vi "SentinelController v25.vi"() -> ()   [LabVIEW 2011]
uses:
  <userlib>/configTool/configTool.llb/loadConfigFile.vi
  <userlib>/configTool/configTool.llb/getProperty(STR).vi
  <userlib>/configTool/configTool.llb/initConfigGlobal.vi
  <userlib>/configTool/configTool.llb/closeConfig.vi
  <userlib>/configTool/configTool.llb/getProperty(DBL).vi
  <userlib>/configTool/configTool.llb/getProperty(I32).vi
  <userlib>/configTool/configTool.llb/getProperty(U32).vi
  <userlib>/configTool/configTool.llb/getProperty(BOOL).vi
  SC virtual tester states.ctl
  <vilib>/Instr/_visa.llb/Select Event Type.ctl
  SC virtual handler states.ctl
panel:
  in  "H2 sites ready hidden":string
  out "H2 wt start hidden":u32
  out "H2 wt end hidden":u32
  out "H2 it start hidden":u32
  out "H2 it end hidden":u32
  out "H2 tt start hidden":u32
  out "H2 tt end hidden":u32
  in  "Panels":T1(tab)=enum."System Configuration"
  in  "Test cell ID":string="default"
  in  "Operator name":string="default"
  in  "Lot number":string="default"
  in  "Configuration file path and filename":path
  in  "POWER":bool=TRUE
  in  "H2 allow lower parallelism":bool
  in  "H1 allow lower parallelism":bool
  in  "H1 low yield warning":dbl=95.0 min=0.0 max=100.0 step=1.0
  in  "Ignore alarms until AFTER this many cycles":i32=20
  in  "H1 low yield alarm":dbl=85.0 min=0.0 max=100.0 step=1.0
  in  "H1 low UPH warning (%)":dbl=95.0 min=1.0 max=48000.0 step=1.0
  in  "H1 low UPH alarm (%)":dbl=90.0 min=1.0 max=48000.0 step=1.0
  in  "Enable data logging of all events":bool=TRUE
  in  "Enable electronic notification of alarms":bool
  in  "H2 low UPH alarm (%)":dbl=90.0 min=1.0 max=48000.0 step=1.0
  in  "H2 low UPH warning (%)":dbl=95.0 min=1.0 max=48000.0 step=1.0
  in  "H2 low yield alarm":dbl=90.0 min=0.0 max=100.0 step=1.0
  in  "H2  low yield warning":dbl=95.0 min=0.0 max=100.0 step=1.0
  in  "H1 enable halt\non yield alarm":bool
  in  "H2 enable halt\non yield alarm":bool
  in  "H1 enable halt\non UPH alarm":bool
  in  "H2 enable halt\non UPH alarm":bool
  out "H2 Device Count":u32 caption="Device Count"
  out "H1 Device Count":u32 caption="Decvice Count"
  out "H1 Good Units":u32 caption="Decvice Count"
  out "H2 Good Units":u32 caption="Device Count"
  out "H1 lot yield mon":dbl format="%.1f"
  out "H2 lot yield mon":dbl format="%.1f"
  out "UPH averaging":u32=20 min=2 max=100 step=1
  out "Yield averaging":u32=20 min=2 max=100 step=1
  in  "Push to reset charts":bool
  in  "Run":bool caption="Run / Stop"
  in  "Optimize handler speed":bool
  out "H1 parallelism":u32
  out "Utilization averaging":i32=6 min=2 max=20 step=1
  out "H2 nominal 2":bool=TRUE
  out "H2 warning 2":bool
  out "H2 alarm 2":bool
  out "H1 nominal 2":bool=TRUE
  out "H1 warning 2":bool
  out "H1 alarm 2":bool
  out "H2 nominal":bool=TRUE
  out "H2 warning":bool
  out "H2 alarm":bool
  out "H1 nominal":bool=TRUE
  out "H1 warning":bool
  out "H1 alarm":bool
  out "H2 Lock":bool
  out "H1 Lock":bool
  out "H2 measured Test Time":dbl caption="Index Time" format="%.2f"
  out "H2 measured  Index Time":dbl caption="Index Time" format="%.2f"
  out "H2 Indexing":bool
  out "H2 Testing":bool
  out "H2 Ready with sites":bool
  out "H2 On/Off-line":bool
  out "H2 measured Wait Time":dbl caption="Index Time" format="%.2f"
  out "H1 measured Test Time":dbl caption="Index Time" format="%.2f"
  out "H1 measured Index Time":dbl caption="Index Time" format="%.2f"
  out "H1 Indexing":bool
  out "H1 Testing":bool
  out "H1 Ready with sites":bool
  out "H1 On/Off-line":bool
  out "H1 measured Wait Time":dbl caption="Index Time" format="%.2f"
  out "System UPH":u32(knob) caption="Sys UPH" scale=0.0..30240.0 scale format="%#.0f"
  out "H2 UPH":cluster{u32, u32}(knob) scale=0.0..14400.0 scale format="%#.0f"
  out "H1 UPH":cluster{u32, u32}(knob) scale=0.0..14400.0 scale format="%#.0f"
  out "Sys utilization":dbl(knob) caption="Yield" scale=0.0..100.0
  in  "H2 online":bool=TRUE
  in  "H1 online":bool=TRUE
  in  "Tester online":bool=TRUE
  in  "Alert volume":u32(knob)=5 max=10 step=1 scale=0.0..10.0
  in  "Audio On / Off":bool
  out "SysUtilMon":cluster{i32, i32}(graph)
  out "H2 parallelism":u32 caption="H2 Paralellism"
  out "YieldMon":cluster{i32, i32, i32, i32}(graph)
  out "Program Parallelism":u32=8 caption="Tester Parallelism" min=1 max=16 step=1
  out "H2 calc UPH":dbl format="%#.0f"
  out "H1 Index Time 2":dbl caption="H1 index time"
  out "H1 Test Time 2":dbl caption="H1 test time"
  out "H1 P in formula":u32 caption="H1 Parallelism"
  out "H2 UPH per unit area":dbl format="%.1f"
  out "H1 calc UPH":dbl format="%#.0f"
  out "H1 UPH per unit area":dbl format="%.1f"
  out "Std mo cost ($/mo)":dbl
  out "Std unit cost\n(cents/device)":dbl format="%.3g"
  out "UPH":dbl format="%#.0f"
  in  "Hours per month":i32=730
  out "Std hourly\ncost ($/hr)":dbl format="%.2f"
  in  "Std cell \nfloorspace area":i32=200 min=10 max=1000 step=10
  in  "Overhead ($/mo)":dbl=1000.0 min=0.0 max=10000.0 step=100.0
  in  "Handler cost ($/mo)":dbl=2500.0 min=0.0 max=100000.0 step=100.0
  in  "Tester cost ($/mo)":dbl=8500.0 min=0.0 max=100000.0 step=500.0
  in  "Utilization (%)":u32=80 min=10 max=100 step=10
  out "Calendar days required\nfor testing all units":dbl format="%.1f"
  in  "# of devices to test":u32=10000000 min=1000 max=100000000 step=1000
  out "$ saved":i64 format="%#.0f"
  out "H2 IT (scycle)":dbl format="%.2f"
  out "H2 TT (s/cycle)":dbl format="%.2f"
  out "H2 WT (s/cycle)":dbl format="%.2f"
  out "H1 WT (s/cycle)":dbl format="%.2f"
  out "H1 IT (s/cycle)":dbl format="%.2f"
  out "H1 TT (s/cycle)":dbl format="%.2f"
  out "H2 units/cycle":u32 caption="H1 Parallelism"
  out "H1 units/cycle":u32
  out "Calc H1 UPH":u32
  out "Calc H2 UPH":u32
  out "Std cell floorspace area":i32
  out "Tandem unit cost\n(cents/device)":dbl format="%.3f"
  out "Hours per month 2":i32 caption="Hours per month"
  out "Total Mo Costs ($/mo) 3":dbl caption="Tandem mo cost ($/mo)"
  out "Total Mo Costs ($/mo) 2":dbl caption="Std mo cost ($/mo)"
  out "Calc\nsystem UPH":u32 caption="Simulated\nSystem UPH"
  out "Tandem\nfloorspace area":i32
  out "Tandem UPH\nper unit area":dbl format="%.1f"
  in  "Second handler cost ($/mo)":dbl=2500.0 min=0.0 max=10000.0 step=100.0
  out "Tandem hourly\ncost ($/hr)":dbl format="%.2f"
  in  "Celerint licensing cost ($/mo)":dbl=1000.0 min=0.0 max=10000.0 step=100.0
  in  "Celerint hardware cost ($/mo)":dbl min=0.0 max=10000.0 step=1.0
  in  "Additional floorspace\nfor second handler":i32=50 min=0 max=1000 step=10
  out "Number of text alerts":u32 caption="Number of alerts\nsent as notifications"
  in  "Enable text notification":bool
  out "Notifications Lot Display":string="default" caption="Lot number (not editable)"
  in  "Include\ndata log as\nattachment":bool=TRUE
  out "Number of email alerts":u32 caption="Number of alerts\nsent as notifications"
  out "Email alert - attachment (not editable)":path
  in  "Email alert - message":string="An alarm event has ocurred on a semiconductor test lot that you have requested to monitor.  Please see the attached data log for event details.\n\nThis message is generated automatically by the Sentinel Controller program.\n\nTo stop these messages, please contact the test floor operator and disable automatic alert notifictions.\n\n"
  in  "Email alert - engineer":string="harry@celerint.com"
  in  "Email alert - CC":string="hjr@celerint.com"
  in  "Enable email notification":bool
  in  "Carrier":enum16{"T-Mobile", "AT&T", "Verizon", "Sprint"}(ring)=enum."AT&T"
  in  "Phone number":string="5128263411"
  in  "Subject":string="From: Sentinel Controller"
  in  "Body":string="An alarm event has ocurred"
  in  "GPIB wait time (ms)":u32=1000
  in  "Slow for  Diagnostics":bool
  out "GPIB bus 0 read error":bool
  out "GPIB Bus 0 traffic":string
  out "GPIB bus 1 traffic":string
  out "GPIB bus 2 traffic":string
  out "GPIB bus 0 write error":bool
  out "GPIB bus 1 read error":bool
  out "GPIB bus 1 write error":bool
  out "GPIB bus 2 write error":bool
  out "GPIB bus 2 read error":bool
  out "VISA bus 1 open error":bool
  out "VISA bus 2 open error":bool
  out "VISA bus 0 open error":bool
  out "VISA bus 0 close error":bool
  out "VISA bus 1 close error":bool
  out "VISA bus 2 close error":bool
  out "Decrease Handler Velocity":string
  out "Increase Handler Velocity":string
  out "Get Handler Velocity":string
  in  "SentCtrl listens to tester at":refnum<visa-resource-name>="GPIB0::INTFC"
  out "H2 Address":string
  out "H1 Address":string
  out "Tester address":string
  in  "SentCtrl talks to tester at":refnum<visa-resource-name>="GPIB0::0::INSTR"
  in  "SentCtrl listens to handler 1 at":refnum<visa-resource-name>="GPIB1::INTFC"
  in  "SentCtrl talks to handler 1 at":refnum<visa-resource-name>="GPIB1::1::INSTR"
  in  "SentCtrl listens to handler 2 at":refnum<visa-resource-name>="GPIB2::INTFC"
  in  "SentCtrl talks to handler 2 at":refnum<visa-resource-name>="GPIB2::1::INSTR"
  in  "Ni Logo":bool
  in  "Ni Logo 2":bool
  in  "GPIB wait timeout hid":u32
  out "Number of data log entries hid":u32
  in  "Last locked handler":enum16{"H1", "H2"}(ring)
  out "SC measured wait time hid":dbl
  out "Exit virtual tester H2 state machine hid":bool
  out "Exit virtual tester H1 state machine hid":bool
  out "Exit virtual handler state machine hid":bool
  out "H2 response to *HAND? hidden":string
  out "H1 response to *HAND? hidden":string
  in  "SC virtual tester 2 states":T2
  in  "Tester loop counterhid":u32
  in  "H2 loop counter hid":u32
  in  "H1 loop counter hid":u32
  in  "Test Cycle State hid":T3(ring)
  in  "Test time expected hid":dbl
  out "H1 it end hidden":u32
  out "H1 wt start hidden":u32
  out "H1 tt start hidden":u32
  out "H1 wt end hidden":u32
  out "H1 tt end hidden":u32
  out "H1 it start hidden":u32
  in  "SC virtual tester 1 states":T2
  in  "H1 sites ready hidden":string
  out "VISA bus 1 resource name out":refnum<visa-resource-name>
  out "VISA bus 1 error out":errorcluster
  out "VISA bus 2 error out":errorcluster
  out "VISA bus 2 resource name out":refnum<visa-resource-name>
  out "VISA bus 0 error out":errorcluster
  out "tester wt start hidden":u32
  out "tester wt end hidden":u32
  out "tester tt start hidden":u32
  out "tester tt end hidden":u32
  out "SC measured test time hid":dbl
  in  "Binning_string hidden":string
  out "VISA bus 0 resource name out":refnum<visa-resource-name>
  in  "SC virtual handler states":T4
  out "H1 Single Handler UPH hid":dbl
  out "H1 UPH warning limit hid":dbl
  out "H1 UPH alarm limit hid":dbl
  out "H2 Single Handler UPH hid":dbl
  out "H2 UPH warning limit hid":dbl
  out "H2 UPH alarm limit hid":dbl
  in  "Min Test Time hid":dbl=0.499 caption="Min Test Time" min=0.1 max=1.0 step=0.1 format="%#.1g"
  in  "H2 index time expected hid":dbl
  in  "H1 index time expected hid":dbl
  in  "system states hid":T5(ring)
  in  "system statuts hid":T6(ring)
  out "H1 cycle yield hid":dbl format="%.1f"
  out "H2 cycle yield hid":dbl format="%.1f"
  in  "Data log path and filename":path=path "configuraitons/default_configuraiton.cfg"
  # "Sentinel Controller\nfor\nTandlem Handler\nTest Cells \nwww.celerint.com"
  # "Turning off POWER will stop execution the Sentinel Controller Program"
  # "INPUT FILE"
  # "LOT INFORMATION"
  # "Celerint Sentinel Controller"
  # "SYSTEM PERFORMANCE THRESHOLDS"
  # "Handler  1"
  # "Handler 2"
  # "Set UPH thresholds as % of max UPH"
  # "Set UPH thresholds as % of max UPH"
  # "test cycles (insertions)"
  # "Celerint Sentinel Controller"
  # "Handler 2"
  # "Handler 1"
  # "Yield"
  # "UPH"
  # "Yield"
  # "UPH"
  # "parallelism"
  # "lot yield (%)"
  # "good devices"
  # "devices tested"
  # "Data"
  # "Avg"
  # "wait time"
  # "index time"
  # "test time"
  # "waiting"
  # "H1"
  # "H2"
  # "testing"
  # "indexing"
  # "on/off-line"
  # "STANDARD SETUP"
  # "H2 calculated\nsimilarly"
  # "3600"
  # "Celerint Sentinel\nController Simulator"
  # "TANDEM HANDLER SETUP"
  # "SAVINGS"
  # "3600 (s/hr)"
  # "3600 (s/hr)"
  # "Celerint Sentinel Controller"
  # "Lot number will be appended automatically:"
  # "This data is read from the INI file (.cfg)\nat program start and is used to configure\nthe various GPIB interfaces on the Sentinel\nController."
  # "These setting are created based on the addresses read from the INI file."
  # "Laptop Tester Sim\nGPIB0,SC\naddress 0\nlisten at: GPIB0::INTFC\ntalk to: GPIB0::1::INSTR"
  # "*SITES?"
  # "binning"
  # "Bus 0"
  # "1011"
  # "SC\nGPIB0,Non-SC\naddress 1\nlisten at: GPIB0::INTFC\ntalk to: GPIB0::0::INSTR"
  # "SC\nGPIB1,SC\naddress 0\nlisten at: GPIB1::INTFC\ntalk to: GPIB1::0::INSTR"
  # "SC\nGPIB2,SC\naddress 0\nlisten at: GPIB2::INTFC\ntalk to: GPIB2::0::INSTR"
  # "NI PXI-1031"
  # "*SITES?"
  # "binning"
  # "*SITES?"
  # "binning"
  # "Bus 1"
  # "Bus 2"
  # "1011"
  # "1011"
  # "Laptop H1 Sim\nGPIB1,Non-SC\naddress 1\nlisten at: GPIB1::INTFC\ntalk to: GPIB1::0::INSTR"
  # "Laptop H2 Sim\nGPIB2,Non-SC\naddress 1\nlisten at: GPIB2::INTFC\ntalk to: GPIB2::0::INSTR"
  # "Note:\nUsually, there are default GPIB addresses used for the tester and handler.\nThese addresses are read in from the INI file (.cfrg extension) when this\nprogram initializes.  For the purposes of this map, we are using  these defaults:\n          - Semiconductor tester default GPIB address: 6\n          - Semiconductor handler default GPIB address: 14\nFor the purposes of this illustration, these addresses are purely arbitrary."
  # "Tester\nGPIB0,SC\naddress 6\nlisten at: GPIB0::INTFC\ntalk to: GPIB0:14::INSTR"
  # "*SITES?"
  # "binning"
  # "Bus 0"
  # "1011"
  # "SC\nGPIB0,Non-SC\naddress 14\nlisten at: GPIB1::INTFC\ntalk to: GPIB1:6::INSTR"
  # "SC\nGPIB1,SC\naddress 6\nlisten at: GPIB1::INTFC\ntalk to: GPIB1:14::INSTR"
  # "SC\nGPIB2,SC\naddress 6\nlisten at: GPIB2::INTFC\ntalk to: GPIB2:14::INSTR"
  # "NI PXI-1031"
  # "*SITES?"
  # "binning"
  # "*SITES?"
  # "binning"
  # "Bus 1"
  # "Bus 2"
  # "1011"
  # "1011"
  # "Handler 1\nGPIB0,Non-SC\naddress 14\nlisten at: GPIB0::INTFC\ntalk to: GPIB0:6::INSTR"
  # "Handler 2\nGPIB0,Non-SC\naddress 14\nlisten at: GPIB0::INTFC\ntalk to: GPIB0:6::INSTR"
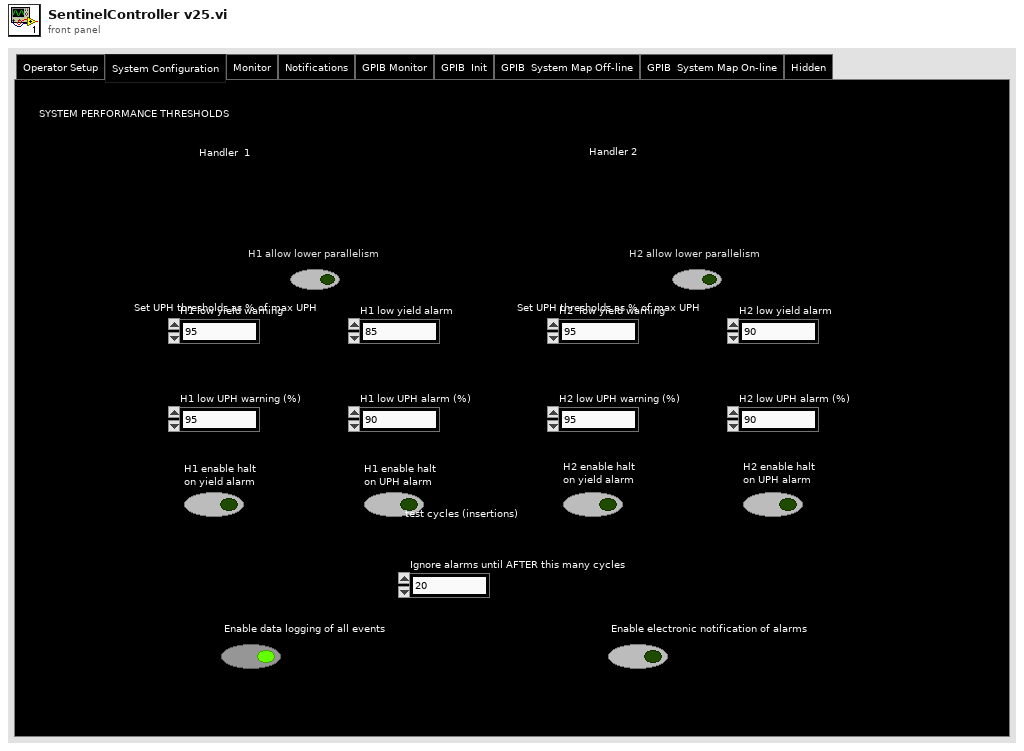
[diagram p1: front panel]
types:
  T1 = enum32{"Operator Setup", "System Configuration", "Monitor", "Benefit Analysis", "Notifications", "GPIB Monitor", "GPIB  Init", "GPIB  System Map Off-line", "GPIB  System Map On-line", "Hidden"}
  T2 = typedef "SC virtual tester states.ctl" = enum16{"initializing bus", "sending *IDN?", "polling SITES?", "sending HAND?", "sending HIDN?", "testing", "binning", "closing bus"}
  T3 = enum16{"idled", "SOT received", "SOT sent", "binning sent", "binning received", "sites ready received", "sites ready sent"}
  T4 = typedef "SC virtual handler states.ctl" = enum16{"initializing bus", "waiting on event", "reading", "responding to *IDN?", "responding to FR?", "responding to *STB?", "responding to *SITES?", "ressponding to FULLSITES?", "responding to *HIDN?", "respond to *HAND?", "testing", "responding to BINON", "responding to A BIN", "responding to ECHOOK", "responding to ECHONG", "indexing", "responding to unknown command", "closing bus"}
  T5 = enum16{"H1 Ready", "H2 Ready", "No Handler Ready"}
  T6 = enum16{"H1NH2N", "H1NH2W", "H1NH2A", "H1WH2N", "H1WH2W", "H1WH2A", "H1AH2N", "H1AH2W", "H1AH2A"}
  T7 = enum16{"open", "replace", "create", "open or create", "replace or create", "replace or create with confirmation"}
  T8 = typedef "configRef.ctl" = refnum<vi>
  T9 = cluster{i32, "rolling avg out":dbl, "H1 low yield alarm":dbl, "H2 low yield alarm":dbl}
  T10 = cluster{"rolling avg out":dbl, i32, "H1 low yield alarm":dbl, "H2 low yield alarm":dbl}
  T11 = typedef "Select Event Type.ctl" = u32
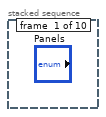
[diagram p2: hidden frame]
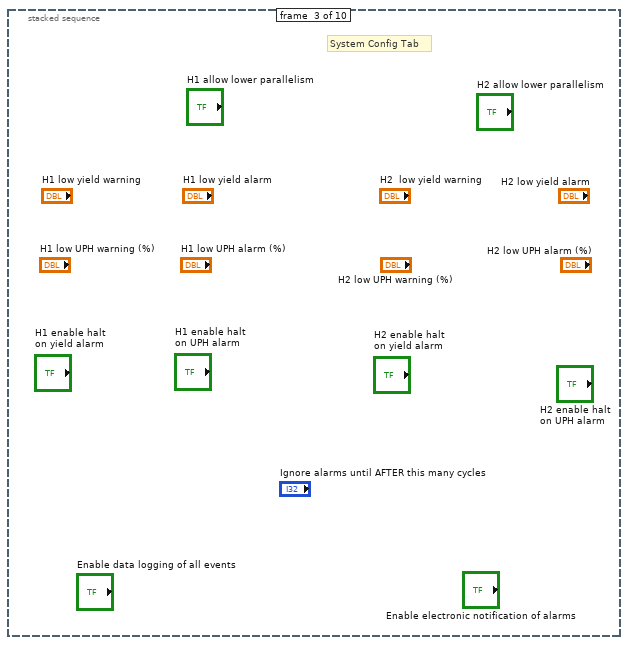
[diagram p3: hidden frame]
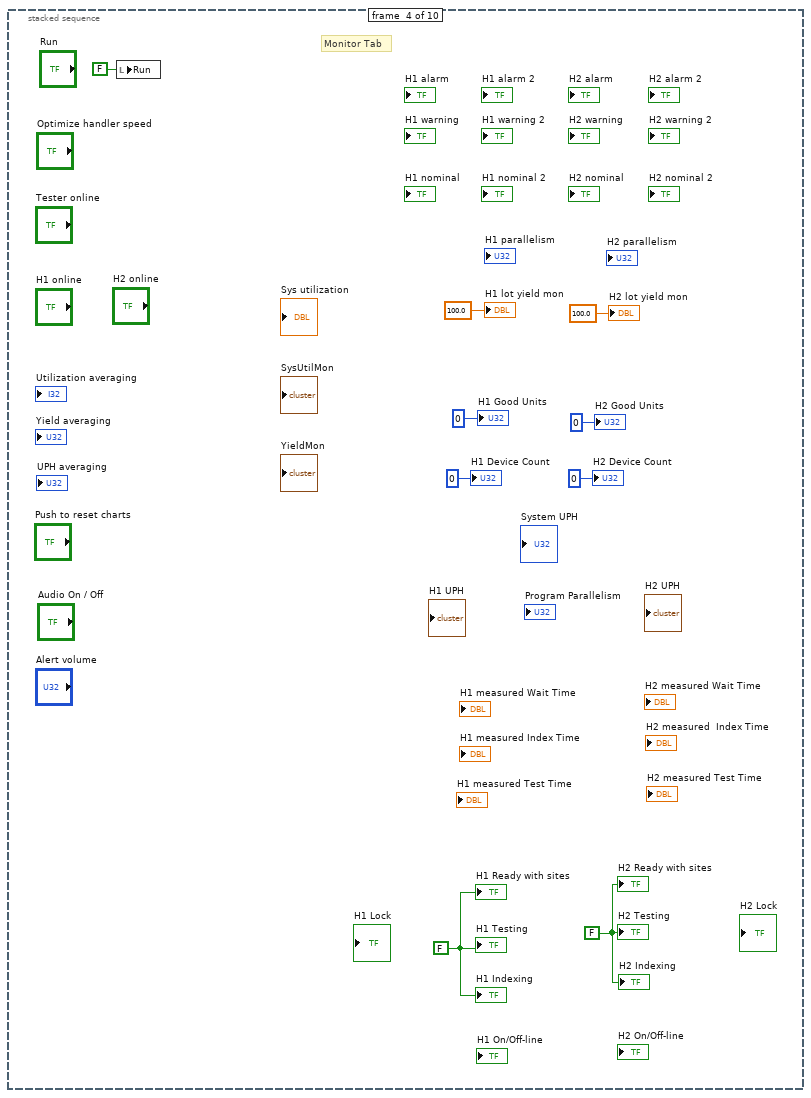
[diagram p4: hidden frame]
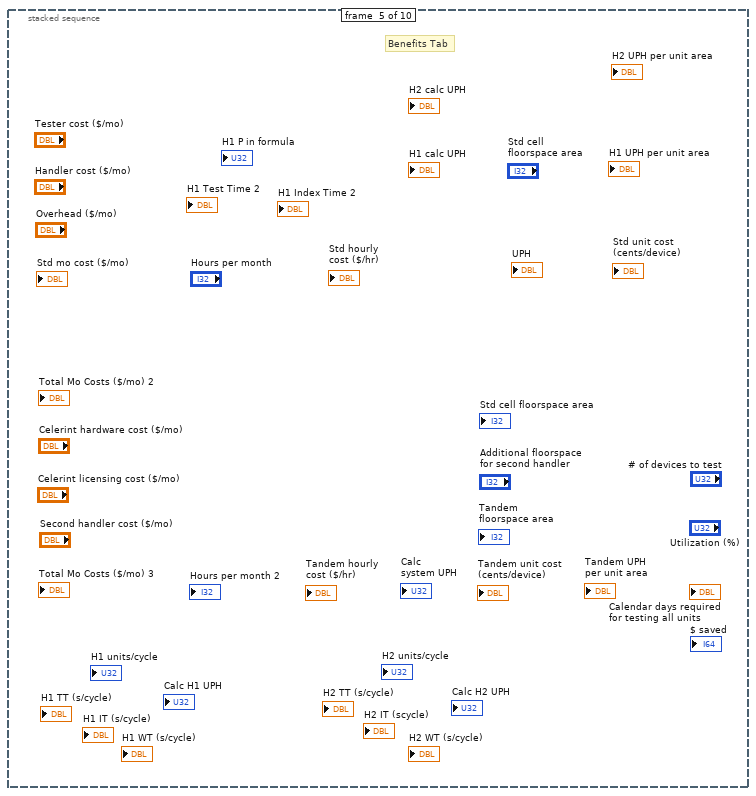
[diagram p5: hidden frame]
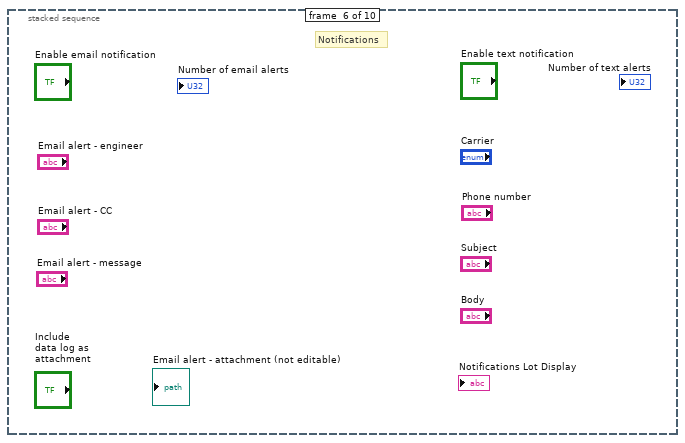
[diagram p6: hidden frame]
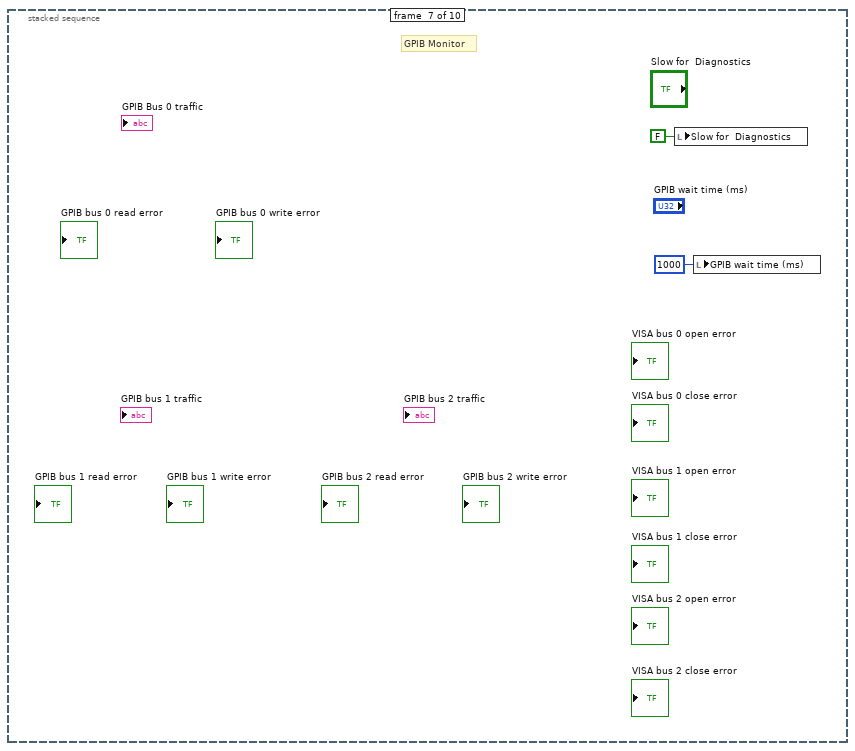
[diagram p7: hidden frame]
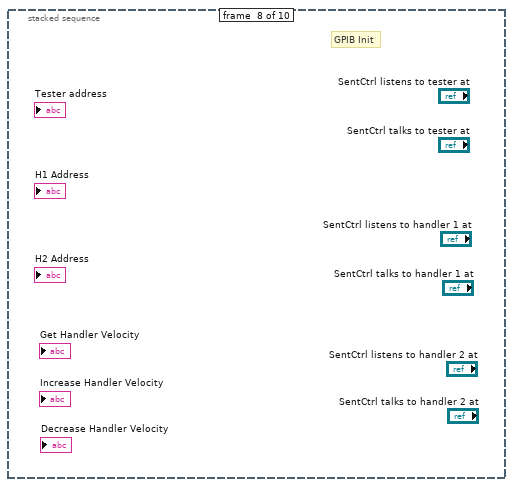
[diagram p8: hidden frame]
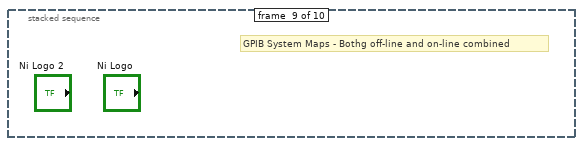
[diagram p9: hidden frame]
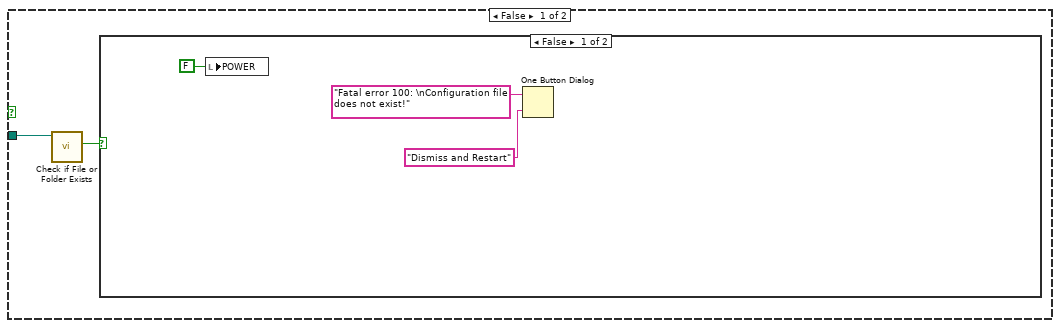
[diagram p11: hidden frame]
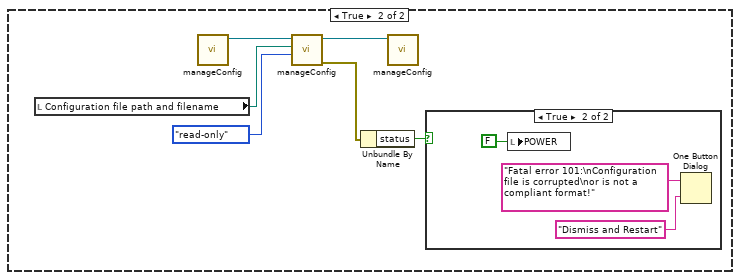
[diagram p12: hidden frame]
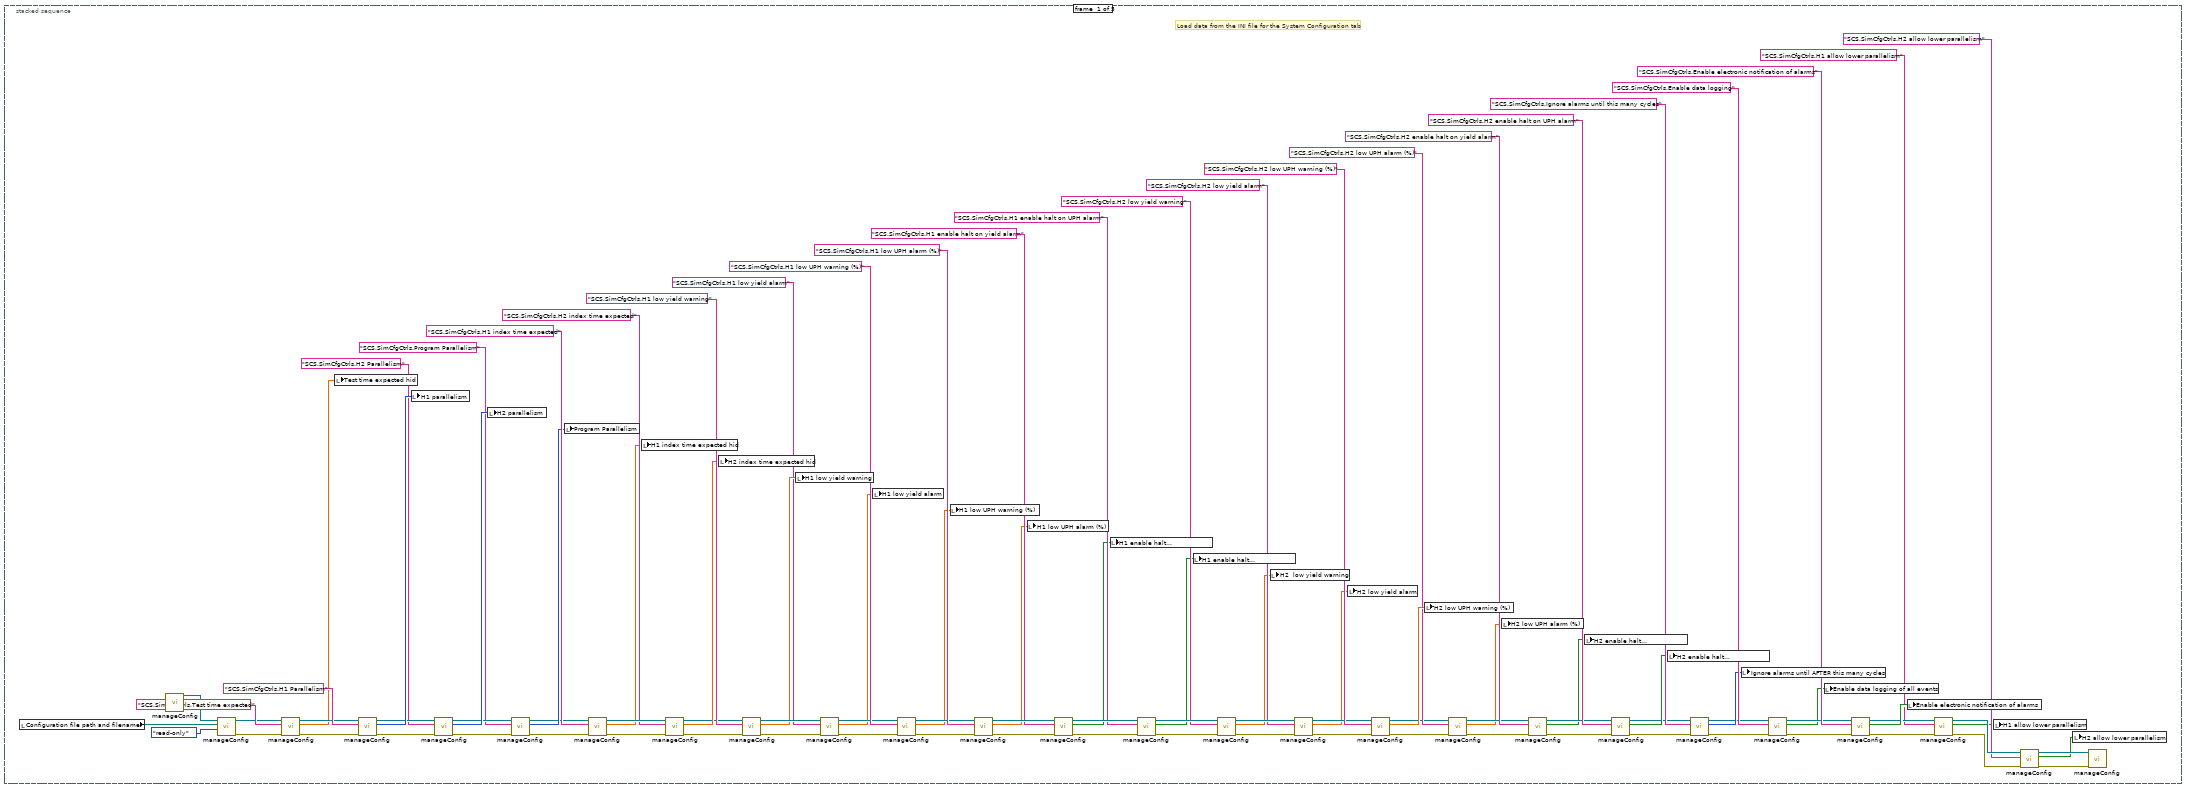
[diagram p15: hidden frame]
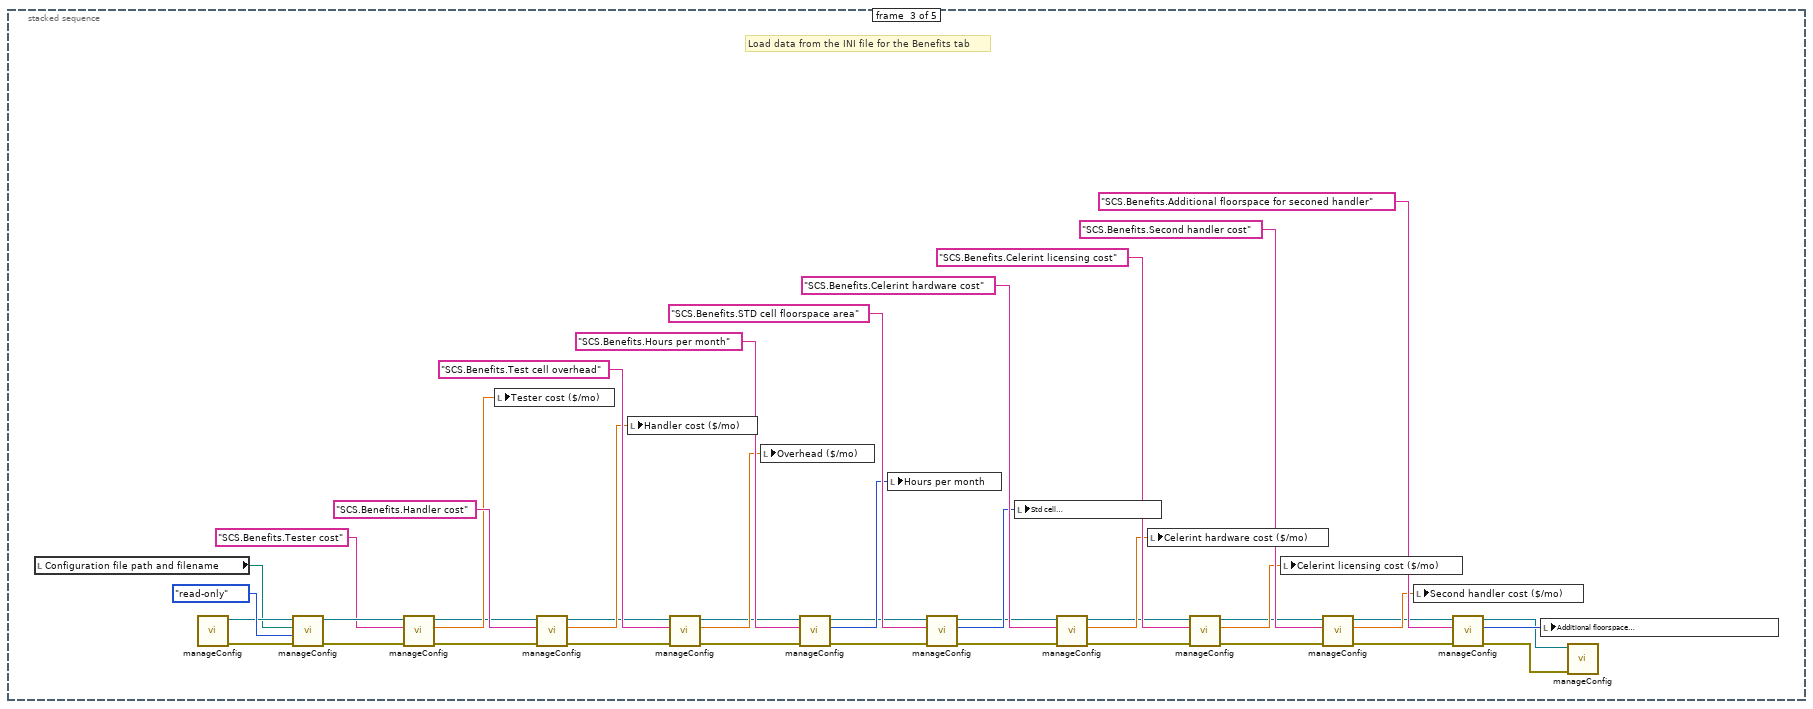
[diagram p16: hidden frame]
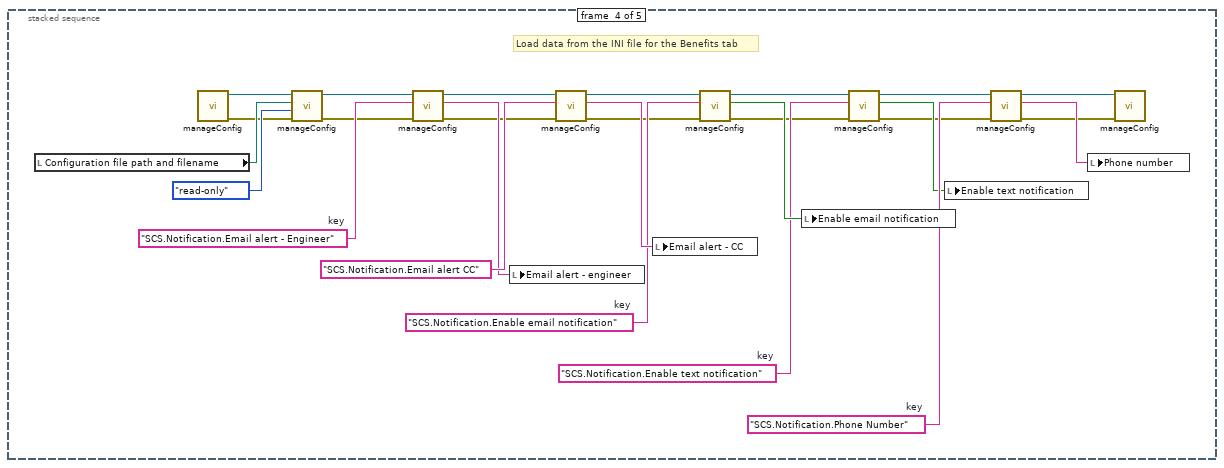
[diagram p17: hidden frame]
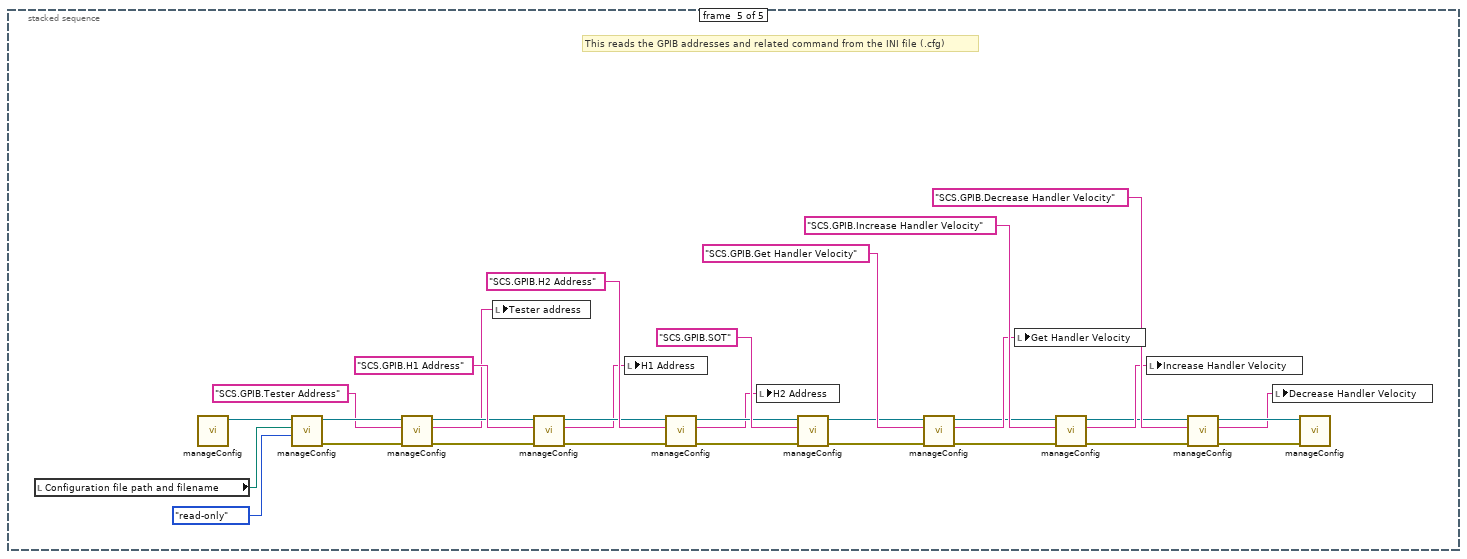
[diagram p18: hidden frame]
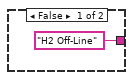
[diagram p20: hidden frame]
diagram:
  n1 = flat-sequence {
    frame #0 {
      # "This frame contains ALL declarations for control and indicators.\nAll hidden objects are on frame #9.  On the front panel, these hidden\nobjects are located on a tab that is hidden."
      n2 = stacked-sequence {
        frame #0 {
        }
        frame #1 {
          # "Operator Setup Tab"
        }
        frame #2 {
          # "System Config Tab"
        }
        frame #3 {
          w2 = FALSE ("H2 Testing")
          w1 = FALSE ("H1 Testing")
          # "Monitor Tab"
          n3 = local write "Run"(FALSE ("Run")) -> ()
          "H1 Testing" <- w1
          "H1 Ready with sites" <- w1
          "H1 Indexing" <- w1
          "H2 Testing" <- w2
          "H2 Ready with sites" <- w2
          "H2 Indexing" <- w2
          "H2 Good Units" <- 0
          "H2 Device Count" <- 0
          "H2 lot yield mon" <- 100.0 ("H2 Yield  Mon")
          "H1 lot yield mon" <- 100.0 ("H1 Yield Mon")
          "H1 Good Units" <- u32 0
          "H1 Device Count" <- u32 0
        }
        frame #4 {
          # "Benefits Tab"
        }
        frame #5 {
          # "Notifications"
        }
        frame #6 {
          # "GPIB Monitor"
          n4 = local write "Slow for  Diagnostics"(FALSE ("Slow for  Diagnostics")) -> ()
          n5 = local write "GPIB wait time (ms)"(u32 1000 ("GPIB wait time (ms)")) -> ()
        }
        frame #7 {
          # "GPIB Init"
        }
        frame #8 {
          # "GPIB System Maps - Bothg off-line and on-line combined"
        }
        frame #9 {
          (unwired) 0.031 ("tester measured wait time")
          # "Hidden controls and indicators"
          n6 = local write "Last locked handler"(enum16{"H1", "H2"}."H2" ("Last locked handler")) -> ()
          "SC measured test time hid" <- 1.0 ("tester measured test time")
          "H1 response to *HAND? hidden" <- "" ("H1 response to *HAND? hidden")
          "H2 response to *HAND? hidden" <- "" ("H2 response to *HAND? hidden")
          "Exit virtual handler state machine hid" <- FALSE ("Exit tester state machine")
          "Exit virtual tester H1 state machine hid" <- FALSE ("Exit H1 state machine")
          "Exit virtual tester H2 state machine hid" <- FALSE ("Exit H2 state machine")
          "SC measured wait time hid" <- 1.0 ("tester measured wait time hid")
          "H2 cycle yield hid" <- 100.0 ("H2 Yield  Mon")
          "H1 cycle yield hid" <- 100.0 ("H1 Yield Mon")
        }
      }
    }
    frame #1 {
      n7 = local write "POWER"(TRUE ("POWER")) -> ()
    }
    frame #2 {
      # "This frame handles verifying that the configuration file exists and is valaid.\nIt also creates the data log."
      n8 = local read "Configuration file path and filename"() -> (w25:path)
      n9 = call <vilib>:"Application Directory.vi"() -> ("Application Directory"=w27:path)
      n10 = Equal?(x=w25, y=path "") -> (x = y?=w24:bool)
      n11 = Get Date/Time String(want seconds? (F)=TRUE) -> (date string=w40:string, time string=w32:string)  [unwired: 2 in]
      n12 = Build Path(base path=w27, name or relative path="datalogs") -> (appended path=w45:path)
      n13 = Path To String(path=w45) -> (string=w36:string)
      n14 = Search and Replace String(replace all?=TRUE ("replace all? (F)"), input string=w40, search string="/", replace string="-" ("replace string (\"\")")) -> (result string=w30:string)  [unwired: 4 in, 3 out]
      n15 = Search and Replace String(replace all?=TRUE ("replace all? (F)"), input string=w32, search string=":", replace string="." ("replace string (\"\")")) -> (result string=w31:string)  [unwired: 4 in, 3 out]
      n16 = case shown="True" w24 {
        tunnel: w25 -> [w47 _]
        frame False {
          n17 = call <vilib>:"Check if File or Folder Exists.vi"("path"=w47) -> ("file or folder exists?"=w46:bool)  [unwired: 8 in, 2 out]
          n18 = case shown="False" w46 {
            frame False {
              n19 = local write "POWER"(FALSE ("POWER")) -> ()
              n20 = One Button Dialog(message="Fatal error 100: \nConfiguration file does not exist!", button name ("OK")="Dismiss and Restart") -> ()  [unwired: 1 out]
            }
            frame True {
              n21 = local read "Configuration file path and filename"() -> (w54:path)
              n22 = call-poly <userlib>:"manageConfig.vi"() -> ("config ref out"=w55:T8)  [unwired: 10 in, 1 out]
              n23 = call-poly <userlib>:"manageConfig.vi"("access (0:read/write)"=enum16{"read/write", "read-only", "write-only"}."read-only", "config file path"=w54, "config ref"=w55) -> ("error out"=w53:errorcluster, "config ref out"=w51:T8)  [unwired: 6 in, 1 out]
              n24 = Unbundle By Name(w53) -> ("status"=w52:bool)
              n25 = call-poly <userlib>:"manageConfig.vi"("config ref"=w51) -> ()  [unwired: 10 in, 1 out]
              n26 = case shown="True" w52 {
                frame False {
                }
                frame True {
                  n27 = local write "POWER"(FALSE ("POWER")) -> ()
                  n28 = One Button Dialog(message="Fatal error 101:\nConfiguration file is corrupted\nor is not a compliant format!", button name ("OK")="Dismiss and Restart") -> ()  [unwired: 1 out]
                }
              }
            }
          }
        }
        frame True {
          n29 = call <vilib>:"Application Directory.vi"() -> ("Application Directory"=w63:path)
          n30 = Build Path(base path=w63, name or relative path="configurations") -> (appended path=w60:path)
          n31 = Path To String(path=w60) -> (string=w65:string)
          n32 = Concatenate Strings(w65, "\\" ("string"), "default_configuration.cfg" ("string")) -> (w66:string)
          n33 = String To Path(string=w66) -> (path=w67:path)
          n34 = local write "Configuration file path and filename"(w67) -> ()
        }
      }
      n35 = Concatenate Strings(w36, "\\" ("string"), w30, " " ("string"), w31, ".txt" ("string")) -> (w42:string)
      n36 = String To Path(string=w42) -> (path=w44:path)
      n37 = local write "Data log path and filename"(w44) -> ()
    }
    frame #3 {
      # "This frame reads the INI file and initializes all data that is under engineering control."
      n38 = local read "POWER"() -> (w68:bool)
      n39 = case shown="True" w68 {
        frame False {
        }
        frame True {
          n40 = stacked-sequence {
            frame #0 {
              # "Load data from the INI file for the System Configuration tab"
              n41 = local read "Configuration file path and filename"() -> (w162:path)
              n42 = call-poly <userlib>:"manageConfig.vi"() -> ("config ref out"=w163:T8)  [unwired: 10 in, 1 out]
              n43 = call-poly <userlib>:"manageConfig.vi"("access (0:read/write)"=enum16{"read/write", "read-only", "write-only"}."read-only", "config file path"=w162, "config ref"=w163) -> ("error out"=w101:errorcluster, "config ref out"=w100:T8)  [unwired: 6 in, 1 out]
              n44 = call-poly <userlib>:"manageConfig.vi"("error in"=w101, "property path"="SCS.SimCfgCtrls.Test time expected" ("key"), "config ref"=w100) -> ("error out"=w97:errorcluster, "data"=w103:dbl, "config ref out"=w104:T8)  [unwired: 5 in, 1 out]
              n45 = local write "Test time expected hid"(w103) -> ()
              n46 = call-poly <userlib>:"manageConfig.vi"("error in"=w97, "property path"="SCS.SimCfgCtrls.H1 Parallelism", "config ref"=w104) -> ("error out"=w96:errorcluster, "value"=w116:u32, "config ref out"=w110:T8)  [unwired: 5 in, 1 out]
              n47 = local write "H1 parallelism"(w116) -> ()
              n48 = call-poly <userlib>:"manageConfig.vi"("error in"=w96, "property path"="SCS.SimCfgCtrls.H2 Parallelism", "config ref"=w110) -> ("error out"=w95:errorcluster, "value"=w112:u32, "config ref out"=w109:T8)  [unwired: 5 in, 1 out]
              n49 = local write "H2 parallelism"(w112) -> ()
              n50 = call-poly <userlib>:"manageConfig.vi"("error in"=w95, "property path"="SCS.SimCfgCtrls.Program Parallelism", "config ref"=w109) -> ("error out"=w94:errorcluster, "value"=w111:u32, "config ref out"=w102:T8)  [unwired: 5 in, 1 out]
              n51 = local write "Program Parallelism"(w111) -> ()
              n52 = call-poly <userlib>:"manageConfig.vi"("error in"=w94, "property path"="SCS.SimCfgCtrls.H1 index time expected", "config ref"=w102) -> ("error out"=w93:errorcluster, "data"=w106:dbl, "config ref out"=w115:T8)  [unwired: 5 in, 1 out]
              n53 = local write "H1 index time expected hid"(w106) -> ()
              n54 = call-poly <userlib>:"manageConfig.vi"("error in"=w93, "property path"="SCS.SimCfgCtrls.H2 index time expected", "config ref"=w115) -> ("error out"=w99:errorcluster, "data"=w105:dbl, "config ref out"=w98:T8)  [unwired: 5 in, 1 out]
              n55 = local write "H2 index time expected hid"(w105) -> ()
              n56 = call-poly <userlib>:"manageConfig.vi"("error in"=w99, "property path"="SCS.SimCfgCtrls.H1 low yield warning" ("key"), "config ref"=w98) -> ("error out"=w92:errorcluster, "data"=w139:dbl, "config ref out"=w149:T8)  [unwired: 5 in, 1 out]
              n57 = local write "H1 low yield warning"(w139) -> ()
              n58 = call-poly <userlib>:"manageConfig.vi"("error in"=w92, "property path"="SCS.SimCfgCtrls.H1 low yield alarm", "config ref"=w149) -> ("error out"=w91:errorcluster, "data"=w138:dbl, "config ref out"=w148:T8)  [unwired: 5 in, 1 out]
              n59 = local write "H1 low yield alarm"(w138) -> ()
              n60 = call-poly <userlib>:"manageConfig.vi"("error in"=w91, "property path"="SCS.SimCfgCtrls.H1 low UPH warning (%)", "config ref"=w148) -> ("error out"=w90:errorcluster, "data"=w137:dbl, "config ref out"=w150:T8)  [unwired: 5 in, 1 out]
              n61 = local write "H1 low UPH warning (%)"(w137) -> ()
              n62 = call-poly <userlib>:"manageConfig.vi"("error in"=w90, "property path"="SCS.SimCfgCtrls.H1 low UPH alarm (%)", "config ref"=w150) -> ("error out"=w89:errorcluster, "data"=w136:dbl, "config ref out"=w151:T8)  [unwired: 5 in, 1 out]
              n63 = local write "H1 low UPH alarm (%)"(w136) -> ()
              n64 = call-poly <userlib>:"manageConfig.vi"("error in"=w89, "property path"="SCS.SimCfgCtrls.H1 enable halt on yield alarm", "config ref"=w151) -> ("error out"=w88:errorcluster, "value"=w135:bool, "config ref out"=w152:T8)  [unwired: 5 in, 1 out]
              n65 = local write "H1 enable halt\non yield alarm"(w135) -> ()
              n66 = call-poly <userlib>:"manageConfig.vi"("error in"=w88, "property path"="SCS.SimCfgCtrls.H1 enable halt on UPH alarm", "config ref"=w152) -> ("error out"=w87:errorcluster, "value"=w134:bool, "config ref out"=w153:T8)  [unwired: 5 in, 1 out]
              n67 = local write "H1 enable halt\non UPH alarm"(w134) -> ()
              n68 = call-poly <userlib>:"manageConfig.vi"("error in"=w87, "property path"="SCS.SimCfgCtrls.H2 low yield warning", "config ref"=w153) -> ("error out"=w86:errorcluster, "data"=w133:dbl, "config ref out"=w154:T8)  [unwired: 5 in, 1 out]
              n69 = local write "H2  low yield warning"(w133) -> ()
              n70 = call-poly <userlib>:"manageConfig.vi"("error in"=w86, "property path"="SCS.SimCfgCtrls.H2 low yield alarm", "config ref"=w154) -> ("error out"=w85:errorcluster, "data"=w132:dbl, "config ref out"=w155:T8)  [unwired: 5 in, 1 out]
              n71 = local write "H2 low yield alarm"(w132) -> ()
              n72 = call-poly <userlib>:"manageConfig.vi"("error in"=w85, "property path"="SCS.SimCfgCtrls.H2 low UPH warning (%)", "config ref"=w155) -> ("error out"=w84:errorcluster, "data"=w131:dbl, "config ref out"=w123:T8)  [unwired: 5 in, 1 out]
              n73 = local write "H2 low UPH warning (%)"(w131) -> ()
              n74 = call-poly <userlib>:"manageConfig.vi"("error in"=w84, "property path"="SCS.SimCfgCtrls.H2 low UPH alarm (%)", "config ref"=w123) -> ("error out"=w83:errorcluster, "data"=w121:dbl, "config ref out"=w122:T8)  [unwired: 5 in, 1 out]
              n75 = local write "H2 low UPH alarm (%)"(w121) -> ()
              n76 = call-poly <userlib>:"manageConfig.vi"("error in"=w83, "property path"="SCS.SimCfgCtrls.H2 enable halt on yield alarm", "config ref"=w122) -> ("error out"=w82:errorcluster, "value"=w130:bool, "config ref out"=w156:T8)  [unwired: 5 in, 1 out]
              n77 = local write "H2 enable halt\non yield alarm"(w130) -> ()
              n78 = call-poly <userlib>:"manageConfig.vi"("error in"=w82, "property path"="SCS.SimCfgCtrls.H2 enable halt on UPH alarm", "config ref"=w156) -> ("error out"=w81:errorcluster, "value"=w129:bool, "config ref out"=w120:T8)  [unwired: 5 in, 1 out]
              n79 = local write "H2 enable halt\non UPH alarm"(w129) -> ()
              n80 = call-poly <userlib>:"manageConfig.vi"("error in"=w81, "property path"="SCS.SimCfgCtrls.Ignore alarms until this many cycles", "config ref"=w120) -> ("error out"=w80:errorcluster, "value"=w128:i32, "config ref out"=w119:T8)  [unwired: 5 in, 1 out]
              n81 = local write "Ignore alarms until AFTER this many cycles"(w128) -> ()
              n82 = call-poly <userlib>:"manageConfig.vi"("error in"=w80, "property path"="SCS.SimCfgCtrls.Enable data logging", "config ref"=w119) -> ("error out"=w79:errorcluster, "value"=w127:bool, "config ref out"=w140:T8)  [unwired: 5 in, 1 out]
              n83 = local write "Enable data logging of all events"(w127) -> ()
              n84 = call-poly <userlib>:"manageConfig.vi"("error in"=w79, "property path"="SCS.SimCfgCtrls.Enable electronic notification of alarms", "config ref"=w140) -> ("error out"=w78:errorcluster, "value"=w126:bool, "config ref out"=w76:T8)  [unwired: 5 in, 1 out]
              n85 = local write "Enable electronic notification of alarms"(w126) -> ()
              n86 = call-poly <userlib>:"manageConfig.vi"("error in"=w78, "property path"="SCS.SimCfgCtrls.H1 allow lower parallelism", "config ref"=w76) -> ("error out"=w77:errorcluster, "value"=w70:bool, "config ref out"=w75:T8)  [unwired: 5 in, 1 out]
              n87 = local write "H1 allow lower parallelism"(w70) -> ()
              n88 = call-poly <userlib>:"manageConfig.vi"("error in"=w77, "property path"="SCS.SimCfgCtrls.H2 allow lower parallelism", "config ref"=w75) -> ("error out"=w73:errorcluster, "value"=w69:bool, "config ref out"=w74:T8)  [unwired: 5 in, 1 out]
              n89 = local write "H2 allow lower parallelism"(w69) -> ()
              n90 = call-poly <userlib>:"manageConfig.vi"("error in (no error)"=w73, "config ref"=w74) -> ()  [unwired: 9 in, 1 out]
            }
            frame #1 {
              # "Load data from the INI file for the Monitor tab"
              n91 = local read "Configuration file path and filename"() -> (w201:path)
              n92 = call-poly <userlib>:"manageConfig.vi"() -> ("error out"=w175:errorcluster, "config ref out"=w202:T8)  [unwired: 10 in]
              n93 = call-poly <userlib>:"manageConfig.vi"("error in (no error)"=w175, "access (0:read/write)"=enum16{"read/write", "read-only", "write-only"}."read-only", "config file path"=w201, "config ref"=w202) -> ("error out"=w204:errorcluster, "config ref out"=w206:T8)  [unwired: 5 in, 1 out]
              n94 = call-poly <userlib>:"manageConfig.vi"("error in"=w204, "property path"="SCS.Monitor.Optimize handler speed" ("key"), "config ref"=w206) -> ("error out"=w174:errorcluster, "value"=w184:bool, "config ref out"=w176:T8)  [unwired: 5 in, 1 out]
              n95 = local write "Optimize handler speed"(w184) -> ()
              n96 = call-poly <userlib>:"manageConfig.vi"("error in"=w174, "property path"="SCS.Monitor.Tester on-line" ("key"), "config ref"=w176) -> ("error out"=w173:errorcluster, "value"=w183:bool, "config ref out"=w197:T8)  [unwired: 5 in, 1 out]
              n97 = local write "Tester online"(w183) -> ()
              n98 = call-poly <userlib>:"manageConfig.vi"("error in"=w173, "property path"="SCS.Monitor.H1 on-line" ("key"), "config ref"=w197) -> ("error out"=w172:errorcluster, "value"=w182:bool, "config ref out"=w196:T8)  [unwired: 5 in, 1 out]
              n99 = local write "H1 online"(w182) -> ()
              n100 = call-poly <userlib>:"manageConfig.vi"("error in"=w172, "property path"="SCS.Monitor.H2 on-line" ("key"), "config ref"=w196) -> ("error out"=w171:errorcluster, "value"=w181:bool, "config ref out"=w195:T8)  [unwired: 5 in, 1 out]
              n101 = local write "H2 online"(w181) -> ()
              n102 = call-poly <userlib>:"manageConfig.vi"("error in"=w171, "property path"="SCS.Monitor.Utilization averaging", "config ref"=w195) -> ("error out"=w170:errorcluster, "value"=w177:i32, "config ref out"=w194:T8)  [unwired: 5 in, 1 out]
              n103 = local write "Utilization averaging"(w177) -> ()
              n104 = call-poly <userlib>:"manageConfig.vi"("error in"=w170, "property path"="SCS.Monitor.Audio On/Off", "config ref"=w194) -> ("error out"=w169:errorcluster, "config ref out"=w193:T8)  [unwired: 5 in, 2 out]
              n105 = call-poly <userlib>:"manageConfig.vi"("error in"=w169, "property path"="SCS.Monitor.Alert volume", "config ref"=w193) -> ("error out"=w168:errorcluster, "value"=w180:u32, "config ref out"=w192:T8)  [unwired: 5 in, 1 out]
              n106 = local write "Alert volume"(w180) -> ()
              n107 = call-poly <userlib>:"manageConfig.vi"("error in"=w168, "property path"="SCS.Monitor.UPH averaging", "config ref"=w192) -> ("error out"=w167:errorcluster, "value"=w179:u32, "config ref out"=w191:T8)  [unwired: 5 in, 1 out]
              n108 = local write "UPH averaging"(w179) -> ()
              n109 = call-poly <userlib>:"manageConfig.vi"("error in"=w167, "property path"="SCS.Monitor.Yield averaging", "config ref"=w191) -> ("error out"=w166:errorcluster, "value"=w178:u32, "config ref out"=w190:T8)  [unwired: 5 in, 1 out]
              n110 = local write "Yield averaging"(w178) -> ()
              n111 = call-poly <userlib>:"manageConfig.vi"("error in (no error)"=w166, "config ref"=w190) -> ()  [unwired: 9 in, 1 out]
            }
            frame #2 {
              # "Load data from the INI file for the Benefits tab"
              n112 = local read "Configuration file path and filename"() -> (w243:path)
              n113 = call-poly <userlib>:"manageConfig.vi"() -> ("error out"=w216:errorcluster, "config ref out"=w244:T8)  [unwired: 10 in]
              n114 = call-poly <userlib>:"manageConfig.vi"("error in (no error)"=w216, "access (0:read/write)"=enum16{"read/write", "read-only", "write-only"}."read-only", "config file path"=w243, "config ref"=w244) -> ("error out"=w246:errorcluster, "config ref out"=w248:T8)  [unwired: 5 in, 1 out]
              n115 = call-poly <userlib>:"manageConfig.vi"("error in"=w246, "property path"="SCS.Benefits.Tester cost" ("key"), "config ref"=w248) -> ("error out"=w215:errorcluster, "data"=w234:dbl, "config ref out"=w225:T8)  [unwired: 5 in, 1 out]
              n116 = local write "Tester cost ($/mo)"(w234) -> ()
              n117 = call-poly <userlib>:"manageConfig.vi"("error in"=w215, "property path"="SCS.Benefits.Handler cost" ("key"), "config ref"=w225) -> ("error out"=w214:errorcluster, "data"=w233:dbl, "config ref out"=w224:T8)  [unwired: 5 in, 1 out]
              n118 = local write "Handler cost ($/mo)"(w233) -> ()
              n119 = call-poly <userlib>:"manageConfig.vi"("error in"=w214, "property path"="SCS.Benefits.Test cell overhead" ("key"), "config ref"=w224) -> ("error out"=w213:errorcluster, "data"=w232:dbl, "config ref out"=w223:T8)  [unwired: 5 in, 1 out]
              n120 = local write "Overhead ($/mo)"(w232) -> ()
              n121 = call-poly <userlib>:"manageConfig.vi"("error in"=w213, "property path"="SCS.Benefits.Hours per month" ("key"), "config ref"=w223) -> ("error out"=w212:errorcluster, "value"=w231:i32, "config ref out"=w222:T8)  [unwired: 5 in, 1 out]
              n122 = local write "Hours per month"(w231) -> ()
              n123 = call-poly <userlib>:"manageConfig.vi"("error in"=w212, "property path"="SCS.Benefits.STD cell floorspace area" ("key"), "config ref"=w222) -> ("error out"=w211:errorcluster, "value"=w230:i32, "config ref out"=w221:T8)  [unwired: 5 in, 1 out]
              n124 = local write "Std cell \nfloorspace area"(w230) -> ()
              n125 = call-poly <userlib>:"manageConfig.vi"("error in"=w211, "property path"="SCS.Benefits.Celerint hardware cost" ("key"), "config ref"=w221) -> ("error out"=w210:errorcluster, "data"=w229:dbl, "config ref out"=w220:T8)  [unwired: 5 in, 1 out]
              n126 = local write "Celerint hardware cost ($/mo)"(w229) -> ()
              n127 = call-poly <userlib>:"manageConfig.vi"("error in"=w210, "property path"="SCS.Benefits.Celerint licensing cost" ("key"), "config ref"=w220) -> ("error out"=w209:errorcluster, "data"=w228:dbl, "config ref out"=w219:T8)  [unwired: 5 in, 1 out]
              n128 = local write "Celerint licensing cost ($/mo)"(w228) -> ()
              n129 = call-poly <userlib>:"manageConfig.vi"("error in"=w209, "property path"="SCS.Benefits.Second handler cost" ("key"), "config ref"=w219) -> ("error out"=w208:errorcluster, "data"=w227:dbl, "config ref out"=w218:T8)  [unwired: 5 in, 1 out]
              n130 = local write "Second handler cost ($/mo)"(w227) -> ()
              n131 = call-poly <userlib>:"manageConfig.vi"("error in"=w208, "property path"="SCS.Benefits.Additional floorspace for seconed handler" ("key"), "config ref"=w218) -> ("error out"=w207:errorcluster, "value"=w226:i32, "config ref out"=w217:T8)  [unwired: 5 in, 1 out]
              n132 = local write "Additional floorspace\nfor second handler"(w226) -> ()
              n133 = call-poly <userlib>:"manageConfig.vi"("error in (no error)"=w207, "config ref"=w217) -> ()  [unwired: 9 in, 1 out]
            }
            frame #3 {
              w259 = "SCS.Notification.Enable text notification"  # key
              w265 = "SCS.Notification.Phone Number"  # key
              w266 = "SCS.Notification.Enable email notification"  # key
              w273 = "SCS.Notification.Email alert - Engineer"  # key
              # "Load data from the INI file for the Benefits tab"
              n134 = local read "Configuration file path and filename"() -> (w270:path)
              n135 = call-poly <userlib>:"manageConfig.vi"() -> ("error out"=w255:errorcluster, "config ref out"=w271:T8)  [unwired: 10 in]
              n136 = call-poly <userlib>:"manageConfig.vi"("error in (no error)"=w255, "access (0:read/write)"=enum16{"read/write", "read-only", "write-only"}."read-only", "config file path"=w270, "config ref"=w271) -> ("error out"=w254:errorcluster, "config ref out"=w274:T8)  [unwired: 5 in, 1 out]
              n137 = call-poly <userlib>:"manageConfig.vi"("error in"=w254, "property path"=w273, "config ref"=w274) -> ("error out"=w253:errorcluster, "value"=w268:string, "config ref out"=w264:T8)  [unwired: 5 in, 1 out]
              n138 = local write "Email alert - engineer"(w268) -> ()
              n139 = call-poly <userlib>:"manageConfig.vi"("error in"=w253, "property path"="SCS.Notification.Email alert CC", "config ref"=w264) -> ("error out"=w252:errorcluster, "value"=w267:string, "config ref out"=w263:T8)  [unwired: 5 in, 1 out]
              n140 = local write "Email alert - CC"(w267) -> ()
              n141 = call-poly <userlib>:"manageConfig.vi"("error in"=w252, "property path"=w266, "config ref"=w263) -> ("error out"=w251:errorcluster, "value"=w261:bool, "config ref out"=w258:T8)  [unwired: 5 in, 1 out]
              n142 = local write "Enable email notification"(w261) -> ()
              n143 = call-poly <userlib>:"manageConfig.vi"("error in"=w251, "property path"=w259, "config ref"=w258) -> ("error out"=w250:errorcluster, "value"=w256:bool, "config ref out"=w257:T8)  [unwired: 5 in, 1 out]
              n144 = local write "Enable text notification"(w256) -> ()
              n145 = call-poly <userlib>:"manageConfig.vi"("error in"=w250, "property path"=w265, "config ref"=w257) -> ("error out"=w249:errorcluster, "value"=w260:string, "config ref out"=w262:T8)  [unwired: 5 in, 1 out]
              n146 = local write "Phone number"(w260) -> ()
              n147 = call-poly <userlib>:"manageConfig.vi"("error in (no error)"=w249, "config ref"=w262) -> ()  [unwired: 9 in, 1 out]
            }
            frame #4 {
              # "This reads the GPIB addresses and related command from the INI file (.cfg)"
              n148 = local read "Configuration file path and filename"() -> (w301:path)
              n149 = call-poly <userlib>:"manageConfig.vi"() -> ("config ref out"=w302:T8)  [unwired: 10 in, 1 out]
              n150 = call-poly <userlib>:"manageConfig.vi"("access (0:read/write)"=enum16{"read/write", "read-only", "write-only"}."read-only", "config file path"=w301, "config ref"=w302) -> ("error out"=w304:errorcluster, "config ref out"=w306:T8)  [unwired: 6 in, 1 out]
              n151 = call-poly <userlib>:"manageConfig.vi"("error in"=w304, "property path"="SCS.GPIB.Tester Address" ("key"), "config ref"=w306) -> ("error out"=w291:errorcluster, "value"=w283:string, "config ref out"=w297:T8)  [unwired: 5 in, 1 out]
              n152 = local write "Tester address"(w283) -> ()
              n153 = call-poly <userlib>:"manageConfig.vi"("error in"=w291, "property path"="SCS.GPIB.H1 Address" ("key"), "config ref"=w297) -> ("error out"=w290:errorcluster, "value"=w282:string, "config ref out"=w296:T8)  [unwired: 5 in, 1 out]
              n154 = local write "H1 Address"(w282) -> ()
              n155 = call-poly <userlib>:"manageConfig.vi"("error in"=w290, "property path"="SCS.GPIB.H2 Address" ("key"), "config ref"=w296) -> ("error out"=w289:errorcluster, "value"=w281:string, "config ref out"=w295:T8)  [unwired: 5 in, 1 out]
              n156 = local write "H2 Address"(w281) -> ()
              n157 = call-poly <userlib>:"manageConfig.vi"("error in"=w289, "property path"="SCS.GPIB.SOT" ("key"), "config ref"=w295) -> ("error out"=w288:errorcluster, "config ref out"=w277:T8)  [unwired: 5 in, 2 out]
              n158 = call-poly <userlib>:"manageConfig.vi"("error in"=w288, "property path"="SCS.GPIB.Get Handler Velocity" ("key"), "config ref"=w277) -> ("error out"=w287:errorcluster, "value"=w280:string, "config ref out"=w276:T8)  [unwired: 5 in, 1 out]
              n159 = local write "Get Handler Velocity"(w280) -> ()
              n160 = call-poly <userlib>:"manageConfig.vi"("error in"=w287, "property path"="SCS.GPIB.Increase Handler Velocity" ("key"), "config ref"=w276) -> ("error out"=w286:errorcluster, "value"=w279:string, "config ref out"=w275:T8)  [unwired: 5 in, 1 out]
              n161 = local write "Increase Handler Velocity"(w279) -> ()
              n162 = call-poly <userlib>:"manageConfig.vi"("error in"=w286, "property path"="SCS.GPIB.Decrease Handler Velocity" ("key"), "config ref"=w275) -> ("error out"=w285:errorcluster, "value"=w278:string, "config ref out"=w284:T8)  [unwired: 5 in, 1 out]
              n163 = local write "Decrease Handler Velocity"(w278) -> ()
              n164 = call-poly <userlib>:"manageConfig.vi"("error in (no error)"=w285, "config ref"=w284) -> ()  [unwired: 9 in, 1 out]
            }
          }
        }
      }
    }
    frame #4 {
      # "This frame writes the headewr to the data log.\nIt includes setup and configuration information for the lot."
      n165 = local read "POWER"() -> (w307:bool)
      n166 = case shown="True" w307 {
        frame False {
        }
        frame True {
          w313 = "\r\n"
          n167 = local read "Lot number"() -> (w317:string)
          n168 = local read "Test cell ID"() -> (w315:string)
          n169 = local read "H1 online"() -> (w325:bool)
          n170 = local read "H2 online"() -> (w326:bool)
          n171 = local read "Data log path and filename"() -> (w308:path)
          n172 = local read "Operator name"() -> (w319:string)
          n173 = local read "H1 UPH warning limit hid"() -> (w321:dbl)
          n174 = local read "H2 UPH warning limit hid"() -> (w323:dbl)
          n175 = local read "H2  low yield warning"() -> (w322:dbl)
          n176 = local read "H1 low yield warning"() -> (w320:dbl)
          n177 = case shown="True" w325 {
            tunnel: ["H1 Off-Line" "H1 On-Line"] -> w327
            frame False {
            }
            frame True {
            }
          }
          n178 = case shown="True" w326 {
            tunnel: ["H2 Off-Line" "H2 On-Line"] -> w332
            frame False {
            }
            frame True {
            }
          }
          n179 = local write "Email alert - attachment (not editable)"(w308) -> ()
          n180 = Number To Decimal String(number=w320) -> (decimal integer string=w329:string)  [unwired: 1 in]
          n181 = Number To Decimal String(number=w321) -> (decimal integer string=w331:string)  [unwired: 1 in]
          n182 = Number To Decimal String(number=w322) -> (decimal integer string=w334:string)  [unwired: 1 in]
          n183 = Number To Decimal String(number=w323) -> (decimal integer string=w336:string)  [unwired: 1 in]
          n184 = Get Date/Time String() -> (date string=w310:string, time string=w312:string)  [unwired: 3 in]
          n185 = Concatenate Strings(w310, "   " ("string"), w312, w313, "Test Cell ID: ", w315, w313, "Lot Number: ", w317, w313, "Operator Name:  ", w319, w313, "System Started", w313, w327, w313, "H1 Low Yield Warning Limit: ", w329, w313, "H1 Low UPH Warning Limit: ", w331, w313, w332, w313, "H2 Low Yield Warning Limit: ", w334, w313, "H2 Low UPH Warning Limit: ", w336, w313, w313) -> (w337:string)
          n186 = call "SentinelDatalog.vi"("operation (0:open)"=T7."open or create", "String"=w337, "data log path"=w308) -> ()  [unwired: 8 in, 1 out]
        }
      }
    }
    frame #5 {
      # "This frame implements the main Sentinel Controller loop.\nAll loops within this frame execute as parallel processes."
      n187 = local read "POWER"() -> (w342:bool)
      n188 = case shown="True" w342 {
        frame False {
        }
        frame True {
          n189 = while {
            stop <- w357 stop-if-true
            w347 = 0
            w346 = 0.0
            w354 = 0
            w355 = 0.0
            # "Sentinel operating loop\n- tester loop\n- H1 loop\n- H2 loop\n- controls loop\n- alarm state machine loop\nExit with Power off"
            n190 = local read "POWER"() -> (w358:bool)
            n191 = Wait (ms)(milliseconds to wait=u32 100) -> ()  [unwired: 1 out]
            n192 = Not(x=w358) -> (.not. x?=w357:bool)
            n193 = while {
              i -> [w2333]
              stop <- w2349 stop-if-true
              n194 = local read "Run"() -> (w2325:bool)
              n195 = First Call?() -> (First Call?: T/F=w2326:bool)
              n196 = case shown="True" w2325 {
                frame False {
                  n197 = local write "Tester online"(FALSE ("Tester online")) -> ()
                  n198 = local write "H2 online"(FALSE ("H2 online")) -> ()
                  n199 = local write "H1 online"(FALSE ("H1 online")) -> ()
                }
                frame True {
                }
              }
              n200 = local read "Additional floorspace\nfor second handler"() -> (w2334:i32)
              n201 = Wait (ms)(milliseconds to wait=u32 50) -> ()  [unwired: 1 out]
              n202 = local read "Optimize handler speed"() -> (w2342:bool)
              n203 = local read "Std cell \nfloorspace area"() -> (w2347:i32)
              n204 = local read "Std cell \nfloorspace area"() -> (w2319:i32)
              n205 = local read "Celerint hardware cost ($/mo)"() -> (w2337:dbl)
              n206 = local read "Celerint licensing cost ($/mo)"() -> (w2336:dbl)
              n207 = local read "Second handler cost ($/mo)"() -> (w2335:dbl)
              n208 = case shown="True" w2326 {
                frame False {
                }
                frame True {
                  n209 = local read "H1 parallelism"() -> (w2382:u32)
                  n210 = local read "H2 parallelism"() -> (w2381:u32)
                  n211 = local read "H1 index time expected hid"() -> (w2380:dbl)
                  n212 = local read "H1 index time expected hid"() -> (w2390:dbl)
                  n213 = local read "H2 index time expected hid"() -> (w2379:dbl)
                  n214 = local read "H2 index time expected hid"() -> (w2391:dbl)
                  n215 = local read "Test time expected hid"() -> (w2388:dbl)
                  n216 = local write "H2 units/cycle"(w2381) -> ()
                  n217 = local write "H1 units/cycle"(w2382) -> ()
                  n218 = formula code="H1UPHorig=P1*3600/(T+H1ITorig);\nH2UPHorig=P2*3600/(T+H2ITorig);\nSYSH1WT=T-H1I;\nSYSH2WT=T-H2I;"("T"=w2388, "H1I"=w2380, "H2I"=w2379, "P1"=w2382, "H1ITorig"=w2390, "H2ITorig"=w2391, "P2"=w2381) -> ("H1UPHorig"=w2378:dbl, "H2UPHorig"=w2377:dbl, "SYSH1WT"=w2397:dbl, "SYSH2WT"=w2396:dbl)
                  n219 = local write "H1 Index Time 2"(w2380) -> ()
                  n220 = local write "H1 Test Time 2"(w2379) -> ()
                  n221 = local write "H1 P in formula"(w2382) -> ()
                  n222 = local write "H2 calc UPH"(w2377) -> ()
                  n223 = local read "H1 index time expected hid"() -> (w2384:dbl)
                  n224 = local read "H2 index time expected hid"() -> (w2383:dbl)
                  n225 = local read "Test time expected hid"() -> (w2385:dbl)
                  n226 = local write "H1 calc UPH"(w2378) -> ()
                  n227 = local write "UPH"(w2378) -> ()
                  n228 = local read "H2 parallelism"() -> (w2387:u32)
                  n229 = local read "H1 parallelism"() -> (w2386:u32)
                  n230 = Less Than 0?(x=w2397) -> (x < 0?=w2398:bool)
                  n231 = Less Than 0?(x=w2396) -> (x < 0?=w2399:bool)
                  n232 = Select(t=0.0, s=w2398, f=w2397) -> (s? t:f=w2393:dbl)
                  n233 = Select(t=0.0, s=w2399, f=w2396) -> (s? t:f=w2392:dbl)
                  n234 = local read "H1 index time expected hid"() -> (w2376:dbl)
                  n235 = local read "H2 index time expected hid"() -> (w2375:dbl)
                  n236 = local read "Test time expected hid"() -> (w2371:dbl)
                  n237 = formula code="ExpH1UPH=P1*3600/(T+SYSH1I+SYSH1WT);\nExpH2UPH=P2*3600/(T+SYSH2I+SYSH2WT);\nMaxUPH=Margin*(ExpH1UPH+ExpH2UPH);"("P1"=w2387, "T"=w2385, "SYSH1I"=w2384, "SYSH2I"=w2383, "Margin"=1.05 ("input variable"), "SYSH1WT"=w2393, "SYSH2WT"=w2392, "P2"=w2386) -> ("MaxUPH"=w2389:dbl, "ExpH1UPH"=w2395:dbl, "ExpH2UPH"=w2394:dbl)
                  n238 = Add(x=w2376, y=w2375) -> (x+y=w2374:dbl)
                  n239 = Divide(x=w2374, y=2.0) -> (x/y=w2372:dbl)
                  n240 = Add(x=w2371, y=w2372) -> (x+y=w2370:dbl)
                  n241 = Multiply(x=4000.0, y=w2370) -> (x*y=w2368:dbl)
                  n242 = To Unsigned Long Integer(number=w2368) -> (unsigned 32bit integer=w2367:u32)
                  n243 = local write "GPIB wait timeout hid"(w2367) -> ()
                  n244 = property on="System UPH" class="Knob (strict)"("Scale.Maximum"=w2389) -> ()  [unwired: 2 in, 2 out]
                  n245 = property on="H1 UPH" class="Knob (strict)"("Scale.Maximum"=w2395) -> ()  [unwired: 2 in, 2 out]
                  n246 = property on="H2 UPH" class="Knob (strict)"("Scale.Maximum"=w2394) -> ()  [unwired: 2 in, 2 out]
                }
              }
              n247 = local read "Handler cost ($/mo)"() -> (w2339:dbl)
              n248 = local read "Tester cost ($/mo)"() -> (w2340:dbl)
              n249 = local read "H1 online"() -> (w2329:bool)
              n250 = local read "H2 online"() -> (w2328:bool)
              n251 = local read "Overhead ($/mo)"() -> (w2338:dbl)
              n252 = local read "POWER"() -> (w2351:bool)
              n253 = Not(x=w2351) -> (.not. x?=w2350:bool)
              n254 = Not(x=w2329) -> (.not. x?=w2317:bool)
              n255 = Not(x=w2328) -> (.not. x?=w2316:bool)
              n256 = local read "Hours per month"() -> (w2321:i32)
              n257 = case shown="True" w2342 {
                frame False {
                }
                frame True {
                  # "place code here to optimize handler index times"
                }
              }
              n258 = local write "Std cell floorspace area"(w2319) -> ()
              n259 = Compound Arithmetic op=OR(w2350) -> (w2349:bool)
              n260 = And(x=w2317, y=w2316) -> (x .and. y?=w2327:bool)
              n261 = case shown="True" w2317 {
                frame False {
                }
                frame True {
                  n262 = local write "H1 nominal 2"(TRUE) -> ()
                  n263 = local write "H1 nominal"(TRUE) -> ()
                  n264 = local write "H1 warning 2"(TRUE) -> ()
                  n265 = local write "H1 warning"(TRUE) -> ()
                  n266 = local write "H1 alarm 2"(TRUE) -> ()
                  n267 = local write "H1 alarm"(TRUE) -> ()
                }
              }
              n268 = local write "H1 On/Off-line"(w2317) -> ()
              n269 = case shown="True" w2316 {
                frame False {
                }
                frame True {
                  n270 = local write "H2 nominal"(TRUE) -> ()
                  n271 = local write "H2 nominal 2"(TRUE) -> ()
                  n272 = local write "H2 warning"(TRUE) -> ()
                  n273 = local write "H2 warning 2"(TRUE) -> ()
                  n274 = local write "H2 alarm"(TRUE) -> ()
                  n275 = local write "H2 alarm 2"(TRUE) -> ()
                }
              }
              n276 = local write "H2 On/Off-line"(w2316) -> ()
              n277 = Add(x=w2334, y=w2347) -> (x+y=w2318:i32)
              n278 = Compound Arithmetic op=ADD(w2340, w2339, w2338) -> (w2344:dbl)
              n279 = Compound Arithmetic op=ADD(w2337, w2336, w2335) -> (w2345:dbl)
              n280 = Compound Arithmetic op=ADD(w2340, w2338) -> (w2322:dbl)
              n281 = case shown="False" w2327 {
                frame False {
                }
                frame True {
                  n282 = local write "System UPH"(u32 0 ("System UPH")) -> ()
                  n283 = local write "Sys utilization"(0.0 ("Sys utilization")) -> ()
                }
              }
              n284 = local write "Tandem\nfloorspace area"(w2318) -> ()
              n285 = Divide(x=w2345, y=w2321) -> (x/y=w2348:dbl)
              n286 = Add(x=w2345, y=w2344) -> (x+y=w2324:dbl)
              n287 = Divide(x=w2344, y=w2321) -> (x/y=w2320:dbl)
              n288 = local write "Hours per month 2"(w2321) -> ()
              n289 = local write "Total Mo Costs ($/mo) 2"(w2322) -> ()
              n290 = local write "Total Mo Costs ($/mo) 3"(w2324) -> ()
              n291 = local write "Std mo cost ($/mo)"(w2322) -> ()
              n292 = Add(x=w2320, y=w2348) -> (x+y=w2323:dbl)
              n293 = local write "Std hourly\ncost ($/hr)"(w2320) -> ()
              n294 = local read "Push to reset charts"() -> (w2331:bool)
              n295 = local write "Tandem hourly\ncost ($/hr)"(w2323) -> ()
              n296 = local read "Optimize handler speed"() -> (w2330:bool)
              n297 = case shown="True" w2331 {
                frame False {
                }
                frame True {
                  n298 = property on="YieldMon" class="WFChart (strict)"("History Data"=cluster{dbl, dbl, dbl, dbl}[] [{100.0, 100.0, 0.0, 0.0}]) -> ()  [unwired: 2 in, 2 out]
                  n299 = property on="SysUtilMon" class="WFChart (strict)"("History Data"=cluster{dbl, dbl}[] []) -> ()  [unwired: 2 in, 2 out]
                }
              }
              n300 = Equal To 0?(x=w2333) -> (x = 0?=w2332:bool)
              n301 = case shown="True" w2332 {
                frame False {
                }
                frame True {
                  w2424 = "" ("Message from tester")
                  w2427 = 0
                  w2430 = 0
                  w2443 = 100
                  w2444 = 0
                  w2445 = FALSE ("H1 alarm")
                  # "graphs and charts - declared here, displayed elsewhere"
                  n302 = Bundle(w2443, w2443, w2443, w2443) -> (w2422:cluster{i32, i32, i32, i32})  [unwired: 1 in]
                  n303 = Bundle(w2444, w2444) -> (w2421:cluster{i32, i32})  [unwired: 1 in]
                  n304 = local write "H2 Lock"(FALSE ("H2 Lock")) -> ()
                  n305 = local write "H1 alarm"(FALSE ("H1 warning")) -> ()
                  n306 = local write "H1 Lock"(FALSE ("H1 Lock")) -> ()
                  n307 = local write "H2 warning 2"(FALSE ("H1 warning")) -> ()
                  n308 = local write "H2 warning"(FALSE ("H1 warning")) -> ()
                  n309 = local write "H1 warning 2"(FALSE ("H1 warning")) -> ()
                  n310 = local write "H1 warning"(FALSE ("H1 warning")) -> ()
                  n311 = local write "H2 nominal 2"(TRUE ("H1 nominal")) -> ()
                  n312 = local write "H2 alarm 2"(FALSE ("H1 warning")) -> ()
                  n313 = local write "H2 alarm"(FALSE ("H1 warning")) -> ()
                  n314 = local write "H1 nominal 2"(TRUE ("H1 nominal")) -> ()
                  n315 = local write "H1 alarm 2"(FALSE ("H1 warning")) -> ()
                  n316 = local write "system statuts hid"(T6."H1NH2N" ("system statuts")) -> ()
                  n317 = local write "H1 Good Units"(w2430) -> ()
                  n318 = local write "H2 Device Count"(w2430) -> ()
                  n319 = local write "H2 Good Units"(w2430) -> ()
                  n320 = local write "H1 Device Count"(w2430) -> ()
                  n321 = property on="System UPH" class="Knob (strict)"("Scale.Minimum"=w2427) -> ()  [unwired: 2 in, 2 out]
                  n322 = property on="H1 UPH" class="Knob (strict)"("Scale.Minimum"=w2427) -> ()  [unwired: 2 in, 2 out]
                  n323 = property on="H2 UPH" class="Knob (strict)"("Scale.Minimum"=w2427) -> ()  [unwired: 2 in, 2 out]
                  n324 = property on="SysUtilMon" class="WFChart (strict)"("History Data"=cluster{dbl, dbl}[] []) -> ()  [unwired: 2 in, 2 out]
                  n325 = local write "H1 alarm"(w2445) -> ()
                  n326 = local write "H2 alarm"(w2445) -> ()
                  n327 = property on="YieldMon" class="WFChart (strict)"("History Data"=cluster{dbl, dbl, dbl, dbl}[] []) -> ()  [unwired: 2 in, 2 out]
                  n328 = local write "YieldMon"(w2422) -> ()
                  n329 = local write "SysUtilMon"(w2421) -> ()
                  n330 = local write "Sys utilization"(0.0) -> ()
                  n331 = local write "H2 alarm 2"(w2445) -> ()
                  n332 = local write "H1 alarm 2"(w2445) -> ()
                  n333 = local write "H2 nominal"(TRUE ("H1 nominal")) -> ()
                  n334 = local write "H1 nominal"(TRUE ("H1 nominal")) -> ()
                  n335 = local read "Lot number"() -> (w2419:string)
                  n336 = local write "Number of text alerts"(0.0 ("Number of Emails Alerts Sent")) -> ()
                  n337 = local write "Number of email alerts"(u32 0 ("Number of Emails Alerts Sent")) -> ()
                  n338 = local write "Tester loop counterhid"(u32 0 ("Tester loop counter")) -> ()
                  n339 = local write "H1 loop counter hid"(u32 0 ("H1 loop counter hid")) -> ()
                  n340 = local write "H2 loop counter hid"(u32 0 ("H2 loop counter hid")) -> ()
                  n341 = local write "GPIB Bus 0 traffic"(w2424) -> ()
                  n342 = local write "Notifications Lot Display"(w2419) -> ()
                  n343 = local write "GPIB bus 1 traffic"(w2424) -> ()
                  n344 = local write "GPIB bus 2 traffic"(w2424) -> ()
                }
              }
              n345 = case shown="True" w2330 {
                frame False {
                }
                frame True {
                  w2406 = FALSE
                  n346 = local read "H1 online"() -> (w2408:bool)
                  n347 = local read "H2 online"() -> (w2407:bool)
                  n348 = Equal?(x=w2408, y=w2406) -> (x = y?=w2410:bool)
                  n349 = Equal?(x=w2406, y=w2407) -> (x = y?=w2409:bool)
                  n350 = Or(x=w2410, y=w2409) -> (x .or. y?=w2405:bool)
                  n351 = case shown="True" w2405 {
                    frame False {
                    }
                    frame True {
                      n352 = local write "Optimize handler speed"(FALSE ("Optimize Handler Speed")) -> ()
                    }
                  }
                }
              }
              n353 = local read "Alert volume"() -> (w2341:u32)
              n354 = Equal To 0?(x=w2341) -> (x = 0?=w2343:bool)
              n355 = case shown="True" w2343 {
                frame False {
                }
                frame True {
                  n356 = local write "Audio On / Off"(FALSE ("Audio On/Off")) -> ()
                }
              }
            }
            n357 = case shown="True" FALSE {
              frame False {
              }
              frame True {
                n358 = while {
                  i -> [w398]
                  stop <- w411 stop-if-true
                  # "Play Audio Aert Loop"
                  n359 = local read "Ignore alarms until AFTER this many cycles"() -> (w403:i32)
                  n360 = local read "H1 Device Count"() -> (w408:u32)
                  n361 = local read "H2 Device Count"() -> (w407:u32)
                  n362 = local read "Program Parallelism"() -> (w405:u32)
                  n363 = local read "Run"() -> (w400:bool)
                  n364 = local read "POWER"() -> (w401:bool)
                  n365 = Add(x=w408, y=w407) -> (x+y=w406:u32)
                  n366 = Wait (ms)(milliseconds to wait=u32 100) -> ()  [unwired: 1 out]
                  n367 = Divide(x=w406, y=w405) -> (x/y=w404:dbl)
                  n368 = Greater?(x=w398, y=50) -> (0:w396:bool)
                  n369 = Greater?(x=w404, y=w403) -> (0:w402:bool)
                  n370 = Compound Arithmetic op=AND(w402, w401, w400, w396) -> (w399:bool)
                  n371 = case shown="True" w399 {
                    frame False {
                    }
                    frame True {
                      n372 = local read "system statuts hid"() -> (w415:T6)
                      n373 = case shown="\"H1AH2A\"" w415 {
                        frame "H1NH2N", Default {
                          n374 = Wait (ms)(milliseconds to wait=u32 50) -> ()  [unwired: 1 out]
                        }
                        frame "H1NH2W" {
                          n375 = flat-sequence {
                            frame #0 {
                              n376 = local read "Audio On / Off"() -> (w418:bool)
                              n377 = local read "H2 online"() -> (w417:bool)
                              n378 = And(x=w417, y=w418) -> (x .and. y?=w419:bool)
                              n379 = case shown="True" w419 {
                                frame False {
                                }
                                frame True {
                                n380 = local read "Run"() -> (w422:bool)
                                n381 = case shown="True" w422 {
                                tunnel: [0.001 w424] -> w421
                                frame False {
                                }
                                frame True {
                                n382 = local read "Alert volume"() -> (w424:u32)
                                }
                                }
                                n383 = call "PlayAlarm.vi"("wavefilename"="audio\\4_synth_warning.wav", "alertvolume"=w421) -> ()  [unwired: 10 in]
                                }
                              }
                            }
                            frame #1 {
                              n384 = local read "Run"() -> (w425:bool)
                              n385 = case shown="True" w425 {
                                frame False {
                                }
                                frame True {
                                n386 = Wait (ms)(milliseconds to wait=u32 5000) -> ()  [unwired: 1 out]
                                }
                              }
                            }
                          }
                        }
                        frame "H1NH2A" {
                          n387 = flat-sequence {
                            frame #0 {
                              n388 = local read "Audio On / Off"() -> (w429:bool)
                              n389 = local read "H2 online"() -> (w428:bool)
                              n390 = And(x=w428, y=w429) -> (x .and. y?=w427:bool)
                              n391 = case shown="True" w427 {
                                frame False {
                                }
                                frame True {
                                n392 = local read "Run"() -> (w432:bool)
                                n393 = case shown="True" w432 {
                                tunnel: [0.001 w434] -> w431
                                frame False {
                                }
                                frame True {
                                n394 = local read "Alert volume"() -> (w434:u32)
                                }
                                }
                                n395 = call "PlayAlarm.vi"("wavefilename"="audio\\bass_synth_alarm.wav", "alertvolume"=w431) -> ()  [unwired: 10 in]
                                }
                              }
                            }
                            frame #1 {
                              n396 = local read "Run"() -> (w435:bool)
                              n397 = case shown="True" w435 {
                                frame False {
                                n398 = Wait (ms)(milliseconds to wait=u32 50) -> ()  [unwired: 1 out]
                                }
                                frame True {
                                n399 = Wait (ms)(milliseconds to wait=u32 5000) -> ()  [unwired: 1 out]
                                }
                              }
                            }
                          }
                        }
                        frame "H1WH2N" {
                          n400 = flat-sequence {
                            frame #0 {
                              n401 = local read "Audio On / Off"() -> (w440:bool)
                              n402 = local read "H1 online"() -> (w439:bool)
                              n403 = And(x=w439, y=w440) -> (x .and. y?=w438:bool)
                              n404 = case shown="True" w438 {
                                frame False {
                                }
                                frame True {
                                n405 = local read "Run"() -> (w443:bool)
                                n406 = case shown="True" w443 {
                                tunnel: [0.001 w445] -> w442
                                frame False {
                                }
                                frame True {
                                n407 = local read "Alert volume"() -> (w445:u32)
                                }
                                }
                                n408 = call "PlayAlarm.vi"("wavefilename"="audio\\4_synth_warning.wav", "alertvolume"=w442) -> ()  [unwired: 10 in]
                                }
                              }
                            }
                            frame #1 {
                              n409 = local read "Run"() -> (w446:bool)
                              n410 = case shown="True" w446 {
                                frame False {
                                n411 = Wait (ms)(milliseconds to wait=u32 50) -> ()  [unwired: 1 out]
                                }
                                frame True {
                                n412 = Wait (ms)(milliseconds to wait=u32 5000) -> ()  [unwired: 1 out]
                                }
                              }
                            }
                          }
                        }
                        frame "H1WH2W" {
                          n413 = flat-sequence {
                            frame #0 {
                              n414 = local read "Audio On / Off"() -> (w452:bool)
                              n415 = local read "H1 online"() -> (w449:bool)
                              n416 = local read "H2 online"() -> (w451:bool)
                              n417 = Compound Arithmetic op=AND(w449, w451, w452) -> (w450:bool)
                              n418 = case shown="True" w450 {
                                frame False {
                                }
                                frame True {
                                n419 = local read "Run"() -> (w455:bool)
                                n420 = case shown="True" w455 {
                                tunnel: [0.001 w457] -> w454
                                frame False {
                                }
                                frame True {
                                n421 = local read "Alert volume"() -> (w457:u32)
                                }
                                }
                                n422 = call "PlayAlarm.vi"("wavefilename"="audio\\4_synth_warning.wav", "alertvolume"=w454) -> ()  [unwired: 10 in]
                                }
                              }
                            }
                            frame #1 {
                              n423 = local read "Run"() -> (w458:bool)
                              n424 = case shown="True" w458 {
                                frame False {
                                n425 = Wait (ms)(milliseconds to wait=u32 50) -> ()  [unwired: 1 out]
                                }
                                frame True {
                                n426 = Wait (ms)(milliseconds to wait=u32 5000) -> ()  [unwired: 1 out]
                                }
                              }
                            }
                          }
                        }
                        frame "H1WH2A" {
                          n427 = flat-sequence {
                            frame #0 {
                              n428 = local read "Audio On / Off"() -> (w464:bool)
                              n429 = local read "H1 online"() -> (w462:bool)
                              n430 = local read "H2 online"() -> (w463:bool)
                              n431 = Compound Arithmetic op=AND(w462, w463, w464) -> (w461:bool)
                              n432 = case shown="True" w461 {
                                frame False {
                                }
                                frame True {
                                n433 = local read "Run"() -> (w467:bool)
                                n434 = case shown="True" w467 {
                                tunnel: [0.001 w469] -> w466
                                frame False {
                                }
                                frame True {
                                n435 = local read "Alert volume"() -> (w469:u32)
                                }
                                }
                                n436 = call "PlayAlarm.vi"("wavefilename"="audio\\bass_synth_alarm.wav", "alertvolume"=w466) -> ()  [unwired: 10 in]
                                }
                              }
                            }
                            frame #1 {
                              n437 = local read "Run"() -> (w470:bool)
                              n438 = case shown="True" w470 {
                                frame False {
                                n439 = Wait (ms)(milliseconds to wait=u32 50) -> ()  [unwired: 1 out]
                                }
                                frame True {
                                n440 = Wait (ms)(milliseconds to wait=u32 5000) -> ()  [unwired: 1 out]
                                }
                              }
                            }
                          }
                        }
                        frame "H1AH2N" {
                          n441 = flat-sequence {
                            frame #0 {
                              n442 = local read "Audio On / Off"() -> (w475:bool)
                              n443 = local read "H1 online"() -> (w473:bool)
                              n444 = And(x=w473, y=w475) -> (x .and. y?=w474:bool)
                              n445 = case shown="True" w474 {
                                frame False {
                                }
                                frame True {
                                n446 = local read "Run"() -> (w478:bool)
                                n447 = case shown="True" w478 {
                                tunnel: [0.001 w480] -> w477
                                frame False {
                                }
                                frame True {
                                n448 = local read "Alert volume"() -> (w480:u32)
                                }
                                }
                                n449 = call "PlayAlarm.vi"("wavefilename"="audio\\bass_synth_alarm.wav", "alertvolume"=w477) -> ()  [unwired: 10 in]
                                }
                              }
                            }
                            frame #1 {
                              n450 = local read "Run"() -> (w481:bool)
                              n451 = case shown="True" w481 {
                                frame False {
                                n452 = Wait (ms)(milliseconds to wait=u32 50) -> ()  [unwired: 1 out]
                                }
                                frame True {
                                n453 = Wait (ms)(milliseconds to wait=u32 5000) -> ()  [unwired: 1 out]
                                }
                              }
                            }
                          }
                        }
                        frame "H1AH2W" {
                          n454 = flat-sequence {
                            frame #0 {
                              n455 = local read "Audio On / Off"() -> (w487:bool)
                              n456 = local read "H1 online"() -> (w485:bool)
                              n457 = local read "H2 online"() -> (w486:bool)
                              n458 = Compound Arithmetic op=AND(w485, w486, w487) -> (w484:bool)
                              n459 = case shown="True" w484 {
                                frame False {
                                }
                                frame True {
                                n460 = local read "Run"() -> (w490:bool)
                                n461 = case shown="True" w490 {
                                tunnel: [0.001 w492] -> w489
                                frame False {
                                }
                                frame True {
                                n462 = local read "Alert volume"() -> (w492:u32)
                                }
                                }
                                n463 = call "PlayAlarm.vi"("wavefilename"="audio\\bass_synth_alarm.wav", "alertvolume"=w489) -> ()  [unwired: 10 in]
                                }
                              }
                            }
                            frame #1 {
                              n464 = local read "Run"() -> (w493:bool)
                              n465 = case shown="True" w493 {
                                frame False {
                                n466 = Wait (ms)(milliseconds to wait=u32 50) -> ()  [unwired: 1 out]
                                }
                                frame True {
                                n467 = Wait (ms)(milliseconds to wait=u32 5000) -> ()  [unwired: 1 out]
                                }
                              }
                            }
                          }
                        }
                        frame "H1AH2A" {
                          n468 = flat-sequence {
                            frame #0 {
                              n469 = local read "Audio On / Off"() -> (w499:bool)
                              n470 = local read "H1 online"() -> (w497:bool)
                              n471 = local read "H2 online"() -> (w498:bool)
                              n472 = Compound Arithmetic op=AND(w497, w498, w499) -> (w496:bool)
                              n473 = case shown="True" w496 {
                                frame False {
                                }
                                frame True {
                                n474 = local read "Run"() -> (w502:bool)
                                n475 = case shown="True" w502 {
                                tunnel: [0.001 w504] -> w501
                                frame False {
                                }
                                frame True {
                                n476 = local read "Alert volume"() -> (w504:u32)
                                }
                                }
                                n477 = call "PlayAlarm.vi"("wavefilename"="audio\\bass_synth_alarm.wav", "alertvolume"=w501) -> ()  [unwired: 10 in]
                                }
                              }
                            }
                            frame #1 {
                              n478 = local read "Run"() -> (w505:bool)
                              n479 = case shown="True" w505 {
                                frame False {
                                n480 = Wait (ms)(milliseconds to wait=u32 50) -> ()  [unwired: 1 out]
                                }
                                frame True {
                                n481 = Wait (ms)(milliseconds to wait=u32 5000) -> ()  [unwired: 1 out]
                                }
                              }
                            }
                          }
                        }
                      }
                    }
                  }
                  n482 = local read "Run"() -> (w409:bool)
                  n483 = local read "POWER"() -> (w412:bool)
                  n484 = Not(x=w412) -> (.not. x?=w414:bool)
                  n485 = Not(x=w409) -> (.not. x?=w413:bool)
                  n486 = Compound Arithmetic op=OR(w414, w413) -> (w411:bool)
                }
              }
            }
            n487 = while {
              shift-right: [w1736] -> _
              shift-left: T6."H1NH2N" ("system statuts") -> [w1726]
              stop <- w1725 continue-if-true
              # "system status state machine:\n- writes data log whenever there is a change (if data loggin enabled)\n- issues email and text alerts is enabled (electronic notification of alarms)"
              n488 = local read "H1 parallelism"() -> (w1732:u32)
              n489 = local read "H1 Device Count"() -> (w1733:u32)
              n490 = local read "H2 Device Count"() -> (w1731:u32)
              n491 = local read "H2 parallelism"() -> (w1730:u32)
              n492 = local read "POWER"() -> (w1725:bool)
              n493 = Divide(x=w1731, y=w1730) -> (x/y=w1727:dbl)
              n494 = Divide(x=w1733, y=w1732) -> (x/y=w1728:dbl)
              n495 = local read "Ignore alarms until AFTER this many cycles"() -> (w1735:i32)
              n496 = Add(x=w1728, y=w1727) -> (x+y=w1729:dbl)
              n497 = Greater?(x=w1729, y=w1735) -> (0:w1734:bool)
              n498 = case shown="True" w1734 {
                tunnel: [w1738 w1741] -> w1736
                tunnel: w1726 -> [w1738 w1739]
                frame False {
                }
                frame True {
                  n499 = flat-sequence {
                    tunnel: [w1742] -> w1740
                    tunnel: w1739 -> [w1742]
                    tunnel: [w1839] -> w1741
                    tunnel: w1740 -> [w1837]
                    frame #0 {
                      # "Determine current state for System Status state-machine"
                      n500 = stacked-sequence {
                        frame #0 {
                          n501 = local read "H1 nominal 2"() -> (w1746:bool)
                          n502 = local read "H2 nominal 2"() -> (w1744:bool)
                          n503 = local read "H1 nominal"() -> (w1747:bool)
                          n504 = local read "H2 nominal"() -> (w1745:bool)
                          n505 = Compound Arithmetic op=AND(w1747, w1746, w1745, w1744) -> (w1743:bool)
                          n506 = case shown="True" w1743 {
                            frame False {
                            }
                            frame True {
                              n507 = local write "system statuts hid"(T6."H1NH2N" ("system statuts")) -> ()
                            }
                          }
                        }
                        frame #1 {
                          n508 = local read "H2 warning 2"() -> (w1751:bool)
                          n509 = local read "H2 warning"() -> (w1752:bool)
                          n510 = local read "H1 nominal 2"() -> (w1753:bool)
                          n511 = local read "H1 nominal"() -> (w1754:bool)
                          n512 = Or(x=w1752, y=w1751) -> (x .or. y?=w1750:bool)
                          n513 = Compound Arithmetic op=AND(w1754, w1753, w1750) -> (w1749:bool)
                          n514 = case shown="False" w1749 {
                            frame False {
                            }
                            frame True {
                              n515 = local write "system statuts hid"(T6."H1NH2W" ("system statuts")) -> ()
                            }
                          }
                        }
                        frame #2 {
                          n516 = local read "H1 nominal 2"() -> (w1761:bool)
                          n517 = local read "H1 nominal"() -> (w1762:bool)
                          n518 = local read "H2 alarm 2"() -> (w1759:bool)
                          n519 = local read "H2 alarm"() -> (w1760:bool)
                          n520 = Or(x=w1760, y=w1759) -> (x .or. y?=w1757:bool)
                          n521 = And(x=w1762, y=w1761) -> (x .and. y?=w1758:bool)
                          n522 = And(x=w1758, y=w1757) -> (x .and. y?=w1756:bool)
                          n523 = case shown="True" w1756 {
                            frame False {
                            }
                            frame True {
                              n524 = local write "system statuts hid"(T6."H1NH2A" ("system statuts")) -> ()
                            }
                          }
                        }
                        frame #3 {
                          n525 = local read "H1 alarm 2"() -> (w1772:bool)
                          n526 = local read "H1 alarm"() -> (w1773:bool)
                          n527 = local read "H2 nominal 2"() -> (w1775:bool)
                          n528 = local read "H1 warning 2"() -> (w1768:bool)
                          n529 = local read "H1 warning"() -> (w1769:bool)
                          n530 = local read "H2 nominal"() -> (w1774:bool)
                          n531 = Not(x=w1773) -> (.not. x?=w1771:bool)
                          n532 = Not(x=w1772) -> (.not. x?=w1770:bool)
                          n533 = Or(x=w1769, y=w1768) -> (x .or. y?=w1766:bool)
                          n534 = And(x=w1771, y=w1770) -> (x .and. y?=w1765:bool)
                          n535 = And(x=w1774, y=w1775) -> (x .and. y?=w1764:bool)
                          n536 = Compound Arithmetic op=AND(w1766, w1765, w1764) -> (w1767:bool)
                          n537 = case shown="True" w1767 {
                            frame False {
                            }
                            frame True {
                              n538 = local write "system statuts hid"(T6."H1WH2N" ("system statuts")) -> ()
                            }
                          }
                        }
                        frame #4 {
                          n539 = local read "H1 alarm 2"() -> (w1787:bool)
                          n540 = local read "H2 alarm 2"() -> (w1792:bool)
                          n541 = local read "H1 alarm"() -> (w1786:bool)
                          n542 = local read "H2 alarm"() -> (w1793:bool)
                          n543 = local read "H1 warning 2"() -> (w1783:bool)
                          n544 = local read "H2 warning 2"() -> (w1784:bool)
                          n545 = local read "H1 warning"() -> (w1782:bool)
                          n546 = local read "H2 warning"() -> (w1785:bool)
                          n547 = Not(x=w1786) -> (.not. x?=w1788:bool)
                          n548 = Not(x=w1787) -> (.not. x?=w1789:bool)
                          n549 = Not(x=w1793) -> (.not. x?=w1791:bool)
                          n550 = Not(x=w1792) -> (.not. x?=w1790:bool)
                          n551 = Or(x=w1782, y=w1783) -> (x .or. y?=w1780:bool)
                          n552 = Or(x=w1785, y=w1784) -> (x .or. y?=w1778:bool)
                          n553 = And(x=w1788, y=w1789) -> (x .and. y?=w1779:bool)
                          n554 = And(x=w1791, y=w1790) -> (x .and. y?=w1777:bool)
                          n555 = Compound Arithmetic op=AND(w1780, w1779, w1778, w1777) -> (w1781:bool)
                          n556 = case shown="True" w1781 {
                            frame False {
                            }
                            frame True {
                              n557 = local write "system statuts hid"(T6."H1WH2W" ("system statuts")) -> ()
                            }
                          }
                        }
                        frame #5 {
                          n558 = local read "H1 alarm 2"() -> (w1800:bool)
                          n559 = local read "H1 alarm"() -> (w1801:bool)
                          n560 = local read "H1 warning 2"() -> (w1803:bool)
                          n561 = local read "H1 warning"() -> (w1804:bool)
                          n562 = local read "H2 alarm 2"() -> (w1805:bool)
                          n563 = local read "H2 alarm"() -> (w1806:bool)
                          n564 = Not(x=w1801) -> (.not. x?=w1799:bool)
                          n565 = Not(x=w1800) -> (.not. x?=w1798:bool)
                          n566 = Or(x=w1804, y=w1803) -> (x .or. y?=w1797:bool)
                          n567 = Or(x=w1806, y=w1805) -> (x .or. y?=w1795:bool)
                          n568 = And(x=w1799, y=w1798) -> (x .and. y?=w1796:bool)
                          n569 = Compound Arithmetic op=AND(w1797, w1796, w1795) -> (w1802:bool)
                          n570 = case shown="True" w1802 {
                            frame False {
                            }
                            frame True {
                              n571 = local write "system statuts hid"(T6."H1WH2A" ("system statuts")) -> ()
                            }
                          }
                        }
                        frame #6 {
                          n572 = local read "H2 nominal 2"() -> (w1813:bool)
                          n573 = local read "H2 nominal"() -> (w1814:bool)
                          n574 = local read "H1 alarm 2"() -> (w1811:bool)
                          n575 = local read "H1 alarm"() -> (w1812:bool)
                          n576 = Or(x=w1812, y=w1811) -> (x .or. y?=w1809:bool)
                          n577 = And(x=w1814, y=w1813) -> (x .and. y?=w1808:bool)
                          n578 = And(x=w1809, y=w1808) -> (x .and. y?=w1810:bool)
                          n579 = case shown="True" w1810 {
                            frame False {
                            }
                            frame True {
                              n580 = local write "system statuts hid"(T6."H1AH2N" ("system statuts")) -> ()
                            }
                          }
                        }
                        frame #7 {
                          n581 = local read "H2 alarm 2"() -> (w1818:bool)
                          n582 = local read "H2 alarm"() -> (w1819:bool)
                          n583 = local read "H2 warning 2"() -> (w1824:bool)
                          n584 = local read "H2 warning"() -> (w1825:bool)
                          n585 = local read "H1 alarm 2"() -> (w1826:bool)
                          n586 = local read "H1 alarm"() -> (w1827:bool)
                          n587 = Not(x=w1819) -> (.not. x?=w1817:bool)
                          n588 = Not(x=w1818) -> (.not. x?=w1816:bool)
                          n589 = Or(x=w1827, y=w1826) -> (x .or. y?=w1822:bool)
                          n590 = Or(x=w1825, y=w1824) -> (x .or. y?=w1821:bool)
                          n591 = And(x=w1817, y=w1816) -> (x .and. y?=w1820:bool)
                          n592 = Compound Arithmetic op=AND(w1822, w1821, w1820) -> (w1823:bool)
                          n593 = case shown="True" w1823 {
                            frame False {
                            }
                            frame True {
                              n594 = local write "system statuts hid"(T6."H1AH2W" ("system statuts")) -> ()
                            }
                          }
                        }
                        frame #8 {
                          n595 = local read "H1 alarm 2"() -> (w1833:bool)
                          n596 = local read "H2 alarm 2"() -> (w1832:bool)
                          n597 = local read "H1 alarm"() -> (w1834:bool)
                          n598 = local read "H2 alarm"() -> (w1831:bool)
                          n599 = Or(x=w1834, y=w1833) -> (x .or. y?=w1829:bool)
                          n600 = Or(x=w1831, y=w1832) -> (x .or. y?=w1830:bool)
                          n601 = And(x=w1829, y=w1830) -> (x .and. y?=w1835:bool)
                          n602 = case shown="True" w1835 {
                            frame False {
                            }
                            frame True {
                              n603 = local write "system statuts hid"(T6."H1AH2A" ("system statuts")) -> ()
                            }
                          }
                        }
                      }
                    }
                    frame #1 {
                      n604 = local read "system statuts hid"() -> (w1839:T6)
                      n605 = Not Equal?(x=w1839, y=w1837) -> (x != y?=w1838:bool)
                      n606 = case shown="True" w1838 {
                        tunnel: w1839 -> [_ w1841]
                        frame False {
                        }
                        frame True {
                          n607 = local read "Enable data logging of all events"() -> (w1840:bool)
                          n608 = case shown="True" w1840 {
                            tunnel: w1841 -> [_ w1842]
                            frame False {
                            }
                            frame True {
                              n609 = stacked-sequence {
                                tunnel: w1842 -> [_ w1845 _ _ _]
                                frame #0 {
                                n610 = local read "Number of data log entries hid"() -> (w1844:u32)
                                n611 = Increment(x=w1844) -> (x+1=w1843:u32)
                                n612 = local write "Number of data log entries hid"(w1843) -> ()
                                }
                                frame #1 {
                                n613 = case shown="\"H1AH2A\"" w1845 {
                                frame "H1NH2N", Default {
                                w1852 = "\r\n"
                                n614 = local read "H1 online"() -> (w1869:bool)
                                n615 = local read "H2 online"() -> (w1870:bool)
                                n616 = local read "Number of data log entries hid"() -> (w1846:u32)
                                n617 = local read "H1 UPH warning limit hid"() -> (w1865:dbl)
                                n618 = local read "H2 UPH warning limit hid"() -> (w1867:dbl)
                                n619 = local read "YieldMon"() -> (w1850:cluster{i32, i32, i32, i32})
                                n620 = local read "H2  low yield warning"() -> (w1866:dbl)
                                n621 = local read "H1 low yield warning"() -> (w1864:dbl)
                                n622 = local read "H1 UPH"() -> (w1858:cluster{u32, u32})
                                n623 = local read "H2 UPH"() -> (w1856:cluster{u32, u32})
                                n624 = local read "YieldMon"() -> (w1848:cluster{i32, i32, i32, i32})
                                n625 = case shown="True" w1869 {
                                tunnel: ["H1 Off-Line" "H1 On-Line"] -> w1871
                                frame False {
                                }
                                frame True {
                                }
                                }
                                n626 = case shown="True" w1870 {
                                tunnel: ["H2 Off-Line" "H2 On-Line"] -> w1880
                                frame False {
                                }
                                frame True {
                                }
                                }
                                n627 = Unbundle(w1850) -> (w1849:i32)  [unwired: 3 out]
                                n628 = Unbundle(w1858) -> (w1857:u32)  [unwired: 1 out]
                                n629 = Unbundle(w1848) -> (w1847:i32)  [unwired: 3 out]
                                n630 = Unbundle(w1856) -> (w1855:u32)  [unwired: 1 out]
                                n631 = local read "Data log path and filename"() -> (w1854:path)
                                n632 = Number To Decimal String(number=w1864) -> (decimal integer string=w1873:string)  [unwired: 1 in]
                                n633 = Number To Decimal String(number=w1849) -> (decimal integer string=w1875:string)  [unwired: 1 in]
                                n634 = Number To Decimal String(number=w1865) -> (decimal integer string=w1877:string)  [unwired: 1 in]
                                n635 = Number To Decimal String(number=w1857) -> (decimal integer string=w1879:string)  [unwired: 1 in]
                                n636 = Number To Decimal String(number=w1866) -> (decimal integer string=w1882:string)  [unwired: 1 in]
                                n637 = Number To Decimal String(number=w1847) -> (decimal integer string=w1884:string)  [unwired: 1 in]
                                n638 = Number To Decimal String(number=w1867) -> (decimal integer string=w1886:string)  [unwired: 1 in]
                                n639 = Number To Decimal String(number=w1855) -> (decimal integer string=w1888:string)  [unwired: 1 in]
                                n640 = Number To Decimal String(number=w1846) -> (decimal integer string=w1851:string)  [unwired: 1 in]
                                n641 = Get Date/Time String(want seconds? (F)=TRUE) -> (date string=w1862:string, time string=w1863:string)  [unwired: 2 in]
                                n642 = Concatenate Strings(w1851, w1852, w1862, "   " ("string"), w1863, w1852, "H1 Nominal, H2 Nominal", w1852, w1871, w1852, "H1 Low Yield Warning Limit: ", w1873, ", H1 yield = ", w1875, w1852, "H1 Low UPH Warning Limit: ", w1877, ", H1 UPH = ", w1879, w1852, w1880, w1852, "H2 Low Yield Warning Limit: ", w1882, ", H2 yield = ", w1884, w1852, "H2 Low UPH Warning Limit: ", w1886, ", H2 UPH = ", w1888, w1852, w1852) -> (w1860:string)
                                n643 = call "SentinelDatalog.vi"("operation (0:open)"=T7."open", "String"=w1860, "data log path"=w1854) -> ()  [unwired: 8 in, 1 out]
                                }
                                frame "H1NH2W" {
                                w1898 = "\r\n"
                                n644 = local read "H1 online"() -> (w1916:bool)
                                n645 = local read "H2 online"() -> (w1917:bool)
                                n646 = local read "H1 UPH warning limit hid"() -> (w1912:dbl)
                                n647 = local read "H2 UPH warning limit hid"() -> (w1914:dbl)
                                n648 = local read "YieldMon"() -> (w1897:cluster{i32, i32, i32, i32})
                                n649 = local read "H2  low yield warning"() -> (w1913:dbl)
                                n650 = local read "H1 low yield warning"() -> (w1911:dbl)
                                n651 = local read "H1 UPH"() -> (w1905:cluster{u32, u32})
                                n652 = local read "H2 UPH"() -> (w1903:cluster{u32, u32})
                                n653 = local read "YieldMon"() -> (w1895:cluster{i32, i32, i32, i32})
                                n654 = local read "Number of data log entries hid"() -> (w1893:u32)
                                n655 = case shown="True" w1916 {
                                tunnel: ["H1 Off-Line" "H1 On-Line"] -> w1918
                                frame False {
                                }
                                frame True {
                                }
                                }
                                n656 = case shown="True" w1917 {
                                tunnel: ["H2 Off-Line" "H2 On-Line"] -> w1927
                                frame False {
                                }
                                frame True {
                                }
                                }
                                n657 = Unbundle(w1895) -> (w1894:i32)  [unwired: 3 out]
                                n658 = Unbundle(w1905) -> (w1904:u32)  [unwired: 1 out]
                                n659 = Unbundle(w1897) -> (w1896:i32)  [unwired: 3 out]
                                n660 = Unbundle(w1903) -> (w1902:u32)  [unwired: 1 out]
                                n661 = Number To Decimal String(number=w1911) -> (decimal integer string=w1920:string)  [unwired: 1 in]
                                n662 = Number To Decimal String(number=w1894) -> (decimal integer string=w1922:string)  [unwired: 1 in]
                                n663 = Number To Decimal String(number=w1912) -> (decimal integer string=w1924:string)  [unwired: 1 in]
                                n664 = Number To Decimal String(number=w1904) -> (decimal integer string=w1926:string)  [unwired: 1 in]
                                n665 = Number To Decimal String(number=w1913) -> (decimal integer string=w1929:string)  [unwired: 1 in]
                                n666 = Number To Decimal String(number=w1896) -> (decimal integer string=w1931:string)  [unwired: 1 in]
                                n667 = Number To Decimal String(number=w1914) -> (decimal integer string=w1933:string)  [unwired: 1 in]
                                n668 = Number To Decimal String(number=w1902) -> (decimal integer string=w1935:string)  [unwired: 1 in]
                                n669 = Number To Decimal String(number=w1893) -> (decimal integer string=w1899:string)  [unwired: 1 in]
                                n670 = local read "Data log path and filename"() -> (w1901:path)
                                n671 = Get Date/Time String(want seconds? (F)=TRUE) -> (date string=w1909:string, time string=w1910:string)  [unwired: 2 in]
                                n672 = Concatenate Strings(w1899, w1898, w1909, "   " ("string"), w1910, w1898, "H1 Nominal, H2 Warning", w1898, w1918, w1898, "H1 Low Yield Warning Limit: ", w1920, ", H1 yield = ", w1922, w1898, "H1 Low UPH Warning Limit: ", w1924, ", H1 UPH = ", w1926, w1898, w1927, w1898, "H2 Low Yield Warning Limit: ", w1929, ", H2 yield = ", w1931, w1898, "H2 Low UPH Warning Limit: ", w1933, ", H2 UPH = ", w1935, w1898, w1898) -> (w1907:string)
                                n673 = call "SentinelDatalog.vi"("operation (0:open)"=T7."open", "String"=w1907, "data log path"=w1901) -> ()  [unwired: 8 in, 1 out]
                                }
                                frame "H1NH2A" {
                                w1946 = "\r\n"
                                n674 = local read "H1 online"() -> (w1963:bool)
                                n675 = local read "H2 online"() -> (w1964:bool)
                                n676 = local read "Number of data log entries hid"() -> (w1940:u32)
                                n677 = local read "H1 UPH warning limit hid"() -> (w1959:dbl)
                                n678 = local read "H1 low yield warning"() -> (w1958:dbl)
                                n679 = local read "H2 UPH alarm limit hid"() -> (w1961:dbl)
                                n680 = local read "YieldMon"() -> (w1944:cluster{i32, i32, i32, i32})
                                n681 = local read "H1 UPH"() -> (w1952:cluster{u32, u32})
                                n682 = local read "H2 low yield alarm"() -> (w1960:dbl)
                                n683 = local read "H2 UPH"() -> (w1951:cluster{u32, u32})
                                n684 = local read "YieldMon"() -> (w1942:cluster{i32, i32, i32, i32})
                                n685 = case shown="True" w1963 {
                                tunnel: ["H1 Off-Line" "H1 On-Line"] -> w1965
                                frame False {
                                }
                                frame True {
                                }
                                }
                                n686 = case shown="True" w1964 {
                                tunnel: ["H2 Off-Line" "H2 On-Line"] -> w1974
                                frame False {
                                }
                                frame True {
                                }
                                }
                                n687 = Number To Decimal String(number=w1940) -> (decimal integer string=w1945:string)  [unwired: 1 in]
                                n688 = Unbundle(w1944) -> (w1943:i32)  [unwired: 3 out]
                                n689 = Unbundle(w1952) -> (w1949:u32)  [unwired: 1 out]
                                n690 = Unbundle(w1942) -> (w1941:i32)  [unwired: 3 out]
                                n691 = Unbundle(w1951) -> (w1950:u32)  [unwired: 1 out]
                                n692 = Number To Decimal String(number=w1958) -> (decimal integer string=w1967:string)  [unwired: 1 in]
                                n693 = Number To Decimal String(number=w1943) -> (decimal integer string=w1969:string)  [unwired: 1 in]
                                n694 = Number To Decimal String(number=w1959) -> (decimal integer string=w1971:string)  [unwired: 1 in]
                                n695 = Number To Decimal String(number=w1949) -> (decimal integer string=w1973:string)  [unwired: 1 in]
                                n696 = Number To Decimal String(number=w1960) -> (decimal integer string=w1976:string)  [unwired: 1 in]
                                n697 = Number To Decimal String(number=w1941) -> (decimal integer string=w1978:string)  [unwired: 1 in]
                                n698 = Number To Decimal String(number=w1961) -> (decimal integer string=w1980:string)  [unwired: 1 in]
                                n699 = Number To Decimal String(number=w1950) -> (decimal integer string=w1982:string)  [unwired: 1 in]
                                n700 = local read "Data log path and filename"() -> (w1948:path)
                                n701 = Get Date/Time String(want seconds? (F)=TRUE) -> (date string=w1956:string, time string=w1957:string)  [unwired: 2 in]
                                n702 = Concatenate Strings(w1945, w1946, w1956, "   " ("string"), w1957, w1946, "H1 Nominal, H2 Alarming", w1946, w1965, w1946, "H1 Low Yield Warning Limit: ", w1967, ", H1 yield = ", w1969, w1946, "H1 Low UPH Warning Limit: ", w1971, ", H1 UPH = ", w1973, w1946, w1974, w1946, "H2 Low Yield Alarm Limit: ", w1976, ", H2 yield = ", w1978, w1946, "H2 Low UPH Alarm Limit: ", w1980, ", H2 UPH = ", w1982, w1946, w1946) -> (w1954:string)
                                n703 = call "SentinelDatalog.vi"("operation (0:open)"=T7."open", "String"=w1954, "data log path"=w1948) -> ()  [unwired: 8 in, 1 out]
                                }
                                frame "H1WH2N" {
                                w1993 = "\r\n"
                                n704 = local read "H1 online"() -> (w2011:bool)
                                n705 = local read "H2 online"() -> (w2012:bool)
                                n706 = local read "H1 UPH warning limit hid"() -> (w2007:dbl)
                                n707 = local read "H2 UPH warning limit hid"() -> (w2009:dbl)
                                n708 = local read "H2  low yield warning"() -> (w2008:dbl)
                                n709 = local read "H1 low yield warning"() -> (w2006:dbl)
                                n710 = local read "H1 UPH"() -> (w1999:cluster{u32, u32})
                                n711 = local read "H2 UPH"() -> (w1998:cluster{u32, u32})
                                n712 = local read "YieldMon"() -> (w1991:cluster{i32, i32, i32, i32})
                                n713 = local read "YieldMon"() -> (w1989:cluster{i32, i32, i32, i32})
                                n714 = local read "Number of data log entries hid"() -> (w1987:u32)
                                n715 = case shown="True" w2011 {
                                tunnel: ["H1 Off-Line" "H1 On-Line"] -> w2000
                                frame False {
                                }
                                frame True {
                                }
                                }
                                n716 = case shown="True" w2012 {
                                tunnel: ["H2 Off-Line" "H2 On-Line"] -> w2021
                                frame False {
                                }
                                frame True {
                                }
                                }
                                n717 = Unbundle(w1991) -> (w1990:i32)  [unwired: 3 out]
                                n718 = Unbundle(w1999) -> (w1996:u32)  [unwired: 1 out]
                                n719 = Unbundle(w1989) -> (w1988:i32)  [unwired: 3 out]
                                n720 = Unbundle(w1998) -> (w1997:u32)  [unwired: 1 out]
                                n721 = Number To Decimal String(number=w2006) -> (decimal integer string=w2014:string)  [unwired: 1 in]
                                n722 = Number To Decimal String(number=w1990) -> (decimal integer string=w2016:string)  [unwired: 1 in]
                                n723 = Number To Decimal String(number=w2007) -> (decimal integer string=w2018:string)  [unwired: 1 in]
                                n724 = Number To Decimal String(number=w1996) -> (decimal integer string=w2020:string)  [unwired: 1 in]
                                n725 = Number To Decimal String(number=w2008) -> (decimal integer string=w2023:string)  [unwired: 1 in]
                                n726 = Number To Decimal String(number=w1988) -> (decimal integer string=w2025:string)  [unwired: 1 in]
                                n727 = Number To Decimal String(number=w2009) -> (decimal integer string=w2027:string)  [unwired: 1 in]
                                n728 = Number To Decimal String(number=w1997) -> (decimal integer string=w2029:string)  [unwired: 1 in]
                                n729 = local read "Data log path and filename"() -> (w1995:path)
                                n730 = Number To Decimal String(number=w1987) -> (decimal integer string=w1992:string)  [unwired: 1 in]
                                n731 = Get Date/Time String(want seconds? (F)=TRUE) -> (date string=w2004:string, time string=w2005:string)  [unwired: 2 in]
                                n732 = Concatenate Strings(w1992, w1993, w2004, "   " ("string"), w2005, w1993, "H1 Warning, H2 Nominal", w1993, w2000, w1993, "H1 Low Yield Warning Limit: ", w2014, ", H1 yield = ", w2016, w1993, "H1 Low UPH Warning Limit: ", w2018, ", H1 UPH = ", w2020, w1993, w2021, w1993, "H2 Low Yield Warning Limit: ", w2023, ", H2 yield = ", w2025, w1993, "H2 Low UPH Warning Limit: ", w2027, ", H2 UPH = ", w2029, w1993, w1993) -> (w2002:string)
                                n733 = call "SentinelDatalog.vi"("operation (0:open)"=T7."open", "String"=w2002, "data log path"=w1995) -> ()  [unwired: 8 in, 1 out]
                                }
                                frame "H1WH2W" {
                                w2039 = "\r\n"
                                w2047 = "\r\n"
                                n734 = local read "H1 online"() -> (w2058:bool)
                                n735 = local read "H2 online"() -> (w2059:bool)
                                n736 = local read "H1 UPH warning limit hid"() -> (w2054:dbl)
                                n737 = local read "H2 UPH warning limit hid"() -> (w2056:dbl)
                                n738 = local read "H2  low yield warning"() -> (w2055:dbl)
                                n739 = local read "H1 low yield warning"() -> (w2053:dbl)
                                n740 = local read "H1 UPH"() -> (w2046:cluster{u32, u32})
                                n741 = local read "H2 UPH"() -> (w2045:cluster{u32, u32})
                                n742 = local read "YieldMon"() -> (w2038:cluster{i32, i32, i32, i32})
                                n743 = local read "YieldMon"() -> (w2036:cluster{i32, i32, i32, i32})
                                n744 = case shown="True" w2058 {
                                tunnel: ["H1 Off-Line" "H1 On-Line"] -> w2060
                                frame False {
                                }
                                frame True {
                                }
                                }
                                n745 = case shown="True" w2059 {
                                tunnel: ["H2 Off-Line" "H2 On-Line"] -> w2069
                                frame False {
                                }
                                frame True {
                                }
                                }
                                n746 = local read "Number of data log entries hid"() -> (w2034:u32)
                                n747 = Unbundle(w2038) -> (w2037:i32)  [unwired: 3 out]
                                n748 = Unbundle(w2046) -> (w2044:u32)  [unwired: 1 out]
                                n749 = Unbundle(w2036) -> (w2035:i32)  [unwired: 3 out]
                                n750 = Unbundle(w2045) -> (w2043:u32)  [unwired: 1 out]
                                n751 = Number To Decimal String(number=w2053) -> (decimal integer string=w2062:string)  [unwired: 1 in]
                                n752 = Number To Decimal String(number=w2037) -> (decimal integer string=w2064:string)  [unwired: 1 in]
                                n753 = Number To Decimal String(number=w2054) -> (decimal integer string=w2066:string)  [unwired: 1 in]
                                n754 = Number To Decimal String(number=w2044) -> (decimal integer string=w2068:string)  [unwired: 1 in]
                                n755 = Number To Decimal String(number=w2055) -> (decimal integer string=w2071:string)  [unwired: 1 in]
                                n756 = Number To Decimal String(number=w2035) -> (decimal integer string=w2073:string)  [unwired: 1 in]
                                n757 = Number To Decimal String(number=w2056) -> (decimal integer string=w2075:string)  [unwired: 1 in]
                                n758 = Number To Decimal String(number=w2043) -> (decimal integer string=w2077:string)  [unwired: 1 in]
                                n759 = local read "Data log path and filename"() -> (w2042:path)
                                n760 = Get Date/Time String(want seconds? (F)=TRUE) -> (date string=w2051:string, time string=w2052:string)  [unwired: 2 in]
                                n761 = Number To Decimal String(number=w2034) -> (decimal integer string=w2040:string)  [unwired: 1 in]
                                n762 = Concatenate Strings(w2040, w2039, w2051, "   " ("string"), w2052, w2039, "H1 Warning, H2 Warning", w2039, w2060, w2039, "H1 Low Yield Warning Limit: ", w2062, ", H1 yield = ", w2064, w2047, "H1 Low UPH Warning Limit: ", w2066, ", H1 UPH = ", w2068, w2047, w2069, w2047, "H2 Low Yield Warning Limit: ", w2071, ", H2 yield = ", w2073, w2047, "H2 Low UPH Warning Limit: ", w2075, ", H2 UPH = ", w2077, w2047, w2047) -> (w2049:string)
                                n763 = call "SentinelDatalog.vi"("operation (0:open)"=T7."open", "String"=w2049, "data log path"=w2042) -> ()  [unwired: 8 in, 1 out]
                                }
                                frame "H1WH2A" {
                                w2088 = "\r\n"
                                n764 = local read "H1 online"() -> (w2105:bool)
                                n765 = local read "H2 online"() -> (w2106:bool)
                                n766 = local read "H1 UPH warning limit hid"() -> (w2101:dbl)
                                n767 = local read "H1 low yield warning"() -> (w2100:dbl)
                                n768 = local read "H2 UPH alarm limit hid"() -> (w2103:dbl)
                                n769 = local read "H1 UPH"() -> (w2094:cluster{u32, u32})
                                n770 = local read "H2 low yield alarm"() -> (w2102:dbl)
                                n771 = local read "H2 UPH"() -> (w2093:cluster{u32, u32})
                                n772 = local read "YieldMon"() -> (w2084:cluster{i32, i32, i32, i32})
                                n773 = local read "YieldMon"() -> (w2086:cluster{i32, i32, i32, i32})
                                n774 = local read "Number of data log entries hid"() -> (w2082:u32)
                                n775 = case shown="True" w2105 {
                                tunnel: ["H1 Off-Line" "H1 On-Line"] -> w2107
                                frame False {
                                }
                                frame True {
                                }
                                }
                                n776 = case shown="True" w2106 {
                                tunnel: ["H2 Off-Line" "H2 On-Line"] -> w2116
                                frame False {
                                }
                                frame True {
                                }
                                }
                                n777 = Unbundle(w2084) -> (w2083:i32)  [unwired: 3 out]
                                n778 = Unbundle(w2094) -> (w2092:u32)  [unwired: 1 out]
                                n779 = Unbundle(w2086) -> (w2085:i32)  [unwired: 3 out]
                                n780 = Unbundle(w2093) -> (w2091:u32)  [unwired: 1 out]
                                n781 = Number To Decimal String(number=w2100) -> (decimal integer string=w2109:string)  [unwired: 1 in]
                                n782 = Number To Decimal String(number=w2083) -> (decimal integer string=w2111:string)  [unwired: 1 in]
                                n783 = Number To Decimal String(number=w2101) -> (decimal integer string=w2113:string)  [unwired: 1 in]
                                n784 = Number To Decimal String(number=w2092) -> (decimal integer string=w2115:string)  [unwired: 1 in]
                                n785 = Number To Decimal String(number=w2102) -> (decimal integer string=w2118:string)  [unwired: 1 in]
                                n786 = Number To Decimal String(number=w2085) -> (decimal integer string=w2120:string)  [unwired: 1 in]
                                n787 = Number To Decimal String(number=w2103) -> (decimal integer string=w2122:string)  [unwired: 1 in]
                                n788 = Number To Decimal String(number=w2091) -> (decimal integer string=w2124:string)  [unwired: 1 in]
                                n789 = local read "Data log path and filename"() -> (w2090:path)
                                n790 = Get Date/Time String(want seconds? (F)=TRUE) -> (date string=w2098:string, time string=w2099:string)  [unwired: 2 in]
                                n791 = Number To Decimal String(number=w2082) -> (decimal integer string=w2087:string)  [unwired: 1 in]
                                n792 = Concatenate Strings(w2087, w2088, w2098, "   " ("string"), w2099, w2088, "H1 Warning, H2 Alarming", w2088, w2107, w2088, "H1 Low Yield Warning Limit: ", w2109, ", H1 yield = ", w2111, w2088, "H1 Low UPH Warning Limit: ", w2113, ", H1 UPH = ", w2115, w2088, w2116, w2088, "H2 Low Yield Alarm Limit: ", w2118, ", H2 yield = ", w2120, w2088, "H2 Low UPH Alarm Limit: ", w2122, ", H2 UPH = ", w2124, w2088, w2088) -> (w2096:string)
                                n793 = call "SentinelDatalog.vi"("operation (0:open)"=T7."open", "String"=w2096, "data log path"=w2090) -> ()  [unwired: 8 in, 1 out]
                                }
                                frame "H1AH2N" {
                                w2135 = "\r\n"
                                n794 = local read "H1 online"() -> (w2152:bool)
                                n795 = local read "H2 online"() -> (w2153:bool)
                                n796 = local read "H2 UPH warning limit hid"() -> (w2150:dbl)
                                n797 = local read "H2  low yield warning"() -> (w2149:dbl)
                                n798 = local read "H1 UPH alarm limit hid"() -> (w2148:dbl)
                                n799 = local read "H1 low yield alarm"() -> (w2147:dbl)
                                n800 = local read "H1 UPH"() -> (w2141:cluster{u32, u32})
                                n801 = local read "H2 UPH"() -> (w2140:cluster{u32, u32})
                                n802 = local read "YieldMon"() -> (w2133:cluster{i32, i32, i32, i32})
                                n803 = local read "YieldMon"() -> (w2131:cluster{i32, i32, i32, i32})
                                n804 = case shown="True" w2152 {
                                tunnel: ["H1 Off-Line" "H1 On-Line"] -> w2154
                                frame False {
                                }
                                frame True {
                                }
                                }
                                n805 = case shown="False" w2153 {
                                tunnel: ["H2 Off-Line" "H2 On-Line"] -> w2163
                                frame False {
                                }
                                frame True {
                                }
                                }
                                n806 = local read "Number of data log entries hid"() -> (w2129:u32)
                                n807 = Unbundle(w2133) -> (w2132:i32)  [unwired: 3 out]
                                n808 = Unbundle(w2141) -> (w2139:u32)  [unwired: 1 out]
                                n809 = Unbundle(w2131) -> (w2130:i32)  [unwired: 3 out]
                                n810 = Unbundle(w2140) -> (w2138:u32)  [unwired: 1 out]
                                n811 = Number To Decimal String(number=w2147) -> (decimal integer string=w2156:string)  [unwired: 1 in]
                                n812 = Number To Decimal String(number=w2132) -> (decimal integer string=w2158:string)  [unwired: 1 in]
                                n813 = Number To Decimal String(number=w2148) -> (decimal integer string=w2160:string)  [unwired: 1 in]
                                n814 = Number To Decimal String(number=w2139) -> (decimal integer string=w2162:string)  [unwired: 1 in]
                                n815 = Number To Decimal String(number=w2149) -> (decimal integer string=w2165:string)  [unwired: 1 in]
                                n816 = Number To Decimal String(number=w2130) -> (decimal integer string=w2167:string)  [unwired: 1 in]
                                n817 = Number To Decimal String(number=w2150) -> (decimal integer string=w2169:string)  [unwired: 1 in]
                                n818 = Number To Decimal String(number=w2138) -> (decimal integer string=w2171:string)  [unwired: 1 in]
                                n819 = local read "Data log path and filename"() -> (w2137:path)
                                n820 = Get Date/Time String(want seconds? (F)=TRUE) -> (date string=w2145:string, time string=w2146:string)  [unwired: 2 in]
                                n821 = Number To Decimal String(number=w2129) -> (decimal integer string=w2134:string)  [unwired: 1 in]
                                n822 = Concatenate Strings(w2134, w2135, w2145, "   " ("string"), w2146, w2135, "H1 Alarming, H2 Nominal", w2135, w2154, w2135, "H1 Low Yield Alarm Limit: ", w2156, ", H1 yield = ", w2158, w2135, "H1 Low UPH Alarm Limit: ", w2160, ", H1 UPH = ", w2162, w2135, w2163, w2135, "H2 Low Yield Warning Limit: ", w2165, ", H2 yield = ", w2167, w2135, "H2 Low UPH Warning Limit: ", w2169, ", H2 UPH = ", w2171, w2135, w2135) -> (w2143:string)
                                n823 = call "SentinelDatalog.vi"("operation (0:open)"=T7."open", "String"=w2143, "data log path"=w2137) -> ()  [unwired: 8 in, 1 out]
                                }
                                frame "H1AH2W" {
                                w2182 = "\r\n"
                                n824 = local read "H1 online"() -> (w2199:bool)
                                n825 = local read "H2 online"() -> (w2200:bool)
                                n826 = local read "H2 UPH warning limit hid"() -> (w2197:dbl)
                                n827 = local read "H2  low yield warning"() -> (w2196:dbl)
                                n828 = local read "H1 UPH alarm limit hid"() -> (w2195:dbl)
                                n829 = local read "H1 low yield alarm"() -> (w2194:dbl)
                                n830 = local read "H1 UPH"() -> (w2188:cluster{u32, u32})
                                n831 = local read "H2 UPH"() -> (w2187:cluster{u32, u32})
                                n832 = local read "YieldMon"() -> (w2180:cluster{i32, i32, i32, i32})
                                n833 = local read "YieldMon"() -> (w2178:cluster{i32, i32, i32, i32})
                                n834 = case shown="True" w2199 {
                                tunnel: ["H1 Off-Line" "H1 On-Line"] -> w2201
                                frame False {
                                }
                                frame True {
                                }
                                }
                                n835 = case shown="True" w2200 {
                                tunnel: ["H2 Off-Line" "H2 On-Line"] -> w2210
                                frame False {
                                }
                                frame True {
                                }
                                }
                                n836 = local read "Number of data log entries hid"() -> (w2176:u32)
                                n837 = Unbundle(w2180) -> (w2179:i32)  [unwired: 3 out]
                                n838 = Unbundle(w2188) -> (w2186:u32)  [unwired: 1 out]
                                n839 = Unbundle(w2178) -> (w2177:i32)  [unwired: 3 out]
                                n840 = Unbundle(w2187) -> (w2185:u32)  [unwired: 1 out]
                                n841 = Number To Decimal String(number=w2194) -> (decimal integer string=w2203:string)  [unwired: 1 in]
                                n842 = Number To Decimal String(number=w2179) -> (decimal integer string=w2205:string)  [unwired: 1 in]
                                n843 = Number To Decimal String(number=w2195) -> (decimal integer string=w2207:string)  [unwired: 1 in]
                                n844 = Number To Decimal String(number=w2186) -> (decimal integer string=w2209:string)  [unwired: 1 in]
                                n845 = Number To Decimal String(number=w2196) -> (decimal integer string=w2212:string)  [unwired: 1 in]
                                n846 = Number To Decimal String(number=w2177) -> (decimal integer string=w2214:string)  [unwired: 1 in]
                                n847 = Number To Decimal String(number=w2197) -> (decimal integer string=w2216:string)  [unwired: 1 in]
                                n848 = Number To Decimal String(number=w2185) -> (decimal integer string=w2218:string)  [unwired: 1 in]
                                n849 = local read "Data log path and filename"() -> (w2184:path)
                                n850 = Get Date/Time String(want seconds? (F)=TRUE) -> (date string=w2192:string, time string=w2193:string)  [unwired: 2 in]
                                n851 = Number To Decimal String(number=w2176) -> (decimal integer string=w2181:string)  [unwired: 1 in]
                                n852 = Concatenate Strings(w2181, w2182, w2192, "   " ("string"), w2193, w2182, "H1 Alarming, H2 Warning", w2182, w2201, w2182, "H1 Low Yield Alarm Limit: ", w2203, ", H1 yield = ", w2205, w2182, "H1 Low UPH Alarm Limit: ", w2207, ", H1 UPH = ", w2209, w2182, w2210, w2182, "H2 Low Yield Warning Limit: ", w2212, ", H2 yield = ", w2214, w2182, "H2 Low UPH Warning Limit: ", w2216, ", H2 UPH = ", w2218, w2182) -> (w2190:string)
                                n853 = call "SentinelDatalog.vi"("operation (0:open)"=T7."open", "String"=w2190, "data log path"=w2184) -> ()  [unwired: 8 in, 1 out]
                                }
                                frame "H1AH2A" {
                                w2229 = "\r\n"
                                n854 = local read "H1 online"() -> (w2246:bool)
                                n855 = local read "H2 online"() -> (w2247:bool)
                                n856 = local read "H1 UPH alarm limit hid"() -> (w2242:dbl)
                                n857 = local read "H2 UPH alarm limit hid"() -> (w2244:dbl)
                                n858 = local read "H1 low yield alarm"() -> (w2241:dbl)
                                n859 = local read "H1 UPH"() -> (w2235:cluster{u32, u32})
                                n860 = local read "H2 low yield alarm"() -> (w2243:dbl)
                                n861 = local read "H2 UPH"() -> (w2234:cluster{u32, u32})
                                n862 = local read "YieldMon"() -> (w2227:cluster{i32, i32, i32, i32})
                                n863 = local read "YieldMon"() -> (w2226:cluster{i32, i32, i32, i32})
                                n864 = case shown="True" w2246 {
                                tunnel: ["H1 Off-Line" "H1 On-Line"] -> w2248
                                frame False {
                                }
                                frame True {
                                }
                                }
                                n865 = case shown="True" w2247 {
                                tunnel: ["H2 Off-Line" "H2 On-Line"] -> w2257
                                frame False {
                                }
                                frame True {
                                }
                                }
                                n866 = local read "Number of data log entries hid"() -> (w2223:u32)
                                n867 = Unbundle(w2227) -> (w2224:i32)  [unwired: 3 out]
                                n868 = Unbundle(w2235) -> (w2233:u32)  [unwired: 1 out]
                                n869 = Unbundle(w2226) -> (w2225:i32)  [unwired: 3 out]
                                n870 = Unbundle(w2234) -> (w2232:u32)  [unwired: 1 out]
                                n871 = Number To Decimal String(number=w2241) -> (decimal integer string=w2250:string)  [unwired: 1 in]
                                n872 = Number To Decimal String(number=w2224) -> (decimal integer string=w2252:string)  [unwired: 1 in]
                                n873 = Number To Decimal String(number=w2242) -> (decimal integer string=w2254:string)  [unwired: 1 in]
                                n874 = Number To Decimal String(number=w2233) -> (decimal integer string=w2256:string)  [unwired: 1 in]
                                n875 = Number To Decimal String(number=w2243) -> (decimal integer string=w2259:string)  [unwired: 1 in]
                                n876 = Number To Decimal String(number=w2225) -> (decimal integer string=w2261:string)  [unwired: 1 in]
                                n877 = Number To Decimal String(number=w2244) -> (decimal integer string=w2263:string)  [unwired: 1 in]
                                n878 = Number To Decimal String(number=w2232) -> (decimal integer string=w2265:string)  [unwired: 1 in]
                                n879 = local read "Data log path and filename"() -> (w2231:path)
                                n880 = Get Date/Time String(want seconds? (F)=TRUE) -> (date string=w2239:string, time string=w2240:string)  [unwired: 2 in]
                                n881 = Number To Decimal String(number=w2223) -> (decimal integer string=w2228:string)  [unwired: 1 in]
                                n882 = Concatenate Strings(w2228, w2229, w2239, "   " ("string"), w2240, w2229, "H1 Alarming, H2 Alarming", w2229, w2248, w2229, "H1 Low Yield Alarm Limit: ", w2250, ", H1 yield = ", w2252, w2229, "H1 Low UPH Alarm Limit: ", w2254, ", H1 UPH = ", w2256, w2229, w2257, w2229, "H2 Low Yield Alarm Limit: ", w2259, ", H2 yield = ", w2261, w2229, "H2 Low UPH Alarm Limit: ", w2263, ", H2 UPH = ", w2265, w2229, w2229) -> (w2237:string)
                                n883 = call "SentinelDatalog.vi"("operation (0:open)"=T7."open", "String"=w2237, "data log path"=w2231) -> ()  [unwired: 8 in, 1 out]
                                }
                                }
                                }
                                frame #2 {
                                n884 = Wait (ms)(milliseconds to wait=u32 100) -> ()  [unwired: 1 out]
                                }
                                frame #3 {
                                n885 = local read "Enable electronic notification of alarms"() -> (w2271:bool)
                                n886 = case shown="True" w2271 {
                                frame False {
                                }
                                frame True {
                                n887 = stacked-sequence {
                                frame #0 {
                                # "Email"
                                n888 = local read "Enable email notification"() -> (w2274:bool)
                                n889 = local read "Number of email alerts"() -> (w2273:u32)
                                n890 = Increment(x=w2273) -> (x+1=w2272:u32)
                                n891 = local write "Number of email alerts"(w2272) -> ()
                                n892 = case shown="True" w2274 {
                                frame False {
                                }
                                frame True {
                                n893 = flat-sequence {
                                tunnel: [w2281] -> w2276
                                tunnel: [w2289] -> w2275
                                tunnel: w2276 -> [w2289]
                                tunnel: w2275 -> [w2290]
                                frame #0 {
                                n894 = local read "Data log path and filename"() -> (w2286:path)
                                n895 = local read "Number of email alerts"() -> (w2280:u32)
                                n896 = Number To Decimal String(number=w2280) -> (decimal integer string=w2279:string)  [unwired: 1 in]
                                n897 = Strip Path(path=w2286) -> (stripped path=w2284:path, name=w2278:string)
                                n898 = Path To String(path=w2284) -> (string=w2283:string)
                                n899 = Concatenate Strings(w2283, "\\sent_#" ("string"), w2279, "_" ("string"), w2278) -> (w2287:string)
                                n900 = String To Path(string=w2287) -> (path=w2282:path)
                                n901 = Copy(10:w2282, 11:w2286) -> (3:w2281:path)  [unwired: 3 in, 2 out]
                                }
                                frame #1 {
                                n902 = Wait (ms)(milliseconds to wait=u32 1000) -> ()  [unwired: 1 out]
                                }
                                frame #2 {
                                n903 = local read "Email alert - engineer"() -> (w2292:string)
                                n904 = local read "Email alert - CC"() -> (w2291:string)
                                n905 = local read "Email alert - message"() -> (w2293:string)
                                n906 = call "email_alert.vi"("Email Alert - Message"=w2293, "Email Alert - Engineer"=w2292, "Email Alert - CC"=w2291, "Email ALert - Attachment"=w2290) -> ()  [unwired: 8 in]
                                }
                                }
                                }
                                }
                                }
                                frame #1 {
                                n907 = Wait (ms)(milliseconds to wait=u32 200) -> ()  [unwired: 1 out]
                                }
                                frame #2 {
                                # "text"
                                n908 = local read "Enable text notification"() -> (w2295:bool)
                                n909 = case shown="True" w2295 {
                                frame False {
                                }
                                frame True {
                                n910 = local read "Number of text alerts"() -> (w2299:u32)
                                n911 = Increment(x=w2299) -> (x+1=w2298:u32)
                                n912 = local write "Number of text alerts"(w2298) -> ()
                                n913 = local read "Number of email alerts"() -> (w2308:u32)
                                n914 = local read "Carrier"() -> (w2301:enum16{"T-Mobile", "AT&T", "Verizon", "Sprint"})
                                n915 = local read "Phone number"() -> (w2300:string)
                                n916 = local read "Body"() -> (w2297:string)
                                n917 = local read "Lot number"() -> (w2302:string)
                                n918 = local read "Subject"() -> (w2296:string)
                                n919 = Number To Decimal String(number=w2308) -> (decimal integer string=w2304:string)  [unwired: 1 in]
                                n920 = Concatenate Strings(w2297, ", # " ("string"), w2304, ", Lot Number: " ("string"), w2302) -> (w2309:string)
                                n921 = local write "Notifications Lot Display"(w2302) -> ()
                                n922 = call <userlib>:"Send SMS 2009.vi"("Body"=w2309, "Carrier"=w2301, "Subject"=w2296, "phone number"=w2300, "smtp server"="smtp.gmail.com", "password"="sentinelcontroller", "email username"="sentinelcontroller@gmail.com") -> ("Error Out"=w2307:errorcluster)  [unwired: 4 in]
                                n923 = Unbundle By Name(w2307) -> ("status"=w2306:bool)
                                n924 = case shown="True" w2306 {
                                frame False {
                                }
                                frame True {
                                n925 = One Button Dialog(message="Warning:\nError sending text message!\nTry changing the settings or\nswitch to email method", button name ("OK")="Dismiss") -> ()  [unwired: 1 out]
                                }
                                }
                                }
                                }
                                }
                                }
                                }
                                }
                                }
                                frame #4 {
                                n926 = Wait (ms)(milliseconds to wait=u32 100) -> ()  [unwired: 1 out]
                                }
                              }
                            }
                          }
                        }
                      }
                    }
                  }
                }
              }
              n927 = Wait (ms)(milliseconds to wait=u32 100) -> ()  [unwired: 1 out]
            }
            n928 = local read "Yield averaging"() -> (w350:u32)
            n929 = local read "UPH averaging"() -> (w349:u32)
            n930 = local read "Yield averaging"() -> (w351:u32)
            n931 = local read "UPH averaging"() -> (w352:u32)
            n932 = Initialize Array(w347, w350) -> (w348:i32[])
            n933 = Initialize Array(w346, w349) -> (w345:dbl[])
            n934 = Initialize Array(w354, w351) -> (w353:i32[])
            n935 = Initialize Array(w355, w352) -> (w356:dbl[])
            n936 = while {
              shift-right: [w1279] -> _
              shift-left: w346 -> [w1285]
              shift-right: [w1280] -> _
              shift-left: w345 -> [w1284]
              shift-right: [w1281] -> _
              shift-left: w347 -> [w1278]
              shift-right: [w1282] -> _
              shift-left: w348 -> [w1283]
              stop <- w1276 stop-if-true
              # "if there is now a lock, it is unlikely that the test time is going to be less than 100ms,\nso this is a relatively slow loop"
              n937 = local read "H2 Lock"() -> (w1275:bool)
              n938 = Wait (ms)(milliseconds to wait=u32 50) -> ()  [unwired: 1 out]
              n939 = case shown="True" w1275 {
                tunnel: w1285 -> [w1290 w1315]
                tunnel: w1284 -> [w1289 w1310]
                tunnel: w1283 -> [w1287 w1307]
                tunnel: [w1287 w1301] -> w1282
                tunnel: [w1288 w1299] -> w1281
                tunnel: [w1289 w1298] -> w1280
                tunnel: [w1290 w1297] -> w1279
                tunnel: w1278 -> [w1288 w1296]
                frame False {
                  n940 = local write "Calc H1 UPH"(u32 0 ("Sim H1 UPH")) -> ()
                }
                frame True {
                  n941 = flat-sequence {
                    tunnel: w1307 -> [w1318]
                    tunnel: w1296 -> [w1319]
                    tunnel: w1310 -> [w1320]
                    tunnel: w1315 -> [w1321]
                    tunnel: [w1321] -> w1306
                    tunnel: [w1320] -> w1305
                    tunnel: [w1319] -> w1304
                    tunnel: [w1318] -> w1303
                    tunnel: [w1334] -> w1314
                    tunnel: [w1333] -> w1311
                    tunnel: [w1332] -> w1309
                    tunnel: [w1331] -> w1308
                    tunnel: w1306 -> [w1334]
                    tunnel: w1305 -> [w1333]
                    tunnel: w1304 -> [w1332]
                    tunnel: w1303 -> [w1331]
                    tunnel: w1314 -> [w1360]
                    tunnel: [w1360] -> w1313
                    tunnel: [w1359] -> w1312
                    tunnel: w1311 -> [w1359]
                    tunnel: w1309 -> [w1349]
                    tunnel: w1308 -> [w1348]
                    tunnel: [w1347] -> w1302
                    tunnel: [w1346] -> w1300
                    tunnel: w1313 -> [w1386]
                    tunnel: w1312 -> [w1387]
                    tunnel: w1302 -> [w1405]
                    tunnel: w1300 -> [w1404]
                    tunnel: [w1405] -> w1295
                    tunnel: [w1404] -> w1294
                    tunnel: [w1383] -> w1293
                    tunnel: [w1382] -> w1292
                    tunnel: [w1420] -> w1297
                    tunnel: [w1421] -> w1298
                    tunnel: [w1422] -> w1299
                    tunnel: [w1423] -> w1301
                    tunnel: w1295 -> [w1423]
                    tunnel: w1294 -> [w1422]
                    tunnel: w1293 -> [w1421]
                    tunnel: w1292 -> [w1420]
                    frame #0 {
                      n942 = local read "H2 loop counter hid"() -> (w1316:u32)
                      n943 = Equal To 0?(x=w1316) -> (x = 0?=w1317:bool)
                      n944 = case shown="True" w1317 {
                        frame False {
                        }
                        frame True {
                          # "H2 first pass init"
                          n945 = local write "H2 Device Count"(0.0 ("H2 Device Count")) -> ()
                          n946 = local write "H2 measured  Index Time"(0.0 ("H2 Index Time")) -> ()
                          n947 = local write "H2 measured Test Time"(0.0 ("H2 Test Time")) -> ()
                          n948 = local write "H2 measured Wait Time"(0.0 ("H2 Wait Time")) -> ()
                          n949 = local read "H2 low UPH alarm (%)"() -> (w1325:dbl)
                          n950 = Divide(x=w1325, y=100.0) -> (x/y=w1324:dbl)
                          n951 = Bundle(0.0, w1324) -> (w1322:cluster{dbl, dbl})  [unwired: 1 in]
                          n952 = local write "H2 UPH"(w1322) -> ()
                        }
                      }
                    }
                    frame #1 {
                      # "H2 testing"
                      n953 = while {
                        stop <- w1338 stop-if-true
                        n954 = local read "H2 Lock"() -> (w1342:bool)
                        n955 = local read "POWER"() -> (w1337:bool)
                        n956 = local read "Run"() -> (w1335:bool)
                        n957 = Not(x=w1342) -> (.not. x?=w1336:bool)
                        n958 = Not(x=w1337) -> (.not. x?=w1340:bool)
                        n959 = Not(x=w1335) -> (.not. x?=w1339:bool)
                        n960 = Compound Arithmetic op=OR(w1336, w1340, w1339) -> (w1338:bool)
                        n961 = Wait (ms)(milliseconds to wait=u32 1) -> ()  [unwired: 1 out]
                      }
                    }
                    frame #2 {
                      n962 = local read "H2 cycle yield hid"() -> (w1343:dbl)
                      n963 = local read "H2 loop counter hid"() -> (w1344:u32)
                      n964 = local read "Yield averaging"() -> (w1345:u32)
                      n965 = local read "H2 low yield alarm"() -> (w1358:dbl)
                      n966 = local read "YieldMon"() -> (w1351:cluster{i32, i32, i32, i32})
                      n967 = local read "H2  low yield warning"() -> (w1357:dbl)
                      n968 = call "moving_avg_core.vi"("Array in"=w1348, "avg"=w1345, "accumulator in"=w1349, "i"=w1344, "data in"=w1343) -> ("Array out"=w1347:dbl[], "accumulator out"=w1346:dbl, "rolling avg out"=w1352:dbl)  [unwired: 4 in]
                      n969 = Unbundle(w1351) -> (w1350:i32)  [unwired: 3 out]
                      n970 = Less?(x=w1352, y=w1357) -> (x < y?=w1356:bool)
                      n971 = case shown="True" w1356 {
                        tunnel: w1352 -> [_ w1365]
                        tunnel: w1358 -> [_ w1364]
                        frame False {
                          n972 = local write "H2 nominal"(TRUE ("H1 nominal")) -> ()
                          n973 = local write "H2 warning"(FALSE ("H1 warning")) -> ()
                          n974 = local write "H2 alarm"(FALSE ("H1 warning")) -> ()
                        }
                        frame True {
                          n975 = Less?(x=w1365, y=w1364) -> (x < y?=w1366:bool)
                          n976 = case shown="True" w1366 {
                            frame False {
                              n977 = local write "H2 nominal"(FALSE ("H1 nominal")) -> ()
                              n978 = local write "H2 warning"(TRUE ("H1 warning")) -> ()
                              n979 = local write "H2 alarm"(FALSE ("H1 warning")) -> ()
                            }
                            frame True {
                              n980 = local read "H2 enable halt\non yield alarm"() -> (w1370:bool)
                              n981 = local write "H2 nominal"(FALSE ("H1 nominal")) -> ()
                              n982 = local write "H2 alarm"(TRUE ("H1 warning")) -> ()
                              n983 = local write "H2 warning"(FALSE ("H1 warning")) -> ()
                              n984 = case shown="True" w1370 {
                                frame False {
                                }
                                frame True {
                                n985 = local write "H2 online"(FALSE ("H1 Online")) -> ()
                                }
                              }
                            }
                          }
                        }
                      }
                      n986 = local read "H1 low yield alarm"() -> (w1355:dbl)
                      n987 = local read "H2 low yield alarm"() -> (w1354:dbl)
                      n988 = Bundle(w1350, "rolling avg out"=w1352, "H1 low yield alarm"=w1355, "H2 low yield alarm"=w1354) -> (w1353:T9)  [unwired: 1 in]
                      n989 = local write "YieldMon"(w1353) -> ()
                    }
                    frame #3 {
                      n990 = local read "H2 measured  Index Time"() -> (w1376:dbl)
                      n991 = local read "H2 measured Wait Time"() -> (w1375:dbl)
                      n992 = local read "H2 measured Test Time"() -> (w1377:dbl)
                      n993 = local read "H2 parallelism"() -> (w1389:u32)
                      n994 = local read "H2 lot yield mon"() -> (w1403:dbl)
                      n995 = local write "H2 IT (scycle)"(w1376) -> ()
                      n996 = local write "H2 TT (s/cycle)"(w1377) -> ()
                      n997 = local write "H2 WT (s/cycle)"(w1375) -> ()
                      n998 = Compound Arithmetic op=ADD(w1376, w1377, w1375) -> (w1392:dbl)
                      n999 = Compound Arithmetic op=ADD(w1376, w1377) -> (w1388:dbl)
                      n1000 = Multiply(x=w1389, y=3600.0 ("x")) -> (x*y=w1391:dbl)
                      n1001 = Divide(x=w1391, y=w1392) -> (x/y=w1402:dbl)
                      n1002 = Divide(x=w1403, y=w1388) -> (x/y=w1381:dbl)
                      n1003 = local write "H2 Single Handler UPH hid"(w1381) -> ()
                      n1004 = local read "H2 low UPH warning (%)"() -> (w1399:dbl)
                      n1005 = local read "H2 loop counter hid"() -> (w1385:u32)
                      n1006 = local read "Yield averaging"() -> (w1384:u32)
                      n1007 = local read "H2 low UPH alarm (%)"() -> (w1394:dbl)
                      n1008 = property on="H2 UPH" class="Knob (strict)"() -> ("Scale.Maximum"=w1400:dbl)  [unwired: 2 in, 2 out]
                      n1009 = Divide(x=w1399, y=100.0) -> (x/y=w1398:dbl)
                      n1010 = call "moving_avg_core.vi"("Array in"=w1387, "avg"=w1384, "accumulator in"=w1386, "i"=w1385, "data in"=w1402) -> ("Array out"=w1383:dbl[], "accumulator out"=w1382:dbl, "rolling avg out"=w1401:dbl)  [unwired: 4 in]
                      n1011 = Multiply(x=w1400, y=w1398) -> (x*y=w1380:dbl)
                      n1012 = Divide(x=w1394, y=100.0) -> (x/y=w1396:dbl)
                      n1013 = local write "H2 UPH warning limit hid"(w1380) -> ()
                      n1014 = Less?(x=w1401, y=w1380) -> (x < y?=w1393:bool)
                      n1015 = Multiply(x=w1400, y=w1396) -> (x*y=w1379:dbl)
                      n1016 = case shown="True" w1393 {
                        tunnel: w1401 -> [_ w1410]
                        tunnel: w1379 -> [_ w1409]
                        frame False {
                          n1017 = local write "H2 nominal 2"(TRUE ("H1 nominal")) -> ()
                          n1018 = local write "H2 warning 2"(FALSE ("H1 warning")) -> ()
                          n1019 = local write "H2 alarm 2"(FALSE ("H1 warning")) -> ()
                        }
                        frame True {
                          n1020 = Less?(x=w1410, y=w1409) -> (x < y?=w1411:bool)
                          n1021 = case shown="True" w1411 {
                            frame False {
                              n1022 = local write "H2 nominal 2"(FALSE ("H1 nominal")) -> ()
                              n1023 = local write "H2 warning 2"(TRUE ("H1 warning")) -> ()
                              n1024 = local write "H2 alarm 2"(FALSE ("H1 warning")) -> ()
                            }
                            frame True {
                              n1025 = local read "H2 enable halt\non UPH alarm"() -> (w1415:bool)
                              n1026 = local write "H2 alarm 2"(TRUE ("H1 warning")) -> ()
                              n1027 = local write "H2 warning 2"(FALSE ("H1 warning")) -> ()
                              n1028 = local write "H2 nominal 2"(FALSE ("H1 nominal")) -> ()
                              n1029 = case shown="True" w1415 {
                                frame False {
                                }
                                frame True {
                                n1030 = local write "H2 online"(FALSE ("H1 Online")) -> ()
                                }
                              }
                            }
                          }
                        }
                      }
                      n1031 = local write "H2 UPH alarm limit hid"(w1379) -> ()
                      n1032 = Bundle("rolling avg out"=w1401, w1379) -> (w1378:cluster{"rolling avg out":dbl, dbl})  [unwired: 1 in]
                      n1033 = local write "H2 UPH"(w1378) -> ()
                    }
                    frame #4 {
                      n1034 = while {
                        stop <- w1425 continue-if-true
                        n1035 = local read "H2 Lock"() -> (w1425:bool)
                        n1036 = Wait (ms)(milliseconds to wait=u32 10) -> ()  [unwired: 1 out]
                      }
                    }
                  }
                }
              }
              n1037 = local read "POWER"() -> (w1277:bool)
              n1038 = Not(x=w1277) -> (.not. x?=w1276:bool)
            }
            n1039 = while {
              shift-right: [w2453] -> _
              shift-left: w355 -> [w2456]
              shift-right: [w2454] -> _
              shift-left: w356 -> [w2455]
              shift-right: [w2449] -> _
              shift-left: w354 -> [w2452]
              shift-right: [w2450] -> _
              shift-left: w353 -> [w2451]
              stop <- w2448 stop-if-true
              # "if there is now a lock, it is unlikely that the test time is going to be less than 100ms,\nso this is a relatively slow loop"
              n1040 = local read "H1 Lock"() -> (w2447:bool)
              n1041 = case shown="True" w2447 {
                tunnel: w2456 -> [w2462 w2487]
                tunnel: w2455 -> [w2461 w2482]
                tunnel: [w2461 w2481] -> w2454
                tunnel: [w2462 w2480] -> w2453
                tunnel: w2452 -> [w2460 w2478]
                tunnel: w2451 -> [w2459 w2476]
                tunnel: [w2459 w2474] -> w2450
                tunnel: [w2460 w2472] -> w2449
                frame False {
                  n1042 = local write "Calc H1 UPH"(u32 0 ("Sim H1 UPH")) -> ()
                }
                frame True {
                  n1043 = flat-sequence {
                    tunnel: w2476 -> [w2490]
                    tunnel: w2478 -> [w2491]
                    tunnel: w2482 -> [w2492]
                    tunnel: w2487 -> [w2493]
                    tunnel: [w2493] -> w2471
                    tunnel: [w2492] -> w2470
                    tunnel: [w2491] -> w2469
                    tunnel: [w2490] -> w2468
                    tunnel: [w2506] -> w2486
                    tunnel: [w2505] -> w2483
                    tunnel: [w2504] -> w2479
                    tunnel: [w2503] -> w2477
                    tunnel: w2471 -> [w2506]
                    tunnel: w2470 -> [w2505]
                    tunnel: w2469 -> [w2504]
                    tunnel: w2468 -> [w2503]
                    tunnel: w2486 -> [w2521]
                    tunnel: [w2521] -> w2485
                    tunnel: [w2520] -> w2484
                    tunnel: w2483 -> [w2520]
                    tunnel: w2479 -> [w2519]
                    tunnel: w2477 -> [w2518]
                    tunnel: [w2517] -> w2475
                    tunnel: [w2516] -> w2473
                    tunnel: w2485 -> [w2559]
                    tunnel: w2484 -> [w2558]
                    tunnel: w2475 -> [w2555]
                    tunnel: w2473 -> [w2554]
                    tunnel: [w2557] -> w2467
                    tunnel: [w2556] -> w2466
                    tunnel: [w2555] -> w2465
                    tunnel: [w2554] -> w2464
                    tunnel: [w2594] -> w2472
                    tunnel: [w2595] -> w2474
                    tunnel: [w2596] -> w2480
                    tunnel: [w2597] -> w2481
                    tunnel: w2467 -> [w2597]
                    tunnel: w2466 -> [w2596]
                    tunnel: w2465 -> [w2595]
                    tunnel: w2464 -> [w2594]
                    frame #0 {
                      n1044 = local read "H1 loop counter hid"() -> (w2489:u32)
                      n1045 = Equal To 0?(x=w2489) -> (x = 0?=w2488:bool)
                      n1046 = case shown="True" w2488 {
                        frame False {
                        }
                        frame True {
                          n1047 = local read "H1 low UPH alarm (%)"() -> (w2498:dbl)
                          n1048 = local write "H1 measured Index Time"(0.0 ("H1 Index Time")) -> ()
                          n1049 = local write "H1 measured Wait Time"(0.0 ("H1 Wait Time")) -> ()
                          n1050 = local write "H1 Device Count"(0.0 ("H1 Device Count")) -> ()
                          n1051 = local write "H1 measured Test Time"(0.0 ("H1 Test Time")) -> ()
                          n1052 = Divide(x=w2498, y=100.0) -> (x/y=w2496:dbl)
                          n1053 = Bundle("y"=0.0, w2496) -> (w2494:cluster{"y":dbl, dbl})  [unwired: 1 in]
                          n1054 = local write "H1 UPH"(w2494) -> ()
                        }
                      }
                    }
                    frame #1 {
                      # "H1 testing"
                      n1055 = while {
                        stop <- w2510 stop-if-true
                        n1056 = local read "H1 Lock"() -> (w2514:bool)
                        n1057 = local read "POWER"() -> (w2508:bool)
                        n1058 = local read "Run"() -> (w2507:bool)
                        n1059 = Wait (ms)(milliseconds to wait=u32 1) -> ()  [unwired: 1 out]
                        n1060 = Not(x=w2514) -> (.not. x?=w2509:bool)
                        n1061 = Not(x=w2508) -> (.not. x?=w2512:bool)
                        n1062 = Not(x=w2507) -> (.not. x?=w2511:bool)
                        n1063 = Compound Arithmetic op=OR(w2509, w2512, w2511) -> (w2510:bool)
                      }
                    }
                    frame #2 {
                      n1064 = local read "H1 cycle yield hid"() -> (w2524:dbl)
                      n1065 = local read "H1 loop counter hid"() -> (w2523:u32)
                      n1066 = local read "Yield averaging"() -> (w2522:u32)
                      n1067 = local read "H1 low yield warning"() -> (w2532:dbl)
                      n1068 = local read "H1 low yield alarm"() -> (w2530:dbl)
                      n1069 = call "moving_avg_core.vi"("Array in"=w2518, "avg"=w2522, "accumulator in"=w2519, "i"=w2523, "data in"=w2524) -> ("Array out"=w2517:dbl[], "accumulator out"=w2516:dbl, "rolling avg out"=w2527:dbl)  [unwired: 4 in]
                      n1070 = Less?(x=w2527, y=w2532) -> (x < y?=w2531:bool)
                      n1071 = case shown="True" w2531 {
                        tunnel: w2527 -> [_ w2538]
                        tunnel: w2530 -> [_ w2537]
                        frame False {
                          n1072 = local write "H1 alarm"(FALSE ("H1 warning")) -> ()
                          n1073 = local write "H1 warning"(FALSE ("H1 warning")) -> ()
                          n1074 = local write "H1 nominal"(TRUE ("H1 nominal")) -> ()
                        }
                        frame True {
                          n1075 = Less?(x=w2538, y=w2537) -> (x < y?=w2536:bool)
                          n1076 = case shown="True" w2536 {
                            frame False {
                              n1077 = local write "H1 alarm"(FALSE ("H1 warning")) -> ()
                              n1078 = local write "H1 warning"(TRUE ("H1 warning")) -> ()
                              n1079 = local write "H1 nominal"(FALSE ("H1 nominal")) -> ()
                            }
                            frame True {
                              n1080 = local read "H1 enable halt\non yield alarm"() -> (w2542:bool)
                              n1081 = local write "H1 nominal"(FALSE ("H1 nominal")) -> ()
                              n1082 = local write "H1 warning"(FALSE ("H1 warning")) -> ()
                              n1083 = local write "H1 alarm"(TRUE ("H1 warning")) -> ()
                              n1084 = case shown="True" w2542 {
                                frame False {
                                }
                                frame True {
                                n1085 = local write "H1 online"(FALSE ("H1 Online")) -> ()
                                }
                              }
                            }
                          }
                        }
                      }
                      n1086 = local read "YieldMon"() -> (w2526:cluster{i32, i32, i32, i32})
                      n1087 = local read "H1 low yield alarm"() -> (w2529:dbl)
                      n1088 = local read "H2 low yield alarm"() -> (w2528:dbl)
                      n1089 = Unbundle(w2526) -> (w2515:i32)  [unwired: 3 out]
                      n1090 = Bundle("rolling avg out"=w2527, w2515, "H1 low yield alarm"=w2529, "H2 low yield alarm"=w2528) -> (w2525:T10)  [unwired: 1 in]
                      n1091 = local write "YieldMon"(w2525) -> ()
                    }
                    frame #3 {
                      n1092 = local read "H1 measured Index Time"() -> (w2549:dbl)
                      n1093 = local read "H1 measured Wait Time"() -> (w2547:dbl)
                      n1094 = local read "H1 measured Test Time"() -> (w2548:dbl)
                      n1095 = local read "H1 parallelism"() -> (w2566:u32)
                      n1096 = local read "H1 loop counter hid"() -> (w2561:u32)
                      n1097 = local read "UPH averaging"() -> (w2560:u32)
                      n1098 = local read "H1 low UPH warning (%)"() -> (w2570:dbl)
                      n1099 = local write "H1 IT (s/cycle)"(w2549) -> ()
                      n1100 = local write "H1 TT (s/cycle)"(w2548) -> ()
                      n1101 = local write "H1 WT (s/cycle)"(w2547) -> ()
                      n1102 = Compound Arithmetic op=ADD(w2549, w2548, w2547) -> (w2562:dbl)
                      n1103 = Compound Arithmetic op=ADD(w2549, w2548) -> (w2569:dbl)
                      n1104 = Multiply(x=w2566, y=u32 3600 ("x")) -> (x*y=w2568:u32)
                      n1105 = Divide(x=w2568, y=w2569) -> (x/y=w2552:dbl)
                      n1106 = local read "H1 low UPH alarm (%)"() -> (w2575:dbl)
                      n1107 = local write "H1 Single Handler UPH hid"(w2552) -> ()
                      n1108 = property on="H1 UPH" class="Knob (strict)"() -> ("Scale.Maximum"=w2577:dbl)  [unwired: 2 in, 2 out]
                      n1109 = Divide(x=w2570, y=100.0) -> (x/y=w2571:dbl)
                      n1110 = Multiply(x=w2577, y=w2571) -> (x*y=w2550:dbl)
                      n1111 = Divide(x=w2575, y=100.0) -> (x/y=w2573:dbl)
                      n1112 = local write "H1 UPH warning limit hid"(w2550) -> ()
                      n1113 = Multiply(x=w2577, y=w2573) -> (x*y=w2551:dbl)
                      n1114 = local write "H1 UPH alarm limit hid"(w2551) -> ()
                      n1115 = local read "H1 parallelism"() -> (w2565:u32)
                      n1116 = Multiply(x=w2565, y=u32 3600 ("x")) -> (x*y=w2563:u32)
                      n1117 = Divide(x=w2563, y=w2562) -> (x/y=w2579:dbl)
                      n1118 = call "moving_avg_core.vi"("Array in"=w2558, "avg"=w2560, "accumulator in"=w2559, "i"=w2561, "data in"=w2579) -> ("Array out"=w2557:dbl[], "accumulator out"=w2556:dbl, "rolling avg out"=w2578:dbl)  [unwired: 4 in]
                      n1119 = Less?(x=w2578, y=w2550) -> (x < y?=w2576:bool)
                      n1120 = case shown="True" w2576 {
                        tunnel: w2578 -> [_ w2584]
                        tunnel: w2551 -> [_ w2583]
                        frame False {
                          n1121 = local write "H1 alarm 2"(FALSE ("H1 warning")) -> ()
                          n1122 = local write "H1 nominal 2"(TRUE ("H1 nominal")) -> ()
                          n1123 = local write "H1 warning 2"(FALSE ("H1 warning")) -> ()
                        }
                        frame True {
                          n1124 = Less?(x=w2584, y=w2583) -> (x < y?=w2585:bool)
                          n1125 = case shown="True" w2585 {
                            frame False {
                              n1126 = local write "H1 nominal 2"(FALSE ("H1 nominal")) -> ()
                              n1127 = local write "H1 warning 2"(TRUE ("H1 warning")) -> ()
                              n1128 = local write "H1 alarm 2"(FALSE ("H1 warning")) -> ()
                            }
                            frame True {
                              n1129 = local read "H1 enable halt\non UPH alarm"() -> (w2589:bool)
                              n1130 = local write "H1 warning 2"(FALSE ("H1 warning")) -> ()
                              n1131 = local write "H1 alarm 2"(TRUE ("H1 warning")) -> ()
                              n1132 = local write "H1 nominal 2"(FALSE ("H1 nominal")) -> ()
                              n1133 = case shown="True" w2589 {
                                frame False {
                                }
                                frame True {
                                n1134 = local write "H1 online"(FALSE ("H1 Online")) -> ()
                                }
                              }
                            }
                          }
                        }
                      }
                      n1135 = Bundle("rolling avg out"=w2578, w2551) -> (w2553:cluster{"rolling avg out":dbl, dbl})  [unwired: 1 in]
                      n1136 = local write "H1 UPH"(w2553) -> ()
                    }
                    frame #4 {
                      n1137 = while {
                        stop <- w2599 continue-if-true
                        n1138 = local read "H1 Lock"() -> (w2599:bool)
                        n1139 = Wait (ms)(milliseconds to wait=u32 10) -> ()  [unwired: 1 out]
                      }
                    }
                  }
                }
              }
              n1140 = Wait (ms)(milliseconds to wait=u32 50) -> ()  [unwired: 1 out]
              n1141 = local read "POWER"() -> (w2458:bool)
              n1142 = Not(x=w2458) -> (.not. x?=w2448:bool)
            }
            n1143 = while {
              stop <- w378 continue-if-true
              n1144 = while {
                stop <- w380 stop-if-true
                n1145 = event shown="[1] \"H1 online\": Value Change" {
                  selector: _ -> [_ _]
                  dyn-events: _ -> [_ _]
                  timeout: -1 -> [_ _]
                  tunnel: [_ TRUE] -> w380
                  event Timeout {
                    n1146 = event-data() -> ()  [unwired: 1 in, 2 out]
                  }
                  event "H1 online": Value Change {
                    n1147 = event-data() -> ()  [unwired: 1 in, 5 out]
                    n1148 = local read "Enable data logging of all events"() -> (w381:bool)
                    n1149 = case shown="True" w381 {
                      frame False {
                      }
                      frame True {
                        w385 = "\r\n"
                        n1150 = Get Date/Time String(want seconds? (F)=TRUE) -> (date string=w390:string, time string=w389:string)  [unwired: 2 in]
                        n1151 = local read "H1 online"() -> (w387:bool)
                        n1152 = case shown="False" w387 {
                          tunnel: ["H1 Off-Line" "H1 On-Line"] -> w386
                          frame False {
                          }
                          frame True {
                          }
                        }
                        n1153 = local read "Data log path and filename"() -> (w384:path)
                        n1154 = Concatenate Strings(w390, "   " ("string"), w389, w385, "Change in H1 Status: ", w386, w385, w385) -> (w392:string)
                        n1155 = call "SentinelDatalog.vi"("operation (0:open)"=T7."open", "String"=w392, "data log path"=w384) -> ()  [unwired: 8 in, 1 out]
                      }
                    }
                  }
                }
              }
              n1156 = local read "POWER"() -> (w378:bool)
            }
            n1157 = while {
              stop <- w360 continue-if-true
              n1158 = while {
                stop <- w362 stop-if-true
                n1159 = event shown="[1] \"H2 online\": Value Change" {
                  selector: _ -> [_ _]
                  dyn-events: _ -> [_ _]
                  timeout: -1 -> [_ _]
                  tunnel: [_ TRUE] -> w362
                  event Timeout {
                    n1160 = event-data() -> ()  [unwired: 1 in, 2 out]
                  }
                  event "H2 online": Value Change {
                    n1161 = event-data() -> ()  [unwired: 1 in, 5 out]
                    n1162 = local read "Enable data logging of all events"() -> (w363:bool)
                    n1163 = case shown="True" w363 {
                      frame False {
                      }
                      frame True {
                        w367 = "\r\n"
                        n1164 = local read "H2 online"() -> (w369:bool)
                        n1165 = case shown="False" w369 {
                          tunnel: ["H2 Off-Line" "H2 On-Line"] -> w368
                          frame False {
                          }
                          frame True {
                          }
                        }
                        n1166 = local read "Data log path and filename"() -> (w366:path)
                        n1167 = Get Date/Time String(want seconds? (F)=TRUE) -> (date string=w372:string, time string=w371:string)  [unwired: 2 in]
                        n1168 = Concatenate Strings(w372, "   " ("string"), w371, w367, "Change in H2 Status: ", w368, w367, w367) -> (w374:string)
                        n1169 = call "SentinelDatalog.vi"("operation (0:open)"=T7."open", "String"=w374, "data log path"=w366) -> ()  [unwired: 8 in, 1 out]
                      }
                    }
                  }
                }
              }
              n1170 = local read "POWER"() -> (w360:bool)
            }
            n1171 = while {
              stop <- w508 continue-if-true
              n1172 = local read "Tester online"() -> (w509:bool)
              n1173 = case shown="True" w509 {
                frame False {
                }
                frame True {
                  n1174 = flat-sequence {
                    frame #0 {
                      n1175 = local write "Exit virtual handler state machine hid"(FALSE ("Exit tester state machine hid")) -> ()
                      n1176 = local write "SC virtual handler states"(SC_virtual_handler_states."initializing bus" ("SC virtual handler states")) -> ()
                    }
                    frame #1 {
                      n1177 = flat-sequence {
                        tunnel: [w516] -> w513
                        tunnel: [w515] -> w514
                        frame #0 {
                          w515 = 0.0
                          # "These are consumed in the \"responding to sites\"\nstate when at least one handler has sites ready.  \nIt is executed only after one cycle. At that point,\nthere is at least one test period and one wait period\nto make a utilization calculation."
                          n1178 = local read "Utilization averaging"() -> (w517:i32)
                          n1179 = Initialize Array(w515, w517) -> (w516:dbl[])
                        }
                      }
                      n1180 = while {
                        shift-right: [w526] -> _
                        shift-left: w514 -> [w519]
                        shift-right: [w520] -> _
                        shift-left: w513 -> [w518]
                        stop <- w521 stop-if-true
                        n1181 = flat-sequence {
                          tunnel: w518 -> [w529]
                          tunnel: w519 -> [w530]
                          tunnel: [w532] -> w525
                          tunnel: [w531] -> w523
                          tunnel: w525 -> [w971]
                          tunnel: [w971] -> w524
                          tunnel: w523 -> [w970]
                          tunnel: [w970] -> w522
                          tunnel: [w973] -> w520
                          tunnel: [w974] -> w526
                          tunnel: w524 -> [w974]
                          tunnel: w522 -> [w973]
                          frame #0 {
                            n1182 = local read "SC virtual handler states"() -> (w528:T4)
                            n1183 = case shown="\"responding to A BIN\"" w528 {
                              tunnel: w530 -> [w533 w549 w582 w617 w737 w752 w785 w816 w839 w952 w960]
                              tunnel: [w534 w550 w583 w614 w738 w753 w784 w817 w835 w951 w959] -> w531
                              tunnel: w529 -> [w534 w550 w583 w616 w738 w753 w784 w817 w838 w951 w959]
                              tunnel: [w533 w549 w582 w615 w737 w752 w785 w816 w832 w952 w960] -> w532
                              frame "initializing bus", Default {
                                n1184 = flat-sequence {
                                frame #0 {
                                w541 = T11 1073684500 items=["Service Request"=1073684491, "Trigger"=3221168138, "Clear"=1073684493, "VXI Signal"=1073684512, "VXI/VME Interrupt"=3221168161, "VXI/VME Sysfail"=1073684509, "VXI/VME Sysreset"=1073684510, "GPIB CIC"=1073684498, "GPIB Talk"=1073684499, "GPIB Listen"=1073684500, "PXI Interrupt"=1073684514, "Serial Break"=1073684515, "Serial TermChar"=1073684516, "Serial CTS"=1073684521, "Serial DSR"=1073684522, "Serial DCD"=1073684524, "Serial RI"=1073684526, "Serial Character"=1073684533, "USB Interrupt"=1073684535, "All Enabled"=1073709055] ("Event Type")
                                n1185 = local read "SentCtrl listens to tester at"() -> (w538:refnum<visa-resource-name>)
                                n1186 = local read "GPIB wait timeout hid"() -> (w535:u32)
                                n1187 = VISA Open(VISA resource name=w538) -> (VISA resource name=w543:refnum<visa-resource-name>, error out=w542:errorcluster)  [unwired: 1 in, 3 out]
                                n1188 = Unbundle By Name(w542) -> ()  [unwired: 1 out]
                                n1189 = property class="GPIB BoardInterface"(reference=w543, error in=w542, "General Settings:Timeout Value"=w535) -> (reference out=w540:refnum<visa-resource-name>, error out=w539:errorcluster)
                                n1190 = VISA Enable Event(8:w539, 10:w541, 11:w540) -> (0:→"VISA bus 0 error out":errorcluster, 3:→"VISA bus 0 resource name out":refnum<visa-resource-name>)  [unwired: 1 out]
                                }
                                frame #1 {
                                n1191 = local write "SC virtual handler states"(SC_virtual_handler_states."waiting on event" ("SC Test Interface States")) -> ()
                                n1192 = Concatenate Strings("Bus 0 initializing " ("string"), "\r\n") -> (w545:string)
                                n1193 = local write "GPIB Bus 0 traffic"(w545) -> ()
                                }
                                frame #2 {
                                n1194 = local write "Exit virtual handler state machine hid"(FALSE ("Exit tester state machine hid")) -> ()
                                }
                                }
                              }
                              frame "waiting on event" {
                                n1195 = flat-sequence {
                                frame #0 {
                                n1196 = local read "GPIB Bus 0 traffic"() -> (w551:string)
                                n1197 = Concatenate Strings(w551, "\r\n", "Bus 0 waiting on event" ("string")) -> (w554:string)
                                n1198 = local write "GPIB Bus 0 traffic"(w554) -> ()
                                }
                                frame #1 {
                                n1199 = local read "VISA bus 0 resource name out"() -> (w564:refnum<visa-resource-name>)
                                n1200 = local read "GPIB wait timeout hid"() -> (w562:u32)
                                n1201 = local read "VISA bus 0 error out"() -> (w563:errorcluster)
                                n1202 = VISA Wait on Event(7:w562, 8:w563, 11:w564) -> (0:w555:errorcluster, 3:w556:refnum<visa-resource-name>)  [unwired: 2 in, 2 out]
                                n1203 = local write "VISA bus 0 resource name out"(w556) -> ()
                                n1204 = local write "VISA bus 0 error out"(w555) -> ()
                                n1205 = Unbundle By Name(w555) -> ("status"=w559:bool)
                                n1206 = Unbundle By Name(w555) -> ("code"=w561:i32)
                                n1207 = Equal?(x=w561, y=-1073807339) -> (x = y?=w558:bool)
                                n1208 = Or(x=w559, y=w558) -> (x .or. y?=w557:bool)
                                n1209 = case shown="True" w557 {
                                tunnel: w556 -> [_ w567]
                                tunnel: w555 -> [_ w566]
                                frame False {
                                n1210 = local write "SC virtual handler states"(SC_virtual_handler_states."reading" ("SC Test Interface States")) -> ()
                                }
                                frame True {
                                n1211 = flat-sequence {
                                tunnel: w567 -> [w571]
                                tunnel: w566 -> [w570]
                                frame #0 {
                                n1212 = VISA Close(VISA resource name=w571, error in (no error)=w570) -> (error out=w569:errorcluster)
                                n1213 = Unbundle By Name(w569) -> ("status"=w568:bool)
                                n1214 = local write "VISA bus 0 close error"(w568) -> ()
                                }
                                frame #1 {
                                n1215 = local write "VISA bus 0 close error"(FALSE ("VISA bus 0 close error")) -> ()
                                n1216 = Concatenate Strings("GPIB bus 0 error or time out waiting on event,\nclosing Bus 0 and re-initializing." ("string"), "\r\n") -> (w574:string)
                                n1217 = local write "GPIB Bus 0 traffic"(w574) -> ()
                                }
                                frame #2 {
                                n1218 = local write "SC virtual handler states"(SC_virtual_handler_states."closing bus" ("SC Test Interface States")) -> ()
                                }
                                }
                                }
                                }
                                }
                                }
                              }
                              frame "reading" {
                                n1219 = local read "VISA bus 0 resource name out"() -> (w585:refnum<visa-resource-name>)
                                n1220 = local read "VISA bus 0 error out"() -> (w586:errorcluster)
                                n1221 = local read "GPIB Bus 0 traffic"() -> (w581:string)
                                n1222 = VISA Read(VISA resource name=w585, byte count=256, error in (no error)=w586) -> (VISA resource name out=w584:refnum<visa-resource-name>, read buffer=w578:string, error out=w587:errorcluster)  [unwired: 1 out]
                                n1223 = local write "VISA bus 0 resource name out"(w584) -> ()
                                n1224 = Unbundle By Name(w587) -> ("status"=w596:bool)
                                n1225 = String Subset(string=w578, length (rest)=1 ("length (rest)")) -> (substring=w593:string)  [unwired: 1 in]
                                n1226 = local write "GPIB bus 0 read error"(w596) -> ()
                                n1227 = Concatenate Strings(w581, "\r\n", "Bus 0 read: " ("string"), w578) -> (w579:string)
                                n1228 = Equal?(x=w593, y="*") -> (x = y?=w592:bool)
                                n1229 = String Subset(string=w578, length (rest)=5 ("length (rest)")) -> (substring=w589:string)  [unwired: 1 in]
                                n1230 = local write "GPIB Bus 0 traffic"(w579) -> ()
                                n1231 = Select(t=w578, s=w592, f=w589) -> (s? t:f=w588:string)
                                n1232 = case shown="Default" w588 {
                                tunnel: w578 -> [_ _ _ _ w609 _]
                                frame "*SITES?" {
                                n1233 = local read "Tester online"() -> (w599:bool)
                                n1234 = local read "POWER"() -> (w597:bool)
                                n1235 = Compound Arithmetic op=AND(w599, w597) -> (w598:bool)
                                n1236 = case shown="True" w598 {
                                frame False {
                                n1237 = local write "SC virtual handler states"(SC_virtual_handler_states."closing bus" ("SC virtual handler states")) -> ()
                                }
                                frame True {
                                n1238 = flat-sequence {
                                frame #0 {
                                n1239 = while {
                                stop <- w602 stop-if-true
                                n1240 = local read "H1 Ready with sites"() -> (w604:bool)
                                n1241 = local read "H2 Ready with sites"() -> (w603:bool)
                                n1242 = Or(x=w604, y=w603) -> (x .or. y?=w602:bool)
                                n1243 = Wait (ms)(milliseconds to wait=u32 5) -> ()  [unwired: 1 out]
                                }
                                }
                                frame #1 {
                                n1244 = local write "SC virtual handler states"(SC_virtual_handler_states."responding to *SITES?" ("SC Test Interface States")) -> ()
                                }
                                }
                                }
                                }
                                }
                                frame "*IDN?" {
                                n1245 = local write "SC virtual handler states"(SC_virtual_handler_states."responding to *IDN?" ("SC Test Interface States")) -> ()
                                }
                                frame "*HIDN?" {
                                n1246 = local write "SC virtual handler states"(SC_virtual_handler_states."responding to *HIDN?" ("SC Test Interface States")) -> ()
                                }
                                frame "*HAND?" {
                                n1247 = local write "SC virtual handler states"(SC_virtual_handler_states."respond to *HAND?" ("SC Test Interface States")) -> ()
                                }
                                frame "A BIN" {
                                n1248 = local write "Binning_string hidden"(w609) -> ()
                                n1249 = local write "SC virtual handler states"(SC_virtual_handler_states."responding to *HIDN?" ("SC Test Interface States")) -> ()
                                }
                                frame Default {
                                n1250 = local write "SC virtual handler states"(SC_virtual_handler_states."responding to unknown command" ("SC Test Interface States")) -> ()
                                }
                                }
                              }
                              frame "responding to *SITES?" {
                                n1251 = local read "H1 Ready with sites"() -> (w612:bool)
                                n1252 = local read "H2 Ready with sites"() -> (w613:bool)
                                n1253 = Or(x=w612, y=w613) -> (x .or. y?=w618:bool)
                                n1254 = case shown="True" w618 {
                                tunnel: w617 -> [w619 w633]
                                tunnel: w616 -> [w620 w632]
                                tunnel: [w619 w626] -> w615
                                tunnel: [w620 w629] -> w614
                                frame False {
                                n1255 = local write "SC virtual handler states"(SC_virtual_handler_states."waiting on event" ("SC Test Interface States")) -> ()
                                }
                                frame True {
                                n1256 = flat-sequence {
                                tunnel: w632 -> [w636]
                                tunnel: w633 -> [w637]
                                tunnel: [w635] -> w631
                                tunnel: [w634] -> w628
                                tunnel: w631 -> [w650]
                                tunnel: [w650] -> w630
                                tunnel: w628 -> [w649]
                                tunnel: [w649] -> w627
                                tunnel: w630 -> [w724]
                                tunnel: w627 -> [w723]
                                tunnel: [w724] -> w625
                                tunnel: [w723] -> w624
                                tunnel: w625 -> [w733]
                                tunnel: w624 -> [w732]
                                tunnel: [w733] -> w623
                                tunnel: [w732] -> w622
                                tunnel: [w735] -> w626
                                tunnel: [w736] -> w629
                                tunnel: w623 -> [w736]
                                tunnel: w622 -> [w735]
                                frame #0 {
                                n1257 = local read "SC measured test time hid"() -> (w638:dbl)
                                n1258 = local read "SC measured wait time hid"() -> (w639:dbl)
                                n1259 = Add(x=w638, y=w639) -> (x+y=w645:dbl)
                                n1260 = local read "Tester loop counterhid"() -> (w641:u32)
                                n1261 = local read "Utilization averaging"() -> (w640:i32)
                                n1262 = Divide(x=w638, y=w645) -> (x/y=w646:dbl)
                                n1263 = Multiply(x=100.0, y=w646) -> (x*y=w642:dbl)
                                n1264 = call "moving_avg_core.vi"("Array in"=w636, "avg"=w640, "accumulator in"=w637, "i"=w641, "data in"=w642) -> ("Array out"=w635:dbl[], "accumulator out"=w634:dbl, "rolling avg out"=w643:dbl)  [unwired: 4 in]
                                n1265 = local write "Sys utilization"(w643) -> ()
                                n1266 = Bundle(w642, "rolling avg out"=w643) -> (w644:cluster{dbl, "rolling avg out":dbl})  [unwired: 1 in]
                                n1267 = local write "SysUtilMon"(w644) -> ()
                                }
                                frame #1 {
                                # "This is the engine that decides if H1 is checked first or H2"
                                n1268 = local read "Last locked handler"() -> (w648:enum16{"H1", "H2"})
                                n1269 = case shown="\"H1\", Default" w648 {
                                frame "H1", Default {
                                n1270 = local read "H2 Ready with sites"() -> (w651:bool)
                                n1271 = case shown="True" w651 {
                                frame False {
                                n1272 = local read "H1 Ready with sites"() -> (w652:bool)
                                n1273 = case shown="False" w652 {
                                frame False {
                                # "end up here only if neither handler is waiting and ready"
                                }
                                frame True {
                                n1274 = flat-sequence {
                                frame #0 {
                                n1275 = local write "H1 Lock"(TRUE ("H1 Lock")) -> ()
                                n1276 = local write "H2 Lock"(FALSE ("H1 Lock")) -> ()
                                n1277 = local write "Last locked handler"(enum16{"H1", "H2"}."H1" ("Last locked handler")) -> ()
                                }
                                frame #1 {
                                n1278 = while {
                                stop <- w656 stop-if-true
                                n1279 = local read "VISA bus 0 resource name out"() -> (w665:refnum<visa-resource-name>)
                                n1280 = local read "H1 sites ready hidden"() -> (w659:string)
                                n1281 = local read "VISA bus 0 error out"() -> (w666:errorcluster)
                                n1282 = VISA Write(VISA resource name=w665, write buffer=w659, error in (no error)=w666) -> (VISA resource name out=w664:refnum<visa-resource-name>, return count=w657:u32, error out=w663:errorcluster)
                                n1283 = local write "VISA bus 0 resource name out"(w664) -> ()
                                n1284 = Unbundle By Name(w663) -> ("status"=w667:bool)
                                n1285 = local write "VISA bus 0 error out"(w663) -> ()
                                n1286 = Concatenate Strings("H1: Tester test cycle start" ("string"), "\r\n", "Bus 0 write: " ("string"), w659) -> (w661:string)
                                n1287 = Greater Than 0?(x=w657) -> (x > 0?=w656:bool)
                                n1288 = local write "GPIB bus 0 write error"(w667) -> ()
                                n1289 = local write "GPIB Bus 0 traffic"(w661) -> ()
                                }
                                }
                                frame #2 {
                                n1290 = local read "H1 loop counter hid"() -> (w669:u32)
                                n1291 = Increment(x=w669) -> (x+1=w668:u32)
                                n1292 = local write "H1 loop counter hid"(w668) -> ()
                                }
                                }
                                }
                                }
                                }
                                frame True {
                                n1293 = flat-sequence {
                                frame #0 {
                                n1294 = local write "H2 Lock"(TRUE ("H1 Lock")) -> ()
                                n1295 = local write "H1 Lock"(FALSE ("H1 Lock")) -> ()
                                n1296 = local write "Last locked handler"(enum16{"H1", "H2"}."H2" ("Last locked handler")) -> ()
                                }
                                frame #1 {
                                n1297 = while {
                                stop <- w674 stop-if-true
                                n1298 = local read "VISA bus 0 resource name out"() -> (w682:refnum<visa-resource-name>)
                                n1299 = local read "H2 sites ready hidden"() -> (w676:string)
                                n1300 = local read "VISA bus 0 error out"() -> (w683:errorcluster)
                                n1301 = VISA Write(VISA resource name=w682, write buffer=w676, error in (no error)=w683) -> (VISA resource name out=w681:refnum<visa-resource-name>, return count=w673:u32, error out=w680:errorcluster)
                                n1302 = local write "VISA bus 0 resource name out"(w681) -> ()
                                n1303 = Unbundle By Name(w680) -> ("status"=w684:bool)
                                n1304 = local write "VISA bus 0 error out"(w680) -> ()
                                n1305 = Concatenate Strings("H2: Tester test cycle start" ("string"), "\r\n", "Bus 0 write: " ("string"), w676) -> (w678:string)
                                n1306 = Greater Than 0?(x=w673) -> (x > 0?=w674:bool)
                                n1307 = local write "GPIB bus 0 write error"(w684) -> ()
                                n1308 = local write "GPIB Bus 0 traffic"(w678) -> ()
                                }
                                }
                                frame #2 {
                                n1309 = local read "H2 loop counter hid"() -> (w685:u32)
                                n1310 = Increment(x=w685) -> (x+1=w686:u32)
                                n1311 = local write "H2 loop counter hid"(w686) -> ()
                                }
                                }
                                }
                                }
                                }
                                frame "H2" {
                                n1312 = local read "H1 Ready with sites"() -> (w687:bool)
                                n1313 = case shown="False" w687 {
                                frame False {
                                n1314 = local read "H2 Ready with sites"() -> (w688:bool)
                                n1315 = case shown="True" w688 {
                                frame False {
                                # "end up here only if neither handler is waiting and ready"
                                }
                                frame True {
                                n1316 = flat-sequence {
                                frame #0 {
                                n1317 = local write "H1 Lock"(FALSE ("H1 Lock")) -> ()
                                n1318 = local write "H2 Lock"(TRUE ("H1 Lock")) -> ()
                                n1319 = local write "Last locked handler"(enum16{"H1", "H2"}."H2" ("Last locked handler")) -> ()
                                }
                                frame #1 {
                                n1320 = while {
                                stop <- w693 stop-if-true
                                n1321 = local read "VISA bus 0 resource name out"() -> (w701:refnum<visa-resource-name>)
                                n1322 = local read "H2 sites ready hidden"() -> (w695:string)
                                n1323 = local read "VISA bus 0 error out"() -> (w702:errorcluster)
                                n1324 = VISA Write(VISA resource name=w701, write buffer=w695, error in (no error)=w702) -> (VISA resource name out=w700:refnum<visa-resource-name>, return count=w692:u32, error out=w699:errorcluster)
                                n1325 = local write "VISA bus 0 resource name out"(w700) -> ()
                                n1326 = Unbundle By Name(w699) -> ("status"=w703:bool)
                                n1327 = local write "VISA bus 0 error out"(w699) -> ()
                                n1328 = Concatenate Strings("H2: Tester test cycle start" ("string"), "\r\n", "Bus 0 write: " ("string"), w695) -> (w697:string)
                                n1329 = Greater Than 0?(x=w692) -> (x > 0?=w693:bool)
                                n1330 = local write "GPIB bus 0 write error"(w703) -> ()
                                n1331 = local write "GPIB Bus 0 traffic"(w697) -> ()
                                }
                                }
                                frame #2 {
                                n1332 = local read "H2 loop counter hid"() -> (w704:u32)
                                n1333 = Increment(x=w704) -> (x+1=w705:u32)
                                n1334 = local write "H2 loop counter hid"(w705) -> ()
                                }
                                }
                                }
                                }
                                }
                                frame True {
                                n1335 = flat-sequence {
                                frame #0 {
                                n1336 = local write "H1 Lock"(TRUE ("H1 Lock")) -> ()
                                n1337 = local write "H2 Lock"(FALSE ("H1 Lock")) -> ()
                                n1338 = local write "Last locked handler"(enum16{"H1", "H2"}."H1" ("Last locked handler")) -> ()
                                }
                                frame #1 {
                                n1339 = while {
                                stop <- w709 stop-if-true
                                n1340 = local read "VISA bus 0 resource name out"() -> (w718:refnum<visa-resource-name>)
                                n1341 = local read "H1 sites ready hidden"() -> (w712:string)
                                n1342 = local read "VISA bus 0 error out"() -> (w719:errorcluster)
                                n1343 = VISA Write(VISA resource name=w718, write buffer=w712, error in (no error)=w719) -> (VISA resource name out=w717:refnum<visa-resource-name>, return count=w710:u32, error out=w716:errorcluster)
                                n1344 = local write "VISA bus 0 resource name out"(w717) -> ()
                                n1345 = Unbundle By Name(w716) -> ("status"=w720:bool)
                                n1346 = local write "VISA bus 0 error out"(w716) -> ()
                                n1347 = Concatenate Strings("H1: Tester test cycle start" ("string"), "\r\n", "Bus 0 write: " ("string"), w712) -> (w714:string)
                                n1348 = Greater Than 0?(x=w710) -> (x > 0?=w709:bool)
                                n1349 = local write "GPIB bus 0 write error"(w720) -> ()
                                n1350 = local write "GPIB Bus 0 traffic"(w714) -> ()
                                }
                                }
                                frame #2 {
                                n1351 = local read "H1 loop counter hid"() -> (w722:u32)
                                n1352 = Increment(x=w722) -> (x+1=w721:u32)
                                n1353 = local write "H1 loop counter hid"(w721) -> ()
                                }
                                }
                                }
                                }
                                }
                                }
                                }
                                frame #2 {
                                n1354 = Tick Count (ms)() -> (millisecond timer value=w725:u32)
                                n1355 = Tick Count (ms)() -> (millisecond timer value=w726:u32)
                                n1356 = local write "tester tt start hidden"(w725) -> ()
                                n1357 = local write "tester wt end hidden"(w726) -> ()
                                }
                                frame #3 {
                                n1358 = local read "tester wt start hidden"() -> (w730:u32)
                                n1359 = local read "tester wt end hidden"() -> (w731:u32)
                                n1360 = Subtract(x=w731, y=w730) -> (x-y=w729:u32)
                                n1361 = Divide(x=w729, y=u32 1000) -> (x/y=w727:dbl)
                                n1362 = local write "SC measured wait time hid"(w727) -> ()
                                }
                                frame #4 {
                                n1363 = local write "SC virtual handler states"(SC_virtual_handler_states."testing" ("SC Test Interface States")) -> ()
                                }
                                }
                                }
                                }
                              }
                              frame "responding to *IDN?" {
                                n1364 = flat-sequence {
                                frame #0 {
                                n1365 = while {
                                stop <- w740 stop-if-true
                                w742 = "Sentinel Controller Handler Interface"
                                n1366 = local read "VISA bus 0 resource name out"() -> (w750:refnum<visa-resource-name>)
                                n1367 = local read "VISA bus 0 error out"() -> (w749:errorcluster)
                                n1368 = local read "GPIB Bus 0 traffic"() -> (w746:string)
                                n1369 = VISA Write(VISA resource name=w750, write buffer=w742, error in (no error)=w749) -> (VISA resource name out=w748:refnum<visa-resource-name>, return count=w741:u32, error out=w747:errorcluster)
                                n1370 = local write "VISA bus 0 resource name out"(w748) -> ()
                                n1371 = Unbundle By Name(w747) -> ("status"=w739:bool)
                                n1372 = local write "VISA bus 0 error out"(w747) -> ()
                                n1373 = Concatenate Strings(w746, "\r\n", "Bus 0 write: " ("string"), w742) -> (w744:string)
                                n1374 = Greater Than 0?(x=w741) -> (x > 0?=w740:bool)
                                n1375 = local write "GPIB bus 0 write error"(w739) -> ()
                                n1376 = local write "GPIB Bus 0 traffic"(w744) -> ()
                                }
                                }
                                frame #1 {
                                n1377 = local write "SC virtual handler states"(SC_virtual_handler_states."waiting on event" ("SC Test Interface States")) -> ()
                                }
                                }
                              }
                              frame "respond to *HAND?" {
                                n1378 = local read "H1 Lock"() -> (w754:bool)
                                n1379 = case shown="False" w754 {
                                frame False {
                                n1380 = local read "H2 Lock"() -> (w755:bool)
                                n1381 = case shown="False" w755 {
                                frame False {
                                n1382 = flat-sequence {
                                frame #0 {
                                n1383 = One Button Dialog(message="Fatal error 200:\nThe SC responded to a handler being ready with devices\nto test, but when the SC check for a lock when responding\nto *HAND?, no handler had a lock. \nPlease report this bug to Celerint at www.celerint.com  ") -> ()  [unwired: 1 in, 1 out]
                                }
                                frame #1 {
                                n1384 = local write "SC virtual handler states"(SC_virtual_handler_states."closing bus" ("SC Test Interface States")) -> ()
                                }
                                }
                                }
                                frame True {
                                n1385 = flat-sequence {
                                frame #0 {
                                n1386 = while {
                                stop <- w759 stop-if-true
                                w760 = "H2" ("string")
                                n1387 = local read "VISA bus 0 resource name out"() -> (w766:refnum<visa-resource-name>)
                                n1388 = local read "GPIB Bus 0 traffic"() -> (w764:string)
                                n1389 = local read "VISA bus 0 error out"() -> (w765:errorcluster)
                                n1390 = Concatenate Strings(w764, "\r\n", "H2: Bus 0 write: " ("string"), w760) -> (w762:string)
                                n1391 = VISA Write(VISA resource name=w766, write buffer=w760, error in (no error)=w765) -> (VISA resource name out=w767:refnum<visa-resource-name>, return count=w758:u32, error out=w768:errorcluster)
                                n1392 = local write "VISA bus 0 resource name out"(w767) -> ()
                                n1393 = Unbundle By Name(w768) -> ("status"=w769:bool)
                                n1394 = local write "VISA bus 0 error out"(w768) -> ()
                                n1395 = local write "GPIB Bus 0 traffic"(w762) -> ()
                                n1396 = Greater Than 0?(x=w758) -> (x > 0?=w759:bool)
                                n1397 = local write "GPIB bus 0 write error"(w769) -> ()
                                }
                                }
                                frame #1 {
                                n1398 = local write "SC virtual handler states"(SC_virtual_handler_states."waiting on event" ("SC Test Interface States")) -> ()
                                }
                                }
                                }
                                }
                                }
                                frame True {
                                n1399 = flat-sequence {
                                frame #0 {
                                n1400 = while {
                                stop <- w772 stop-if-true
                                w773 = "H1" ("string")
                                n1401 = local read "VISA bus 0 resource name out"() -> (w779:refnum<visa-resource-name>)
                                n1402 = local read "GPIB Bus 0 traffic"() -> (w777:string)
                                n1403 = local read "VISA bus 0 error out"() -> (w778:errorcluster)
                                n1404 = Concatenate Strings(w777, "\r\n", "H1: Bus 0 write: " ("string"), w773) -> (w775:string)
                                n1405 = VISA Write(VISA resource name=w779, write buffer=w773, error in (no error)=w778) -> (VISA resource name out=w780:refnum<visa-resource-name>, return count=w771:u32, error out=w781:errorcluster)
                                n1406 = local write "VISA bus 0 resource name out"(w780) -> ()
                                n1407 = Unbundle By Name(w781) -> ("status"=w782:bool)
                                n1408 = local write "VISA bus 0 error out"(w781) -> ()
                                n1409 = local write "GPIB Bus 0 traffic"(w775) -> ()
                                n1410 = Greater Than 0?(x=w771) -> (x > 0?=w772:bool)
                                n1411 = local write "GPIB bus 0 write error"(w782) -> ()
                                }
                                }
                                frame #1 {
                                n1412 = local write "SC virtual handler states"(SC_virtual_handler_states."waiting on event" ("SC Test Interface States")) -> ()
                                }
                                }
                                }
                                }
                              }
                              frame "responding to *HIDN?" {
                                n1413 = local read "H1 Lock"() -> (w786:bool)
                                n1414 = case shown="False" w786 {
                                frame False {
                                n1415 = local read "H2 Lock"() -> (w787:bool)
                                n1416 = case shown="False" w787 {
                                frame False {
                                n1417 = flat-sequence {
                                frame #0 {
                                n1418 = One Button Dialog(message="Fatal error 201:\nThe SC responded to a handler being ready with devices\nto test, but when the SC check for a lock when responding\nto *HIDN?, no handler had a lock. \nPlease report this bug to Celerint at www.celerint.com  ") -> ()  [unwired: 1 in, 1 out]
                                }
                                frame #1 {
                                n1419 = local write "SC virtual handler states"(SC_virtual_handler_states."testing" ("SC Test Interface States")) -> ()
                                }
                                }
                                }
                                frame True {
                                n1420 = flat-sequence {
                                frame #0 {
                                n1421 = while {
                                stop <- w791 stop-if-true
                                n1422 = local read "H2 response to *HAND? hidden"() -> (w792:string)
                                n1423 = local read "VISA bus 0 resource name out"() -> (w798:refnum<visa-resource-name>)
                                n1424 = local read "VISA bus 0 error out"() -> (w797:errorcluster)
                                n1425 = local read "GPIB Bus 0 traffic"() -> (w796:string)
                                n1426 = VISA Write(VISA resource name=w798, write buffer=w792, error in (no error)=w797) -> (VISA resource name out=w799:refnum<visa-resource-name>, return count=w790:u32, error out=w800:errorcluster)
                                n1427 = local write "VISA bus 0 resource name out"(w799) -> ()
                                n1428 = Unbundle By Name(w800) -> ("status"=w801:bool)
                                n1429 = local write "VISA bus 0 error out"(w800) -> ()
                                n1430 = Concatenate Strings(w796, "\r\n", "H2: Bus 0 write: " ("string"), w792) -> (w794:string)
                                n1431 = Greater Than 0?(x=w790) -> (x > 0?=w791:bool)
                                n1432 = local write "GPIB Bus 0 traffic"(w794) -> ()
                                n1433 = local write "GPIB bus 0 write error"(w801) -> ()
                                }
                                }
                                frame #1 {
                                n1434 = local write "SC virtual handler states"(SC_virtual_handler_states."waiting on event" ("SC Test Interface States")) -> ()
                                }
                                }
                                }
                                }
                                }
                                frame True {
                                n1435 = flat-sequence {
                                frame #0 {
                                n1436 = while {
                                stop <- w804 stop-if-true
                                n1437 = local read "H1 response to *HAND? hidden"() -> (w805:string)
                                n1438 = local read "VISA bus 0 resource name out"() -> (w811:refnum<visa-resource-name>)
                                n1439 = local read "VISA bus 0 error out"() -> (w810:errorcluster)
                                n1440 = local read "GPIB Bus 0 traffic"() -> (w809:string)
                                n1441 = VISA Write(VISA resource name=w811, write buffer=w805, error in (no error)=w810) -> (VISA resource name out=w812:refnum<visa-resource-name>, return count=w803:u32, error out=w813:errorcluster)
                                n1442 = local write "VISA bus 0 resource name out"(w812) -> ()
                                n1443 = Unbundle By Name(w813) -> ("status"=w814:bool)
                                n1444 = local write "VISA bus 0 error out"(w813) -> ()
                                n1445 = Concatenate Strings(w809, "\r\n", "H1: Bus 0 write: " ("string"), w805) -> (w807:string)
                                n1446 = Greater Than 0?(x=w803) -> (x > 0?=w804:bool)
                                n1447 = local write "GPIB Bus 0 traffic"(w807) -> ()
                                n1448 = local write "GPIB bus 0 write error"(w814) -> ()
                                }
                                }
                                frame #1 {
                                n1449 = local write "SC virtual handler states"(SC_virtual_handler_states."waiting on event" ("SC Test Interface States")) -> ()
                                }
                                }
                                }
                                }
                              }
                              frame "testing" {
                                n1450 = flat-sequence {
                                frame #0 {
                                n1451 = local read "VISA bus 0 resource name out"() -> (w822:refnum<visa-resource-name>)
                                n1452 = local read "VISA bus 0 error out"() -> (w821:errorcluster)
                                n1453 = local read "GPIB wait timeout hid"() -> (w818:u32)
                                n1454 = VISA Wait on Event(7:w818, 8:w821, 11:w822) -> (0:w819:errorcluster, 3:w820:refnum<visa-resource-name>)  [unwired: 2 in, 2 out]
                                n1455 = local write "VISA bus 0 resource name out"(w820) -> ()
                                n1456 = local write "VISA bus 0 error out"(w819) -> ()
                                }
                                frame #1 {
                                n1457 = local read "Tester loop counterhid"() -> (w824:u32)
                                n1458 = local write "SC virtual handler states"(SC_virtual_handler_states."reading" ("SC Test Interface States")) -> ()
                                n1459 = Increment(x=w824) -> (x+1=w823:u32)
                                n1460 = local write "Tester loop counterhid"(w823) -> ()
                                }
                                }
                              }
                              frame "responding to A BIN" {
                                n1461 = flat-sequence {
                                tunnel: w839 -> [w840]
                                tunnel: w838 -> [w841]
                                tunnel: [w841] -> w837
                                tunnel: [w840] -> w833
                                tunnel: w837 -> [w855]
                                tunnel: [w855] -> w836
                                tunnel: [w854] -> w834
                                tunnel: w833 -> [w854]
                                tunnel: w836 -> [w857]
                                tunnel: [w857] -> w831
                                tunnel: [w856] -> w829
                                tunnel: w834 -> [w856]
                                tunnel: w831 -> [w865]
                                tunnel: [w865] -> w830
                                tunnel: w829 -> [w864]
                                tunnel: [w864] -> w828
                                tunnel: w830 -> [w943]
                                tunnel: w828 -> [w942]
                                tunnel: [w943] -> w827
                                tunnel: [w942] -> w826
                                tunnel: [w947] -> w832
                                tunnel: [w948] -> w835
                                tunnel: w827 -> [w948]
                                tunnel: w826 -> [w947]
                                frame #0 {
                                n1462 = local read "H1 Lock"() -> (w842:bool)
                                n1463 = case shown="True" w842 {
                                frame False {
                                n1464 = local read "H2 Lock"() -> (w843:bool)
                                n1465 = case shown="False" w843 {
                                frame False {
                                }
                                frame True {
                                n1466 = local read "GPIB Bus 0 traffic"() -> (w847:string)
                                n1467 = Concatenate Strings(w847, "\r\n", "H2: Bus 0: no response " ("string")) -> (w845:string)
                                n1468 = local write "GPIB Bus 0 traffic"(w845) -> ()
                                }
                                }
                                }
                                frame True {
                                n1469 = local read "GPIB Bus 0 traffic"() -> (w851:string)
                                n1470 = Concatenate Strings(w851, "\r\n", "H1: Bus 0: no response " ("string")) -> (w849:string)
                                n1471 = local write "GPIB Bus 0 traffic"(w849) -> ()
                                }
                                }
                                }
                                frame #1 {
                                n1472 = Tick Count (ms)() -> (millisecond timer value=w853:u32)
                                n1473 = Tick Count (ms)() -> (millisecond timer value=w852:u32)
                                n1474 = local write "tester tt end hidden"(w853) -> ()
                                n1475 = local write "tester wt start hidden"(w852) -> ()
                                }
                                frame #2 {
                                n1476 = local read "tester tt start hidden"() -> (w861:u32)
                                n1477 = local read "tester tt end hidden"() -> (w862:u32)
                                n1478 = Subtract(x=w862, y=w861) -> (x-y=w860:u32)
                                n1479 = Divide(x=w860, y=u32 1000) -> (x/y=w858:dbl)
                                n1480 = local write "SC measured test time hid"(w858) -> ()
                                }
                                frame #3 {
                                n1481 = local read "H1 Lock"() -> (w863:bool)
                                n1482 = case shown="True" w863 {
                                frame False {
                                n1483 = local read "H2 Lock"() -> (w866:bool)
                                n1484 = case shown="True" w866 {
                                frame False {
                                n1485 = One Button Dialog(message="Fatal error 202:\nThe SC responded to a handler being ready with devices\nto test, but when the SC received binning data, no handler had a lock. \nPlease report this bug to Celerint at www.celerint.com  ") -> ()  [unwired: 1 in, 1 out]
                                }
                                frame True {
                                n1486 = local read "H2 online"() -> (w887:bool)
                                n1487 = local read "Tandem\nfloorspace area"() -> (w870:i32)
                                n1488 = local read "Std cell \nfloorspace area"() -> (w898:i32)
                                n1489 = case shown="True" w887 {
                                tunnel: [0 w902] -> w888
                                frame False {
                                }
                                frame True {
                                n1490 = local read "H2 UPH"() -> (w903:cluster{u32, u32})
                                n1491 = Unbundle(w903) -> (w902:u32)  [unwired: 1 out]
                                }
                                }
                                n1492 = local read "System UPH"() -> (w869:u32)
                                n1493 = local read "UPH"() -> (w899:dbl)
                                n1494 = Divide(x=w869, y=w870) -> (x/y=w868:dbl)
                                n1495 = local write "Tandem UPH\nper unit area"(w868) -> ()
                                n1496 = Divide(x=w899, y=w898) -> (x/y=w900:dbl)
                                n1497 = local read "Std hourly\ncost ($/hr)"() -> (w895:dbl)
                                n1498 = local read "H1 UPH"() -> (w897:cluster{u32, u32})
                                n1499 = local write "H1 UPH per unit area"(w900) -> ()
                                n1500 = local read "Utilization (%)"() -> (w880:u32)
                                n1501 = local read "Tandem hourly\ncost ($/hr)"() -> (w896:dbl)
                                n1502 = local read "# of devices to test"() -> (w886:u32)
                                n1503 = Unbundle(w897) -> (w889:u32)  [unwired: 1 out]
                                n1504 = local read "Hours per month"() -> (w881:i32)
                                n1505 = local write "Calc H2 UPH"(w888) -> ()
                                n1506 = local write "Calc H1 UPH"(w889) -> ()
                                n1507 = local read "UPH"() -> (w894:dbl)
                                n1508 = Add(x=w889, y=w888) -> (x+y=w876:u32)
                                n1509 = Divide(x=w880, y=u32 100) -> (x/y=w879:dbl)
                                n1510 = Divide(x=w886, y=w876) -> (x/y=w885:dbl)
                                n1511 = Multiply(x=w881, y=w879) -> (x*y=w877:dbl)
                                n1512 = Divide(x=w895, y=w894) -> (x/y=w893:dbl)
                                n1513 = Divide(x=w896, y=w876) -> (x/y=w891:dbl)
                                n1514 = local write "System UPH"(w876) -> ()
                                n1515 = local write "Calc\nsystem UPH"(w876) -> ()
                                n1516 = local read "# of devices to test"() -> (w874:u32)
                                n1517 = Divide(x=w885, y=w877) -> (x/y=w884:dbl)
                                n1518 = Multiply(x=w893, y=100.0) -> (x*y=w872:dbl)
                                n1519 = Multiply(x=w891, y=100.0) -> (x*y=w871:dbl)
                                n1520 = local write "Std unit cost\n(cents/device)"(w872) -> ()
                                n1521 = local write "Tandem unit cost\n(cents/device)"(w871) -> ()
                                n1522 = Subtract(x=w872, y=w871) -> (x-y=w875:dbl)
                                n1523 = Multiply(x=w884, y=30) -> (x*y=w882:dbl)
                                n1524 = Multiply(x=w874, y=w875) -> (x*y=w873:dbl)
                                n1525 = local write "Calendar days required\nfor testing all units"(w882) -> ()
                                n1526 = local write "$ saved"(w873) -> ()
                                }
                                }
                                }
                                frame True {
                                n1527 = local read "H1 online"() -> (w924:bool)
                                n1528 = local read "Tandem\nfloorspace area"() -> (w936:i32)
                                n1529 = local read "Std cell \nfloorspace area"() -> (w929:i32)
                                n1530 = case shown="True" w924 {
                                tunnel: [0 w938] -> w904
                                frame False {
                                }
                                frame True {
                                n1531 = local read "H1 UPH"() -> (w939:cluster{u32, u32})
                                n1532 = Unbundle(w939) -> (w938:u32)  [unwired: 1 out]
                                }
                                }
                                n1533 = local read "System UPH"() -> (w935:u32)
                                n1534 = local read "H2 calc UPH"() -> (w930:dbl)
                                n1535 = Divide(x=w935, y=w936) -> (x/y=w907:dbl)
                                n1536 = Divide(x=w930, y=w929) -> (x/y=w908:dbl)
                                n1537 = local write "Tandem UPH\nper unit area"(w907) -> ()
                                n1538 = local write "H2 UPH per unit area"(w908) -> ()
                                n1539 = local read "Std hourly\ncost ($/hr)"() -> (w932:dbl)
                                n1540 = local read "H2 UPH"() -> (w934:cluster{u32, u32})
                                n1541 = local read "Utilization (%)"() -> (w914:u32)
                                n1542 = local read "Tandem hourly\ncost ($/hr)"() -> (w933:dbl)
                                n1543 = local read "# of devices to test"() -> (w920:u32)
                                n1544 = local read "Hours per month"() -> (w915:i32)
                                n1545 = Unbundle(w934) -> (w910:u32)  [unwired: 1 out]
                                n1546 = local write "Calc H1 UPH"(w904) -> ()
                                n1547 = local write "Calc H2 UPH"(w910) -> ()
                                n1548 = local read "UPH"() -> (w931:dbl)
                                n1549 = Add(x=w904, y=w910) -> (x+y=w909:u32)
                                n1550 = Divide(x=w914, y=u32 100) -> (x/y=w913:dbl)
                                n1551 = local write "System UPH"(w909) -> ()
                                n1552 = local write "Calc\nsystem UPH"(w909) -> ()
                                n1553 = Divide(x=w920, y=w909) -> (x/y=w919:dbl)
                                n1554 = Multiply(x=w915, y=w913) -> (x*y=w911:dbl)
                                n1555 = Divide(x=w932, y=w931) -> (x/y=w928:dbl)
                                n1556 = Divide(x=w933, y=w909) -> (x/y=w926:dbl)
                                n1557 = local read "# of devices to test"() -> (w922:u32)
                                n1558 = Divide(x=w919, y=w911) -> (x/y=w918:dbl)
                                n1559 = Multiply(x=w928, y=100.0) -> (x*y=w906:dbl)
                                n1560 = Multiply(x=w926, y=100.0) -> (x*y=w905:dbl)
                                n1561 = local write "Std unit cost\n(cents/device)"(w906) -> ()
                                n1562 = local write "Tandem unit cost\n(cents/device)"(w905) -> ()
                                n1563 = Subtract(x=w906, y=w905) -> (x-y=w923:dbl)
                                n1564 = Multiply(x=w918, y=30) -> (x*y=w916:dbl)
                                n1565 = Multiply(x=w922, y=w923) -> (x*y=w921:dbl)
                                n1566 = local write "Calendar days required\nfor testing all units"(w916) -> ()
                                n1567 = local write "$ saved"(w921) -> ()
                                }
                                }
                                }
                                frame #4 {
                                # "when this loop unlocks the handlers,\nthe handler interface loops are free to continue\nto send the binning information to their\nrespective handlers.  Each handler interface \nloop using the \"binning string hidden\" to do\nthis.  That is why, here, there is no writing of\nthe binning information to a handler.  \nThat is done in the handler interface loops."
                                n1568 = local write "H1 Lock"(FALSE ("H1 Lock")) -> ()
                                n1569 = local write "H2 Lock"(FALSE ("H1 Lock")) -> ()
                                }
                                frame #5 {
                                n1570 = local read "Tester online"() -> (w944:bool)
                                n1571 = local read "POWER"() -> (w946:bool)
                                n1572 = Compound Arithmetic op=AND(w944, w946) -> (w945:bool)
                                n1573 = case shown="True" w945 {
                                frame False {
                                n1574 = local write "SC virtual handler states"(SC_virtual_handler_states."closing bus" ("SC virtual handler states")) -> ()
                                }
                                frame True {
                                n1575 = local write "SC virtual handler states"(SC_virtual_handler_states."waiting on event" ("SC Test Interface States")) -> ()
                                }
                                }
                                }
                                }
                              }
                              frame "responding to unknown command" {
                                n1576 = flat-sequence {
                                frame #0 {
                                n1577 = local read "GPIB Bus 0 traffic"() -> (w957:string)
                                n1578 = Concatenate Strings(w957, "\r\n", "Bus 0 write: " ("string"), "unrecognized string") -> (w955:string)
                                n1579 = local write "GPIB Bus 0 traffic"(w955) -> ()
                                }
                                frame #1 {
                                n1580 = local write "SC virtual handler states"(SC_virtual_handler_states."waiting on event" ("SC Test Interface States")) -> ()
                                }
                                }
                              }
                              frame "closing bus" {
                                n1581 = flat-sequence {
                                frame #0 {
                                n1582 = local read "GPIB Bus 0 traffic"() -> (w964:string)
                                n1583 = Concatenate Strings(w964, "\r\n", "Bus 0 closing: " ("string")) -> (w962:string)
                                n1584 = local write "GPIB Bus 0 traffic"(w962) -> ()
                                }
                                frame #1 {
                                n1585 = local read "VISA bus 0 resource name out"() -> (w966:refnum<visa-resource-name>)
                                n1586 = local read "VISA bus 0 error out"() -> (w967:errorcluster)
                                n1587 = VISA Close(VISA resource name=w966, error in (no error)=w967) -> (error out=w965:errorcluster)
                                n1588 = Unbundle By Name(w965) -> ("status"=w968:bool)
                                n1589 = local write "VISA bus 0 close error"(w968) -> ()
                                }
                                frame #2 {
                                n1590 = local write "Exit virtual handler state machine hid"(TRUE ("Exit tester state machine hid")) -> ()
                                }
                                }
                              }
                            }
                          }
                          frame #1 {
                          }
                          frame #2 {
                            n1591 = local read "Slow for  Diagnostics"() -> (w972:bool)
                            n1592 = case shown="True" w972 {
                              frame False {
                              }
                              frame True {
                                n1593 = local read "GPIB wait time (ms)"() -> (w975:u32)
                                n1594 = Wait (ms)(milliseconds to wait=w975) -> ()  [unwired: 1 out]
                              }
                            }
                          }
                        }
                        n1595 = Wait (ms)(milliseconds to wait=u32 1) -> ()  [unwired: 1 out]
                        n1596 = local read "Exit virtual handler state machine hid"() -> (w521:bool)
                      }
                    }
                  }
                }
              }
              n1597 = Wait (ms)(milliseconds to wait=u32 5) -> ()  [unwired: 1 out]
              n1598 = local read "POWER"() -> (w508:bool)
            }
            n1599 = while {
              stop <- w1426 continue-if-true
              n1600 = local read "H1 online"() -> (w1427:bool)
              n1601 = case shown="True" w1427 {
                frame False {
                }
                frame True {
                  n1602 = flat-sequence {
                    frame #0 {
                      n1603 = local write "Exit virtual tester H1 state machine hid"(FALSE ("Exit H1 state machine hid")) -> ()
                      n1604 = local write "SC virtual tester 1 states"(SC_virtual_tester_states."initializing bus" ("SC virtual tester states")) -> ()
                    }
                    frame #1 {
                      n1605 = while {
                        stop <- w1431 stop-if-true
                        n1606 = flat-sequence {
                          frame #0 {
                            n1607 = local read "SC virtual tester 1 states"() -> (w1433:T2)
                            n1608 = case shown="\"sending *IDN?\"" w1433 {
                              frame "initializing bus", Default {
                                n1609 = flat-sequence {
                                frame #0 {
                                # "bus 1"
                                n1610 = local read "GPIB wait timeout hid"() -> (w1435:u32)
                                n1611 = local read "SentCtrl talks to handler 1 at"() -> (w1436:refnum<visa-resource-name>)
                                n1612 = local read "GPIB wait timeout hid"() -> (w1434:u32)
                                n1613 = VISA Open(timeout (0)=w1435, VISA resource name=w1436) -> (VISA resource name=w1440:refnum<visa-resource-name>, error out=w1439:errorcluster)  [unwired: 3 in]
                                "VISA bus 1 resource name out" <- w1440
                                n1614 = property class="GPIB Instr"(reference=w1440, error in=w1439, "Timeout"=w1434) -> (error out=w1438:errorcluster)  [unwired: 1 out]
                                "VISA bus 1 error out" <- w1438
                                n1615 = Unbundle By Name(w1438) -> ("status"=w1437:bool)
                                n1616 = local write "VISA bus 1 open error"(w1437) -> ()
                                }
                                frame #1 {
                                n1617 = local write "SC virtual tester 1 states"(SC_virtual_tester_states."sending *IDN?" ("SC virtual tester states")) -> ()
                                n1618 = Concatenate Strings("Bus 1 initializing" ("string"), "\r\n") -> (w1442:string)
                                n1619 = local write "GPIB bus 1 traffic"(w1442) -> ()
                                }
                                frame #2 {
                                n1620 = local write "Exit virtual tester H1 state machine hid"(FALSE ("Exit H1 state machine hid")) -> ()
                                }
                                }
                              }
                              frame "sending *IDN?" {
                                n1621 = flat-sequence {
                                tunnel: [w1455] -> w1448
                                tunnel: [w1454] -> w1447
                                tunnel: w1448 -> [w1470]
                                tunnel: w1447 -> [w1469]
                                tunnel: [w1466] -> w1446
                                tunnel: w1446 -> [w1473]
                                frame #0 {
                                w1449 = "*IDN?"
                                n1622 = local read "VISA bus 1 resource name out"() -> (w1458:refnum<visa-resource-name>)
                                n1623 = local read "GPIB bus 1 traffic"() -> (w1453:string)
                                n1624 = local read "VISA bus 1 error out"() -> (w1457:errorcluster)
                                n1625 = Concatenate Strings(w1453, "\r\n", "Bus 1 write: " ("string"), w1449) -> (w1451:string)
                                n1626 = VISA Write(VISA resource name=w1458, write buffer=w1449, error in (no error)=w1457) -> (VISA resource name out=w1455:refnum<visa-resource-name>, error out=w1454:errorcluster)  [unwired: 1 out]
                                n1627 = Unbundle By Name(w1454) -> ("status"=w1456:bool)
                                n1628 = local write "GPIB bus 1 traffic"(w1451) -> ()
                                n1629 = local write "GPIB bus 1 write error"(w1456) -> ()
                                }
                                frame #1 {
                                n1630 = local read "GPIB bus 1 traffic"() -> (w1460:string)
                                n1631 = VISA Read(VISA resource name=w1470, byte count=u32 256, error in (no error)=w1469) -> (VISA resource name out=w1467:refnum<visa-resource-name>, read buffer=w1459:string, return count=w1466:u32, error out=w1464:errorcluster)
                                n1632 = local write "VISA bus 1 resource name out"(w1467) -> ()
                                n1633 = Unbundle By Name(w1464) -> ("status"=w1465:bool)
                                n1634 = local write "GPIB bus 1 read error"(w1465) -> ()
                                n1635 = Concatenate Strings(w1460, "\r\n", "Bus 1 read: " ("string"), w1459) -> (w1462:string)
                                n1636 = local write "GPIB bus 1 traffic"(w1462) -> ()
                                }
                                frame #2 {
                                n1637 = Greater?(x=w1473, y=u32 0) -> (0:w1471:bool)
                                n1638 = case shown="False" w1471 {
                                frame False {
                                n1639 = local write "SC virtual tester 1 states"(SC_virtual_tester_states."sending *IDN?" ("SC virtual tester states")) -> ()
                                n1640 = local write "H1 online"(FALSE ("H1 online")) -> ()
                                n1641 = One Button Dialog(message="Warning:\nVirtual tester does not get a response\nto *IDN? from handler 1.\nCheck GPIB cable and that  handler 1 \nis running and ready to issue a start of test\nby responding with sites ready.", button name ("OK")="Dismiss and retry") -> ()  [unwired: 1 out]
                                }
                                frame True {
                                n1642 = local write "SC virtual tester 1 states"(SC_virtual_tester_states."sending *IDN?" ("SC virtual tester states")) -> ()
                                }
                                }
                                }
                                }
                              }
                              frame "sending *IDN?" {
                                n1643 = flat-sequence {
                                tunnel: [w1482] -> w1480
                                tunnel: [w1481] -> w1479
                                tunnel: w1480 -> [w1518]
                                tunnel: w1479 -> [w1517]
                                frame #0 {
                                n1644 = while {
                                tunnel: [w1486] -> w1482
                                tunnel: [w1484] -> w1481
                                stop <- w1483 stop-if-true
                                n1645 = stacked-sequence {
                                tunnel: [w1498] -> w1488
                                tunnel: [w1497] -> w1487
                                frame #0 {
                                w1490 = "*SITES?"
                                n1646 = local read "VISA bus 1 resource name out"() -> (w1496:refnum<visa-resource-name>)
                                n1647 = local read "VISA bus 1 error out"() -> (w1495:errorcluster)
                                n1648 = Concatenate Strings("Handler 1 cycle start" ("string"), "\r\n", "Bus 1 write: " ("string"), w1490) -> (w1492:string)
                                n1649 = VISA Write(VISA resource name=w1496, write buffer=w1490, error in (no error)=w1495) -> (VISA resource name out=w1498:refnum<visa-resource-name>, error out=w1497:errorcluster)  [unwired: 1 out]
                                n1650 = Unbundle By Name(w1497) -> ("status"=w1494:bool)
                                n1651 = local write "GPIB bus 1 traffic"(w1492) -> ()
                                n1652 = local write "GPIB bus 1 write error"(w1494) -> ()
                                }
                                }
                                n1653 = Wait (ms)(milliseconds to wait=u32 1) -> ()  [unwired: 1 out]
                                n1654 = flat-sequence {
                                tunnel: w1488 -> [w1516]
                                tunnel: w1487 -> [w1515]
                                tunnel: [w1503] -> w1486
                                tunnel: [w1499] -> w1484
                                tunnel: [w1500] -> w1483
                                frame #0 {
                                n1655 = local read "GPIB bus 1 traffic"() -> (w1508:string)
                                n1656 = VISA Read(VISA resource name=w1516, byte count=u32 256, error in (no error)=w1515) -> (read buffer=w1503:string, error out=w1502:errorcluster)  [unwired: 2 out]
                                n1657 = Unbundle By Name(w1502) -> ("status"=w1499:bool)
                                n1658 = String Length(string=w1503) -> (length=w1505:i32)
                                n1659 = Scan Value(string=w1503, format string="%b", default (0 dbl)=u8 0) -> (value=w1507:u8)  [unwired: 1 out]
                                n1660 = Concatenate Strings(w1508, "\r\n", "Bus 1 read: " ("string"), w1503) -> (w1510:string)
                                n1661 = local write "GPIB bus 1 read error"(w1499) -> ()
                                n1662 = Greater Than 0?(x=w1505) -> (x > 0?=w1504:bool)
                                n1663 = Greater Than 0?(x=w1507) -> (x > 0?=w1506:bool)
                                n1664 = local write "GPIB bus 1 traffic"(w1510) -> ()
                                n1665 = And(x=w1504, y=w1506) -> (x .and. y?=w1501:bool)
                                n1666 = Or(x=w1501, y=w1499) -> (x .or. y?=w1500:bool)
                                }
                                }
                                }
                                }
                                frame #1 {
                                n1667 = case shown="True" w1517 {
                                tunnel: w1518 -> [w1519 _]
                                frame False {
                                n1668 = flat-sequence {
                                tunnel: w1519 -> [w1520]
                                frame #0 {
                                n1669 = String Length(string=w1520) -> (length=w1521:i32)
                                n1670 = local write "H1 sites ready hidden"(w1520) -> ()
                                n1671 = local write "H1 parallelism"(w1521) -> ()
                                }
                                frame #1 {
                                # "This block adds zeroes (sites not ready)\nto SITES READY from handlers when the\nhandler is running at a lower parallelism\nthan the test program, but has the same\npin mapping for the active sites in common."
                                n1672 = local read "Program Parallelism"() -> (w1525:u32)
                                n1673 = local read "H1 allow lower parallelism"() -> (w1524:bool)
                                n1674 = local read "H1 parallelism"() -> (w1526:u32)
                                n1675 = Less?(x=w1526, y=w1525) -> (x < y?=w1523:bool)
                                n1676 = And(x=w1523, y=w1524) -> (x .and. y?=w1522:bool)
                                n1677 = case shown="False" w1522 {
                                frame False {
                                n1678 = local read "Program Parallelism"() -> (w1529:u32)
                                n1679 = local read "H1 parallelism"() -> (w1527:u32)
                                n1680 = Greater?(x=w1527, y=w1529) -> (0:w1528:bool)
                                n1681 = case shown="True" w1528 {
                                frame False {
                                # "parallelisms must match if arriving here"
                                n1682 = local write "SC virtual tester 1 states"(SC_virtual_tester_states."sending HAND?" ("SC virtual tester states")) -> ()
                                }
                                frame True {
                                n1683 = local write "SC virtual tester 1 states"(SC_virtual_tester_states."closing bus" ("SC virtual tester states")) -> ()
                                n1684 = local write "POWER"(FALSE ("POWER")) -> ()
                                n1685 = One Button Dialog(message="Fatal error 300:\nTest program cannot support higher\nparallelism on handler 1.\nThe Sentinel Controller program is shutting down.\nPlease correct the mismatch and restart.") -> ()  [unwired: 1 in, 1 out]
                                }
                                }
                                }
                                frame True {
                                n1686 = local read "Program Parallelism"() -> (w1539:u32)
                                n1687 = local read "H1 parallelism"() -> (w1536:u32)
                                n1688 = local read "H1 sites ready hidden"() -> (w1537:string)
                                n1689 = Subtract(x=w1539, y=w1536) -> (x-y=w1538:u32)
                                n1690 = for {
                                N: w1538 -> [_]
                                shift-right: [w1540] -> w1534
                                shift-left: w1537 -> [w1541]
                                n1691 = Concatenate Strings(w1541, "0" ("string")) -> (w1540:string)
                                }
                                n1692 = local write "H1 sites ready hidden"(w1534) -> ()
                                n1693 = local write "SC virtual tester 1 states"(SC_virtual_tester_states."sending HAND?" ("SC virtual tester states")) -> ()
                                }
                                }
                                }
                                frame #2 {
                                n1694 = Tick Count (ms)() -> (millisecond timer value=w1547:u32)
                                n1695 = Tick Count (ms)() -> (millisecond timer value=w1546:u32)
                                n1696 = local write "H1 Ready with sites"(TRUE ("H2 Waiting")) -> ()
                                n1697 = local write "H1 wt start hidden"(w1547) -> ()
                                n1698 = local write "H1 it end hidden"(w1546) -> ()
                                n1699 = local write "H1 Indexing"(FALSE ("h1 indexing")) -> ()
                                n1700 = local write "H1 Testing"(FALSE ("h1 indexing")) -> ()
                                }
                                frame #3 {
                                n1701 = local read "H1 it start hidden"() -> (w1551:u32)
                                n1702 = local read "H1 it end hidden"() -> (w1552:u32)
                                n1703 = Subtract(x=w1552, y=w1551) -> (x-y=w1548:u32)
                                n1704 = Divide(x=w1548, y=u32 1000) -> (x/y=w1550:dbl)
                                n1705 = local write "H1 measured Index Time"(w1550) -> ()
                                n1706 = local write "SC virtual tester 1 states"(SC_virtual_tester_states."sending HAND?" ("SC virtual tester states")) -> ()
                                }
                                }
                                }
                                frame True {
                                n1707 = flat-sequence {
                                frame #0 {
                                n1708 = local read "VISA bus 1 resource name out"() -> (w1556:refnum<visa-resource-name>)
                                n1709 = local read "VISA bus 1 error out"() -> (w1557:errorcluster)
                                n1710 = VISA Close(VISA resource name=w1556, error in (no error)=w1557) -> (error out=w1555:errorcluster)
                                n1711 = Unbundle By Name(w1555) -> ("status"=w1554:bool)
                                n1712 = local write "VISA bus 1 close error"(w1554) -> ()
                                }
                                frame #1 {
                                n1713 = local write "VISA bus 1 close error"(FALSE ("VISA bus 1 close error")) -> ()
                                n1714 = Concatenate Strings("Bus 1 error  while reading,\nclosing Bus 1 and re-initializing" ("string"), "\r\n") -> (w1560:string)
                                n1715 = local write "GPIB bus 1 traffic"(w1560) -> ()
                                }
                                frame #2 {
                                n1716 = local write "SC virtual tester 1 states"(SC_virtual_tester_states."initializing bus" ("SC virtual tester states")) -> ()
                                }
                                }
                                }
                                }
                                }
                                }
                              }
                              frame "sending HAND?" {
                                n1717 = flat-sequence {
                                tunnel: [w1566] -> w1564
                                tunnel: [w1565] -> w1563
                                tunnel: w1564 -> [w1576]
                                tunnel: w1563 -> [w1575]
                                frame #0 {
                                w1574 = "*HAND?"
                                n1718 = local read "VISA bus 1 resource name out"() -> (w1567:refnum<visa-resource-name>)
                                n1719 = local read "GPIB bus 1 traffic"() -> (w1570:string)
                                n1720 = local read "VISA bus 1 error out"() -> (w1568:errorcluster)
                                n1721 = Concatenate Strings(w1570, "\r\n", "Bus 1 write: " ("string"), w1574) -> (w1572:string)
                                n1722 = VISA Write(VISA resource name=w1567, write buffer=w1574, error in (no error)=w1568) -> (VISA resource name out=w1566:refnum<visa-resource-name>, error out=w1565:errorcluster)  [unwired: 1 out]
                                n1723 = Unbundle By Name(w1565) -> ("status"=w1569:bool)
                                n1724 = local write "GPIB bus 1 traffic"(w1572) -> ()
                                n1725 = local write "GPIB bus 1 write error"(w1569) -> ()
                                }
                                frame #1 {
                                n1726 = local read "GPIB bus 1 traffic"() -> (w1578:string)
                                n1727 = VISA Read(VISA resource name=w1576, byte count=u32 256, error in (no error)=w1575) -> (read buffer=w1577:string, error out=w1583:errorcluster)  [unwired: 2 out]
                                n1728 = local write "H1 response to *HAND? hidden"(w1577) -> ()
                                n1729 = Unbundle By Name(w1583) -> ("status"=w1582:bool)
                                n1730 = local write "GPIB bus 1 read error"(w1582) -> ()
                                n1731 = Concatenate Strings(w1578, "\r\n", "Bus 1 read: " ("string"), w1577) -> (w1580:string)
                                n1732 = local write "GPIB bus 1 traffic"(w1580) -> ()
                                }
                                frame #2 {
                                n1733 = local write "SC virtual tester 1 states"(SC_virtual_tester_states."testing" ("SC virtual tester states")) -> ()
                                }
                                }
                              }
                              frame "testing" {
                                n1734 = flat-sequence {
                                frame #0 {
                                n1735 = while {
                                stop <- w1586 stop-if-true
                                n1736 = local read "H1 Lock"() -> (w1586:bool)
                                n1737 = Wait (ms)(milliseconds to wait=u32 1) -> ()  [unwired: 1 out]
                                }
                                }
                                frame #1 {
                                n1738 = Tick Count (ms)() -> (millisecond timer value=w1597:u32)
                                n1739 = Tick Count (ms)() -> (millisecond timer value=w1596:u32)
                                n1740 = local write "H1 Testing"(TRUE ("testing")) -> ()
                                n1741 = local write "H1 Ready with sites"(FALSE ("H1 Waiting")) -> ()
                                n1742 = local write "H1 Indexing"(FALSE ("waiting")) -> ()
                                n1743 = local write "H1 wt end hidden"(w1597) -> ()
                                n1744 = local write "H1 tt start hidden"(w1596) -> ()
                                n1745 = local read "GPIB bus 1 traffic"() -> (w1589:string)
                                n1746 = local write "SC virtual tester 1 states"(SC_virtual_tester_states."binning" ("SC virtual tester states")) -> ()
                                n1747 = Concatenate Strings(w1589, "\r\n", "Bus 1: " ("string"), "testing" ("string")) -> (w1591:string)
                                n1748 = local write "GPIB bus 1 traffic"(w1591) -> ()
                                }
                                frame #2 {
                                n1749 = local read "H1 wt start hidden"() -> (w1602:u32)
                                n1750 = local read "H1 wt end hidden"() -> (w1603:u32)
                                n1751 = Subtract(x=w1603, y=w1602) -> (x-y=w1601:u32)
                                n1752 = Divide(x=w1601, y=u32 1000) -> (x/y=w1599:dbl)
                                n1753 = local write "H1 measured Wait Time"(w1599) -> ()
                                }
                                }
                              }
                              frame "binning" {
                                n1754 = flat-sequence {
                                tunnel: [w1615] -> w1606
                                tunnel: [w1642] -> w1607
                                tunnel: w1606 -> [w1642]
                                tunnel: w1607 -> [w1649]
                                tunnel: [w1648] -> w1605
                                tunnel: [w1647] -> w1604
                                tunnel: w1605 -> [w1700]
                                tunnel: w1604 -> [w1699]
                                frame #0 {
                                n1755 = while {
                                stop <- w1609 continue-if-true
                                n1756 = local read "H1 Lock"() -> (w1609:bool)
                                n1757 = Wait (ms)(milliseconds to wait=u32 1) -> ()  [unwired: 1 out]
                                }
                                }
                                frame #1 {
                                n1758 = local read "Program Parallelism"() -> (w1613:u32)
                                n1759 = local read "H1 parallelism"() -> (w1614:u32)
                                n1760 = Less?(x=w1614, y=w1613) -> (x < y?=w1611:bool)
                                n1761 = local read "H1 allow lower parallelism"() -> (w1612:bool)
                                n1762 = And(x=w1611, y=w1612) -> (x .and. y?=w1610:bool)
                                n1763 = case shown="False" w1610 {
                                tunnel: [w1616 w1627] -> w1615
                                frame False {
                                n1764 = local read "VISA bus 1 resource name out"() -> (w1624:refnum<visa-resource-name>)
                                n1765 = local read "Binning_string hidden"() -> (w1616:string)
                                n1766 = local read "VISA bus 1 error out"() -> (w1625:errorcluster)
                                n1767 = local read "GPIB bus 1 traffic"() -> (w1620:string)
                                n1768 = VISA Write(VISA resource name=w1624, write buffer=w1616, error in (no error)=w1625) -> (VISA resource name out=w1622:refnum<visa-resource-name>, error out=w1623:errorcluster)  [unwired: 1 out]
                                n1769 = local write "VISA bus 1 resource name out"(w1622) -> ()
                                n1770 = local write "VISA bus 1 error out"(w1623) -> ()
                                n1771 = Unbundle By Name(w1623) -> ("status"=w1621:bool)
                                n1772 = Concatenate Strings(w1620, "\r\n", "Bus 1 write: " ("string"), w1616) -> (w1618:string)
                                n1773 = local write "GPIB bus 1 write error"(w1621) -> ()
                                n1774 = local write "GPIB bus 1 traffic"(w1618) -> ()
                                }
                                frame True {
                                n1775 = local read "H1 parallelism"() -> (w1626:u32)
                                n1776 = local read "Binning_string hidden"() -> (w1628:string)
                                n1777 = local read "VISA bus 1 resource name out"() -> (w1639:refnum<visa-resource-name>)
                                n1778 = local read "VISA bus 1 error out"() -> (w1640:errorcluster)
                                n1779 = Multiply(x=w1626, y=u32 8) -> (x*y=w1630:u32)
                                n1780 = local read "GPIB bus 1 traffic"() -> (w1635:string)
                                n1781 = Decrement(x=w1630) -> (x-1=w1631:u32)
                                n1782 = String Subset(string=w1628, length (rest)=w1631) -> (substring=w1627:string)  [unwired: 1 in]
                                n1783 = VISA Write(VISA resource name=w1639, write buffer=w1627, error in (no error)=w1640) -> (VISA resource name out=w1637:refnum<visa-resource-name>, error out=w1638:errorcluster)  [unwired: 1 out]
                                n1784 = local write "VISA bus 1 resource name out"(w1637) -> ()
                                n1785 = local write "VISA bus 1 error out"(w1638) -> ()
                                n1786 = Unbundle By Name(w1638) -> ("status"=w1636:bool)
                                n1787 = Concatenate Strings(w1635, "\r\n", "Bus 1 write: " ("string"), w1627) -> (w1633:string)
                                n1788 = local write "GPIB bus 1 traffic"(w1633) -> ()
                                n1789 = local write "GPIB bus 1 write error"(w1636) -> ()
                                }
                                }
                                }
                                frame #2 {
                                n1790 = local write "H1 Ready with sites"(FALSE ("waiting")) -> ()
                                n1791 = Tick Count (ms)() -> (millisecond timer value=w1643:u32)
                                n1792 = Tick Count (ms)() -> (millisecond timer value=w1644:u32)
                                n1793 = local write "H1 tt end hidden"(w1643) -> ()
                                n1794 = local write "H1 it start hidden"(w1644) -> ()
                                n1795 = local write "H1 Indexing"(TRUE ("waiting")) -> ()
                                n1796 = local write "H1 Testing"(FALSE ("waiting")) -> ()
                                }
                                frame #3 {
                                n1797 = local read "H1 tt start hidden"() -> (w1653:u32)
                                n1798 = while {
                                tunnel: [w1672] -> w1668 mode=indexing
                                shift-right: [w1673] -> _
                                shift-left: w1649 -> [w1675]
                                stop <- w1670 stop-if-true
                                n1799 = Match Pattern(string=w1675, regular expression=" ") -> (before substring=w1672:string, after substring=w1673:string, offset past match=w1671:i32)  [unwired: 2 out]
                                n1800 = Less Than 0?(x=w1671) -> (x < 0?=w1670:bool)
                                }
                                n1801 = local read "H1 tt end hidden"() -> (w1654:u32)
                                n1802 = Subtract(x=w1654, y=w1653) -> (x-y=w1652:u32)
                                n1803 = Divide(x=w1652, y=u32 1000) -> (x/y=w1650:dbl)
                                n1804 = local write "H1 measured Test Time"(w1650) -> ()
                                n1805 = Array Size(array=w1668) -> (size(s)=w1665:i32)
                                n1806 = Divide(x=w1665, y=3) -> (x/y=w1667:dbl)
                                n1807 = To Unsigned Byte Integer(number=w1667) -> (unsigned 8bit integer=w1663:u8)
                                n1808 = local read "H1 sites ready hidden"() -> (w1660:string)
                                n1809 = local read "H1 parallelism"() -> (w1659:u32)
                                n1810 = Not Equal?(x=w1659, y=w1663) -> (x != y?=w1664:bool)
                                n1811 = for {
                                N: w1663 -> [_]
                                tunnel: w1668 -> [w1698]
                                tunnel: w1660 -> [w1689]
                                shift-right: [w1682] -> w1647
                                shift-left: 0 -> [w1681]
                                shift-right: [w1678] -> w1648
                                shift-left: 0 -> [w1676]
                                i -> [w1679]
                                n1812 = Increment(x=w1676) -> (x+1=w1677:i32)
                                n1813 = Increment(x=w1681) -> (x+1=w1680:i32)
                                n1814 = Increment(x=w1679) -> (x+1=w1697:i32)
                                n1815 = String Subset(string=w1689, offset (0)=w1679, length (rest)=1 ("length (rest)")) -> (substring=w1685:string)
                                n1816 = Multiply(x=3, y=w1697) -> (x*y=w1691:i32)
                                n1817 = Equal?(x=w1685, y="1") -> (x = y?=w1683:bool)
                                n1818 = Decrement(x=w1691) -> (x-1=w1690:i32)
                                n1819 = Select(t=w1680, s=w1683, f=w1681) -> (s? t:f=w1682:i32)
                                n1820 = Index Array(array=w1698, index=w1690) -> (element=w1695:string)
                                n1821 = Decimal String To Number(string=w1695, offset=0) -> (number=w1693:i32)  [unwired: 1 in, 1 out]
                                n1822 = Equal?(x=w1693, y=1) -> (x = y?=w1686:bool)
                                n1823 = And(x=w1686, y=w1683) -> (x .and. y?=w1687:bool)
                                n1824 = Select(t=w1677, s=w1687, f=w1676) -> (s? t:f=w1678:i32)
                                }
                                n1825 = case shown="True" w1664 {
                                frame False {
                                }
                                frame True {
                                n1826 = One Button Dialog(message="Warning:\nH1 Parallelism Mismatch!\nEither allow this from the system configuration tab\nor change the parallelism on H2. This message will\ncontinue until the problem is corrected.") -> ()  [unwired: 1 in, 1 out]
                                }
                                }
                                n1827 = local read "H1 Device Count"() -> (w1656:u32)
                                n1828 = local read "H1 Good Units"() -> (w1657:u32)
                                n1829 = Add(x=w1657, y=w1648) -> (x+y=w1658:u32)
                                n1830 = Add(x=w1656, y=w1647) -> (x+y=w1655:u32)
                                n1831 = local write "H1 Good Units"(w1658) -> ()
                                n1832 = local write "H1 Device Count"(w1655) -> ()
                                }
                                frame #4 {
                                n1833 = local read "H1 Device Count"() -> (w1704:u32)
                                n1834 = Divide(x=w1700, y=w1699) -> (x/y=w1701:dbl)
                                n1835 = local read "H1 Good Units"() -> (w1705:u32)
                                n1836 = Multiply(x=w1701, y=100.0) -> (x*y=w1703:dbl)
                                n1837 = Divide(x=w1705, y=w1704) -> (x/y=w1708:dbl)
                                n1838 = local write "H1 cycle yield hid"(w1703) -> ()
                                n1839 = Multiply(x=w1708, y=100.0) -> (x*y=w1706:dbl)
                                n1840 = local write "H1 lot yield mon"(w1706) -> ()
                                }
                                frame #5 {
                                n1841 = local read "H1 online"() -> (w1709:bool)
                                n1842 = local read "POWER"() -> (w1710:bool)
                                n1843 = Compound Arithmetic op=AND(w1709, w1710) -> (w1711:bool)
                                n1844 = case shown="True" w1711 {
                                frame False {
                                n1845 = local write "SC virtual tester 1 states"(SC_virtual_tester_states."closing bus" ("SC virtual tester states")) -> ()
                                }
                                frame True {
                                n1846 = local write "SC virtual tester 1 states"(SC_virtual_tester_states."sending *IDN?" ("SC virtual tester states")) -> ()
                                }
                                }
                                }
                                }
                              }
                              frame "closing bus" {
                                n1847 = local read "GPIB bus 1 traffic"() -> (w1718:string)
                                n1848 = local write "Exit virtual tester H1 state machine hid"(TRUE ("Exit H1 state machine hid")) -> ()
                                n1849 = local read "VISA bus 1 resource name out"() -> (w1722:refnum<visa-resource-name>)
                                n1850 = local read "VISA bus 1 error out"() -> (w1721:errorcluster)
                                n1851 = Concatenate Strings(w1718, "\r\n", "Bus 1: closing " ("string")) -> (w1716:string)
                                n1852 = local write "GPIB bus 1 traffic"(w1716) -> ()
                                n1853 = VISA Close(VISA resource name=w1722, error in (no error)=w1721) -> (error out=w1720:errorcluster)
                                n1854 = Unbundle By Name(w1720) -> ("status"=w1719:bool)
                                n1855 = local write "VISA bus 1 close error"(w1719) -> ()
                              }
                            }
                          }
                          frame #1 {
                            n1856 = local read "Slow for  Diagnostics"() -> (w1723:bool)
                            n1857 = case shown="True" w1723 {
                              frame False {
                              }
                              frame True {
                                n1858 = local read "GPIB wait time (ms)"() -> (w1724:u32)
                                n1859 = Wait (ms)(milliseconds to wait=w1724) -> ()  [unwired: 1 out]
                              }
                            }
                          }
                        }
                        n1860 = Wait (ms)(milliseconds to wait=u32 1) -> ()  [unwired: 1 out]
                        n1861 = local read "Exit virtual tester H1 state machine hid"() -> (w1431:bool)
                      }
                    }
                  }
                }
              }
              n1862 = Wait (ms)(milliseconds to wait=u32 5) -> ()  [unwired: 1 out]
              n1863 = local read "POWER"() -> (w1426:bool)
            }
            n1864 = while {
              stop <- w976 continue-if-true
              n1865 = local read "H2 online"() -> (w977:bool)
              n1866 = case shown="True" w977 {
                frame False {
                }
                frame True {
                  n1867 = flat-sequence {
                    frame #0 {
                      n1868 = local write "Exit virtual tester H2 state machine hid"(FALSE ("Exit H2 state machine hid")) -> ()
                      n1869 = local write "SC virtual tester 2 states"(SC_virtual_tester_states."initializing bus" ("SC virtual tester states")) -> ()
                    }
                    frame #1 {
                      n1870 = while {
                        stop <- w981 stop-if-true
                        n1871 = flat-sequence {
                          frame #0 {
                            n1872 = local read "SC virtual tester 2 states"() -> (w983:T2)
                            n1873 = case shown="\"sending *IDN?\"" w983 {
                              frame "initializing bus", Default {
                                n1874 = flat-sequence {
                                frame #0 {
                                # "bus 2"
                                n1875 = local read "GPIB wait timeout hid"() -> (w984:u32)
                                n1876 = local read "SentCtrl talks to handler 2 at"() -> (w986:refnum<visa-resource-name>)
                                n1877 = local read "GPIB wait timeout hid"() -> (w985:u32)
                                n1878 = VISA Open(timeout (0)=w984, VISA resource name=w986) -> (VISA resource name=w990:refnum<visa-resource-name>, error out=w989:errorcluster)  [unwired: 3 in]
                                "VISA bus 2 resource name out" <- w990
                                n1879 = property class="GPIB Instr"(reference=w990, error in=w989, "Timeout"=w985) -> (error out=w988:errorcluster)  [unwired: 1 out]
                                "VISA bus 2 error out" <- w988
                                n1880 = Unbundle By Name(w988) -> ("status"=w987:bool)
                                n1881 = local write "VISA bus 2 open error"(w987) -> ()
                                }
                                frame #1 {
                                n1882 = local write "SC virtual tester 2 states"(SC_virtual_tester_states."sending *IDN?" ("SC virtual tester states")) -> ()
                                n1883 = Concatenate Strings("Bus 2 initializing" ("string"), "\r\n") -> (w992:string)
                                n1884 = local write "GPIB bus 2 traffic"(w992) -> ()
                                }
                                frame #2 {
                                n1885 = local write "Exit virtual tester H2 state machine hid"(FALSE ("Exit H2 state machine hid")) -> ()
                                }
                                }
                              }
                              frame "sending *IDN?" {
                                n1886 = flat-sequence {
                                tunnel: [w1005] -> w998
                                tunnel: [w1004] -> w997
                                tunnel: w998 -> [w1020]
                                tunnel: w997 -> [w1019]
                                tunnel: [w1016] -> w996
                                tunnel: w996 -> [w1023]
                                frame #0 {
                                w999 = "*IDN?"
                                n1887 = local read "VISA bus 2 resource name out"() -> (w1008:refnum<visa-resource-name>)
                                n1888 = local read "GPIB bus 2 traffic"() -> (w1003:string)
                                n1889 = local read "VISA bus 2 error out"() -> (w1007:errorcluster)
                                n1890 = Concatenate Strings(w1003, "\r\n", "Bus 2 write: " ("string"), w999) -> (w1001:string)
                                n1891 = VISA Write(VISA resource name=w1008, write buffer=w999, error in (no error)=w1007) -> (VISA resource name out=w1005:refnum<visa-resource-name>, error out=w1004:errorcluster)  [unwired: 1 out]
                                n1892 = local write "GPIB bus 2 traffic"(w1001) -> ()
                                n1893 = Unbundle By Name(w1004) -> ("status"=w1006:bool)
                                n1894 = local write "GPIB bus 2 write error"(w1006) -> ()
                                }
                                frame #1 {
                                n1895 = local read "GPIB bus 2 traffic"() -> (w1010:string)
                                n1896 = VISA Read(VISA resource name=w1020, byte count=u32 256, error in (no error)=w1019) -> (VISA resource name out=w1017:refnum<visa-resource-name>, read buffer=w1009:string, return count=w1016:u32, error out=w1014:errorcluster)
                                n1897 = local write "VISA bus 2 resource name out"(w1017) -> ()
                                n1898 = Unbundle By Name(w1014) -> ("status"=w1015:bool)
                                n1899 = local write "GPIB bus 2 read error"(w1015) -> ()
                                n1900 = Concatenate Strings(w1010, "\r\n", "Bus 2 read: " ("string"), w1009) -> (w1012:string)
                                n1901 = local write "GPIB bus 2 traffic"(w1012) -> ()
                                }
                                frame #2 {
                                n1902 = Greater?(x=w1023, y=u32 0) -> (0:w1021:bool)
                                n1903 = case shown="False" w1021 {
                                frame False {
                                n1904 = local write "SC virtual tester 2 states"(SC_virtual_tester_states."sending *IDN?" ("SC virtual tester states")) -> ()
                                n1905 = local write "H2 online"(FALSE ("H2 online")) -> ()
                                n1906 = One Button Dialog(message="Warning:\nVirtual tester does not get a response\nto *IDN? from handler 2.\nCheck GPIB cable and that  handler 2 \nis running and ready to issue a start of test\nby responding with sites ready.", button name ("OK")="Dismiss and retry") -> ()  [unwired: 1 out]
                                }
                                frame True {
                                n1907 = local write "SC virtual tester 2 states"(SC_virtual_tester_states."sending *IDN?" ("SC virtual tester states")) -> ()
                                }
                                }
                                }
                                }
                              }
                              frame "sending *IDN?" {
                                n1908 = flat-sequence {
                                tunnel: [w1032] -> w1030
                                tunnel: [w1031] -> w1029
                                tunnel: w1030 -> [w1068]
                                tunnel: w1029 -> [w1067]
                                frame #0 {
                                n1909 = while {
                                tunnel: [w1036] -> w1032
                                tunnel: [w1033] -> w1031
                                stop <- w1035 stop-if-true
                                n1910 = stacked-sequence {
                                tunnel: [w1048] -> w1038
                                tunnel: [w1047] -> w1037
                                frame #0 {
                                w1043 = "*SITES?"
                                n1911 = local read "VISA bus 2 resource name out"() -> (w1040:refnum<visa-resource-name>)
                                n1912 = local read "VISA bus 2 error out"() -> (w1039:errorcluster)
                                n1913 = Concatenate Strings("Handler 2 cycle start" ("string"), "\r\n", "Bus 2 write: " ("string"), w1043) -> (w1045:string)
                                n1914 = VISA Write(VISA resource name=w1040, write buffer=w1043, error in (no error)=w1039) -> (VISA resource name out=w1048:refnum<visa-resource-name>, error out=w1047:errorcluster)  [unwired: 1 out]
                                n1915 = Unbundle By Name(w1047) -> ("status"=w1041:bool)
                                n1916 = local write "GPIB bus 2 traffic"(w1045) -> ()
                                n1917 = local write "GPIB bus 2 write error"(w1041) -> ()
                                }
                                }
                                n1918 = Wait (ms)(milliseconds to wait=u32 1) -> ()  [unwired: 1 out]
                                n1919 = flat-sequence {
                                tunnel: w1038 -> [w1066]
                                tunnel: w1037 -> [w1065]
                                tunnel: [w1052] -> w1036
                                tunnel: [w1050] -> w1035
                                tunnel: [w1049] -> w1033
                                frame #0 {
                                n1920 = local read "GPIB bus 2 traffic"() -> (w1057:string)
                                n1921 = VISA Read(VISA resource name=w1066, byte count=u32 256, error in (no error)=w1065) -> (read buffer=w1052:string, error out=w1063:errorcluster)  [unwired: 2 out]
                                n1922 = Unbundle By Name(w1063) -> ("status"=w1049:bool)
                                n1923 = String Length(string=w1052) -> (length=w1054:i32)
                                n1924 = Scan Value(string=w1052, format string="%b", default (0 dbl)=u8 0) -> (value=w1056:u8)  [unwired: 1 out]
                                n1925 = Concatenate Strings(w1057, "\r\n", "Bus 2 read: " ("string"), w1052) -> (w1059:string)
                                n1926 = local write "GPIB bus 2 read error"(w1049) -> ()
                                n1927 = Greater Than 0?(x=w1054) -> (x > 0?=w1053:bool)
                                n1928 = Greater Than 0?(x=w1056) -> (x > 0?=w1055:bool)
                                n1929 = local write "GPIB bus 2 traffic"(w1059) -> ()
                                n1930 = And(x=w1053, y=w1055) -> (x .and. y?=w1051:bool)
                                n1931 = Or(x=w1051, y=w1049) -> (x .or. y?=w1050:bool)
                                }
                                }
                                }
                                }
                                frame #1 {
                                n1932 = case shown="True" w1067 {
                                tunnel: w1068 -> [w1069 _]
                                frame False {
                                n1933 = flat-sequence {
                                tunnel: w1069 -> [w1070]
                                frame #0 {
                                n1934 = String Length(string=w1070) -> (length=w1071:i32)
                                n1935 = local write "H2 sites ready hidden"(w1070) -> ()
                                n1936 = local write "H2 parallelism"(w1071) -> ()
                                }
                                frame #1 {
                                # "This block adds zeroes (sites not ready)\nto SITES READY from handlers when the\nhandler is running at a lower parallelism\nthan the test program, but has the same\npin mapping for the active sites in common."
                                n1937 = local read "Program Parallelism"() -> (w1073:u32)
                                n1938 = local read "H2 allow lower parallelism"() -> (w1074:bool)
                                n1939 = local read "H2 parallelism"() -> (w1072:u32)
                                n1940 = Less?(x=w1072, y=w1073) -> (x < y?=w1075:bool)
                                n1941 = And(x=w1075, y=w1074) -> (x .and. y?=w1076:bool)
                                n1942 = case shown="False" w1076 {
                                frame False {
                                n1943 = local read "Program Parallelism"() -> (w1079:u32)
                                n1944 = local read "H2 parallelism"() -> (w1077:u32)
                                n1945 = Greater?(x=w1077, y=w1079) -> (0:w1078:bool)
                                n1946 = case shown="True" w1078 {
                                frame False {
                                # "parallelisms must match if arriving here"
                                n1947 = local write "SC virtual tester 2 states"(SC_virtual_tester_states."sending HAND?" ("SC virtual tester states")) -> ()
                                }
                                frame True {
                                n1948 = local write "POWER"(FALSE ("POWER")) -> ()
                                n1949 = local write "SC virtual tester 2 states"(SC_virtual_tester_states."closing bus" ("SC virtual tester states")) -> ()
                                n1950 = One Button Dialog(message="Fatal error 301:\nTest program cannot support higher\nparallelism on handler 2.\nThe Sentinel Controller program is shutting down.\nPlease correct the mismatch and restart.") -> ()  [unwired: 1 in, 1 out]
                                }
                                }
                                }
                                frame True {
                                n1951 = local read "Program Parallelism"() -> (w1089:u32)
                                n1952 = local read "H2 parallelism"() -> (w1087:u32)
                                n1953 = local read "H2 sites ready hidden"() -> (w1085:string)
                                n1954 = Subtract(x=w1089, y=w1087) -> (x-y=w1088:u32)
                                n1955 = local write "SC virtual tester 2 states"(SC_virtual_tester_states."sending HAND?" ("SC virtual tester states")) -> ()
                                n1956 = for {
                                N: w1088 -> [_]
                                shift-right: [w1090] -> w1084
                                shift-left: w1085 -> [w1091]
                                n1957 = Concatenate Strings(w1091, "0" ("string")) -> (w1090:string)
                                }
                                n1958 = local write "H2 sites ready hidden"(w1084) -> ()
                                }
                                }
                                }
                                frame #2 {
                                n1959 = Tick Count (ms)() -> (millisecond timer value=w1097:u32)
                                n1960 = Tick Count (ms)() -> (millisecond timer value=w1096:u32)
                                n1961 = local write "H2 Ready with sites"(TRUE ("H2 Waiting")) -> ()
                                n1962 = local write "H2 Indexing"(FALSE ("h1 indexing")) -> ()
                                n1963 = local write "H2 Testing"(FALSE ("h1 indexing")) -> ()
                                n1964 = local write "H2 wt start hidden"(w1097) -> ()
                                n1965 = local write "H2 it end hidden"(w1096) -> ()
                                }
                                frame #3 {
                                n1966 = local read "H2 it start hidden"() -> (w1101:u32)
                                n1967 = local read "H2 it end hidden"() -> (w1102:u32)
                                n1968 = Subtract(x=w1102, y=w1101) -> (x-y=w1098:u32)
                                n1969 = local write "SC virtual tester 2 states"(SC_virtual_tester_states."sending HAND?" ("SC virtual tester states")) -> ()
                                n1970 = Divide(x=w1098, y=u32 1000) -> (x/y=w1100:dbl)
                                n1971 = local write "H2 measured  Index Time"(w1100) -> ()
                                }
                                }
                                }
                                frame True {
                                n1972 = flat-sequence {
                                frame #0 {
                                n1973 = local read "VISA bus 2 resource name out"() -> (w1107:refnum<visa-resource-name>)
                                n1974 = local read "VISA bus 2 error out"() -> (w1106:errorcluster)
                                n1975 = VISA Close(VISA resource name=w1107, error in (no error)=w1106) -> (error out=w1105:errorcluster)
                                n1976 = Unbundle By Name(w1105) -> ("status"=w1104:bool)
                                n1977 = local write "VISA bus 2 close error"(w1104) -> ()
                                }
                                frame #1 {
                                n1978 = local write "VISA bus 2 close error"(FALSE ("VISA bus 1 close error")) -> ()
                                n1979 = Concatenate Strings("Bus 2 error  while reading,\nclosing Bus 2 and re-initializing" ("string"), "\r\n") -> (w1109:string)
                                n1980 = local write "GPIB bus 2 traffic"(w1109) -> ()
                                }
                                frame #2 {
                                n1981 = local write "SC virtual tester 2 states"(SC_virtual_tester_states."initializing bus" ("SC virtual tester states")) -> ()
                                }
                                }
                                }
                                }
                                }
                                }
                              }
                              frame "sending HAND?" {
                                n1982 = flat-sequence {
                                tunnel: [w1116] -> w1114
                                tunnel: [w1115] -> w1113
                                tunnel: w1114 -> [w1126]
                                tunnel: w1113 -> [w1125]
                                frame #0 {
                                w1124 = "*HAND?"
                                n1983 = local read "VISA bus 2 resource name out"() -> (w1117:refnum<visa-resource-name>)
                                n1984 = local read "GPIB bus 2 traffic"() -> (w1120:string)
                                n1985 = local read "VISA bus 2 error out"() -> (w1118:errorcluster)
                                n1986 = Concatenate Strings(w1120, "\r\n", "Bus 2 write: " ("string"), w1124) -> (w1122:string)
                                n1987 = VISA Write(VISA resource name=w1117, write buffer=w1124, error in (no error)=w1118) -> (VISA resource name out=w1116:refnum<visa-resource-name>, error out=w1115:errorcluster)  [unwired: 1 out]
                                n1988 = local write "GPIB bus 2 traffic"(w1122) -> ()
                                n1989 = Unbundle By Name(w1115) -> ("status"=w1119:bool)
                                n1990 = local write "GPIB bus 2 write error"(w1119) -> ()
                                }
                                frame #1 {
                                n1991 = local read "GPIB bus 2 traffic"() -> (w1128:string)
                                n1992 = VISA Read(VISA resource name=w1126, byte count=u32 256, error in (no error)=w1125) -> (read buffer=w1127:string, error out=w1133:errorcluster)  [unwired: 2 out]
                                n1993 = local write "H2 response to *HAND? hidden"(w1127) -> ()
                                n1994 = Unbundle By Name(w1133) -> ("status"=w1132:bool)
                                n1995 = local write "GPIB bus 2 read error"(w1132) -> ()
                                n1996 = Concatenate Strings(w1128, "\r\n", "Bus 2 read: " ("string"), w1127) -> (w1130:string)
                                n1997 = local write "GPIB bus 2 traffic"(w1130) -> ()
                                }
                                frame #2 {
                                n1998 = local write "SC virtual tester 2 states"(SC_virtual_tester_states."testing" ("SC virtual tester states")) -> ()
                                }
                                }
                              }
                              frame "testing" {
                                n1999 = flat-sequence {
                                frame #0 {
                                n2000 = while {
                                stop <- w1136 stop-if-true
                                n2001 = local read "H2 Lock"() -> (w1136:bool)
                                n2002 = Wait (ms)(milliseconds to wait=u32 1) -> ()  [unwired: 1 out]
                                }
                                }
                                frame #1 {
                                n2003 = Tick Count (ms)() -> (millisecond timer value=w1148:u32)
                                n2004 = Tick Count (ms)() -> (millisecond timer value=w1147:u32)
                                n2005 = local write "H2 Ready with sites"(FALSE ("waiting")) -> ()
                                n2006 = local write "H2 Indexing"(FALSE ("waiting")) -> ()
                                n2007 = local write "H2 Testing"(TRUE ("testing")) -> ()
                                n2008 = local write "H2 wt end hidden"(w1148) -> ()
                                n2009 = local write "H2 tt start hidden"(w1147) -> ()
                                n2010 = local read "GPIB bus 2 traffic"() -> (w1139:string)
                                n2011 = local write "SC virtual tester 2 states"(SC_virtual_tester_states."binning" ("SC virtual tester states")) -> ()
                                n2012 = Concatenate Strings(w1139, "\r\n", "Bus 2: " ("string"), "testing" ("string")) -> (w1141:string)
                                n2013 = local write "GPIB bus 2 traffic"(w1141) -> ()
                                }
                                frame #2 {
                                n2014 = local read "H2 wt start hidden"() -> (w1150:u32)
                                n2015 = local read "H2 wt end hidden"() -> (w1149:u32)
                                n2016 = Subtract(x=w1149, y=w1150) -> (x-y=w1153:u32)
                                n2017 = Divide(x=w1153, y=u32 1000) -> (x/y=w1151:dbl)
                                n2018 = local write "H2 measured Wait Time"(w1151) -> ()
                                }
                                }
                              }
                              frame "binning" {
                                n2019 = flat-sequence {
                                tunnel: [w1165] -> w1156
                                tunnel: [w1192] -> w1157
                                tunnel: w1156 -> [w1192]
                                tunnel: w1157 -> [w1199]
                                tunnel: [w1198] -> w1155
                                tunnel: [w1197] -> w1154
                                tunnel: w1155 -> [w1250]
                                tunnel: w1154 -> [w1249]
                                frame #0 {
                                n2020 = while {
                                stop <- w1159 continue-if-true
                                n2021 = local read "H2 Lock"() -> (w1159:bool)
                                n2022 = Wait (ms)(milliseconds to wait=u32 1) -> ()  [unwired: 1 out]
                                }
                                }
                                frame #1 {
                                n2023 = local read "Program Parallelism"() -> (w1162:u32)
                                n2024 = local read "H2 parallelism"() -> (w1161:u32)
                                n2025 = local read "H2 allow lower parallelism"() -> (w1163:bool)
                                n2026 = Less?(x=w1161, y=w1162) -> (x < y?=w1164:bool)
                                n2027 = And(x=w1164, y=w1163) -> (x .and. y?=w1160:bool)
                                n2028 = case shown="True" w1160 {
                                tunnel: [w1166 w1177] -> w1165
                                frame False {
                                n2029 = local read "VISA bus 2 resource name out"() -> (w1174:refnum<visa-resource-name>)
                                n2030 = local read "Binning_string hidden"() -> (w1166:string)
                                n2031 = local read "VISA bus 2 error out"() -> (w1175:errorcluster)
                                n2032 = local read "GPIB bus 2 traffic"() -> (w1170:string)
                                n2033 = VISA Write(VISA resource name=w1174, write buffer=w1166, error in (no error)=w1175) -> (VISA resource name out=w1172:refnum<visa-resource-name>, error out=w1173:errorcluster)  [unwired: 1 out]
                                n2034 = local write "VISA bus 2 resource name out"(w1172) -> ()
                                n2035 = local write "VISA bus 2 error out"(w1173) -> ()
                                n2036 = Unbundle By Name(w1173) -> ("status"=w1171:bool)
                                n2037 = Concatenate Strings(w1170, "\r\n", "Bus 2 write: " ("string"), w1166) -> (w1168:string)
                                n2038 = local write "GPIB bus 2 write error"(w1171) -> ()
                                n2039 = local write "GPIB bus 2 traffic"(w1168) -> ()
                                }
                                frame True {
                                n2040 = local read "H2 parallelism"() -> (w1176:u32)
                                n2041 = local read "Binning_string hidden"() -> (w1178:string)
                                n2042 = local read "VISA bus 2 resource name out"() -> (w1189:refnum<visa-resource-name>)
                                n2043 = Multiply(x=w1176, y=u32 8) -> (x*y=w1180:u32)
                                n2044 = local read "VISA bus 2 error out"() -> (w1190:errorcluster)
                                n2045 = local read "GPIB bus 2 traffic"() -> (w1185:string)
                                n2046 = Decrement(x=w1180) -> (x-1=w1181:u32)
                                n2047 = String Subset(string=w1178, length (rest)=w1181) -> (substring=w1177:string)  [unwired: 1 in]
                                n2048 = VISA Write(VISA resource name=w1189, write buffer=w1177, error in (no error)=w1190) -> (VISA resource name out=w1187:refnum<visa-resource-name>, error out=w1188:errorcluster)  [unwired: 1 out]
                                n2049 = local write "VISA bus 2 resource name out"(w1187) -> ()
                                n2050 = local write "VISA bus 2 error out"(w1188) -> ()
                                n2051 = Unbundle By Name(w1188) -> ("status"=w1186:bool)
                                n2052 = Concatenate Strings(w1185, "\r\n", "Bus 2 write: " ("string"), w1177) -> (w1183:string)
                                n2053 = local write "GPIB bus 2 traffic"(w1183) -> ()
                                n2054 = local write "GPIB bus 2 write error"(w1186) -> ()
                                }
                                }
                                }
                                frame #2 {
                                n2055 = Tick Count (ms)() -> (millisecond timer value=w1194:u32)
                                n2056 = Tick Count (ms)() -> (millisecond timer value=w1193:u32)
                                n2057 = local write "H2 Ready with sites"(FALSE ("waiting")) -> ()
                                n2058 = local write "H2 Testing"(FALSE ("waiting")) -> ()
                                n2059 = local write "H2 Indexing"(TRUE ("waiting")) -> ()
                                n2060 = local write "H2 it start hidden"(w1194) -> ()
                                n2061 = local write "H2 tt end hidden"(w1193) -> ()
                                }
                                frame #3 {
                                n2062 = while {
                                tunnel: [w1222] -> w1218 mode=indexing
                                shift-right: [w1223] -> _
                                shift-left: w1199 -> [w1225]
                                stop <- w1220 stop-if-true
                                n2063 = Match Pattern(string=w1225, regular expression=" ") -> (before substring=w1222:string, after substring=w1223:string, offset past match=w1221:i32)  [unwired: 2 out]
                                n2064 = Less Than 0?(x=w1221) -> (x < 0?=w1220:bool)
                                }
                                n2065 = local read "H2 tt start hidden"() -> (w1203:u32)
                                n2066 = local read "H2 tt end hidden"() -> (w1204:u32)
                                n2067 = Subtract(x=w1204, y=w1203) -> (x-y=w1202:u32)
                                n2068 = Divide(x=w1202, y=u32 1000) -> (x/y=w1200:dbl)
                                n2069 = local read "H2 sites ready hidden"() -> (w1210:string)
                                n2070 = Array Size(array=w1218) -> (size(s)=w1215:i32)
                                n2071 = local read "H2 parallelism"() -> (w1209:u32)
                                n2072 = local write "H2 measured Test Time"(w1200) -> ()
                                n2073 = Divide(x=w1215, y=3) -> (x/y=w1217:dbl)
                                n2074 = To Unsigned Byte Integer(number=w1217) -> (unsigned 8bit integer=w1213:u8)
                                n2075 = Not Equal?(x=w1209, y=w1213) -> (x != y?=w1214:bool)
                                n2076 = case shown="True" w1214 {
                                frame False {
                                }
                                frame True {
                                n2077 = One Button Dialog(message="Warning:\nH2 Parallelism Mismatch!\nEither allow this from the system configuration tab\nor change the parallelism on H2. This message will\ncontinue until the problem is corrected.") -> ()  [unwired: 1 in, 1 out]
                                }
                                }
                                n2078 = for {
                                N: w1213 -> [_]
                                tunnel: w1218 -> [w1248]
                                tunnel: w1210 -> [w1239]
                                shift-right: [w1232] -> w1197
                                shift-left: 0 -> [w1231]
                                shift-right: [w1228] -> w1198
                                shift-left: 0 -> [w1226]
                                i -> [w1229]
                                n2079 = Increment(x=w1226) -> (x+1=w1227:i32)
                                n2080 = Increment(x=w1231) -> (x+1=w1230:i32)
                                n2081 = Increment(x=w1229) -> (x+1=w1247:i32)
                                n2082 = String Subset(string=w1239, offset (0)=w1229, length (rest)=1 ("length (rest)")) -> (substring=w1235:string)
                                n2083 = Multiply(x=3, y=w1247) -> (x*y=w1241:i32)
                                n2084 = Equal?(x=w1235, y="1") -> (x = y?=w1233:bool)
                                n2085 = Select(t=w1230, s=w1233, f=w1231) -> (s? t:f=w1232:i32)
                                n2086 = Decrement(x=w1241) -> (x-1=w1240:i32)
                                n2087 = Index Array(array=w1248, index=w1240) -> (element=w1245:string)
                                n2088 = Decimal String To Number(string=w1245, offset=0) -> (number=w1243:i32)  [unwired: 1 in, 1 out]
                                n2089 = Equal?(x=w1243, y=1) -> (x = y?=w1236:bool)
                                n2090 = And(x=w1236, y=w1233) -> (x .and. y?=w1237:bool)
                                n2091 = Select(t=w1227, s=w1237, f=w1226) -> (s? t:f=w1228:i32)
                                }
                                n2092 = local read "H2 Device Count"() -> (w1206:u32)
                                n2093 = local read "H2 Good Units"() -> (w1207:u32)
                                n2094 = Add(x=w1207, y=w1198) -> (x+y=w1208:u32)
                                n2095 = Add(x=w1206, y=w1197) -> (x+y=w1205:u32)
                                n2096 = local write "H2 Good Units"(w1208) -> ()
                                n2097 = local write "H2 Device Count"(w1205) -> ()
                                }
                                frame #4 {
                                n2098 = local read "H2 Device Count"() -> (w1254:u32)
                                n2099 = local read "H2 Good Units"() -> (w1255:u32)
                                n2100 = Divide(x=w1250, y=w1249) -> (x/y=w1251:dbl)
                                n2101 = Multiply(x=w1251, y=100.0) -> (x*y=w1253:dbl)
                                n2102 = local write "H2 cycle yield hid"(w1253) -> ()
                                n2103 = Divide(x=w1255, y=w1254) -> (x/y=w1258:dbl)
                                n2104 = Multiply(x=w1258, y=100.0) -> (x*y=w1256:dbl)
                                n2105 = local write "H2 lot yield mon"(w1256) -> ()
                                }
                                frame #5 {
                                n2106 = local read "H2 online"() -> (w1259:bool)
                                n2107 = local read "POWER"() -> (w1261:bool)
                                n2108 = Compound Arithmetic op=AND(w1259, w1261) -> (w1260:bool)
                                n2109 = case shown="False" w1260 {
                                frame False {
                                n2110 = local write "SC virtual tester 2 states"(SC_virtual_tester_states."closing bus" ("SC virtual tester states")) -> ()
                                }
                                frame True {
                                n2111 = local write "SC virtual tester 2 states"(SC_virtual_tester_states."sending *IDN?" ("SC virtual tester states")) -> ()
                                }
                                }
                                }
                                }
                              }
                              frame "closing bus" {
                                n2112 = local read "GPIB bus 2 traffic"() -> (w1268:string)
                                n2113 = local write "Exit virtual tester H2 state machine hid"(TRUE ("Exit H2 state machine hid")) -> ()
                                n2114 = local read "VISA bus 2 resource name out"() -> (w1272:refnum<visa-resource-name>)
                                n2115 = local read "VISA bus 2 error out"() -> (w1271:errorcluster)
                                n2116 = Concatenate Strings(w1268, "\r\n", "Bus 2: closing " ("string")) -> (w1266:string)
                                n2117 = local write "GPIB bus 2 traffic"(w1266) -> ()
                                n2118 = VISA Close(VISA resource name=w1272, error in (no error)=w1271) -> (error out=w1270:errorcluster)
                                n2119 = Unbundle By Name(w1270) -> ("status"=w1269:bool)
                                n2120 = local write "VISA bus 2 close error"(w1269) -> ()
                              }
                            }
                          }
                          frame #1 {
                            n2121 = local read "Slow for  Diagnostics"() -> (w1273:bool)
                            n2122 = case shown="True" w1273 {
                              frame False {
                              }
                              frame True {
                                n2123 = local read "GPIB wait time (ms)"() -> (w1274:u32)
                                n2124 = Wait (ms)(milliseconds to wait=w1274) -> ()  [unwired: 1 out]
                              }
                            }
                          }
                        }
                        n2125 = Wait (ms)(milliseconds to wait=u32 1) -> ()  [unwired: 1 out]
                        n2126 = local read "Exit virtual tester H2 state machine hid"() -> (w981:bool)
                      }
                    }
                  }
                }
              }
              n2127 = Wait (ms)(milliseconds to wait=u32 5) -> ()  [unwired: 1 out]
              n2128 = local read "POWER"() -> (w976:bool)
            }
          }
        }
      }
    }
  }
